vi "Core_Chem_User_Interface_v3.0.vi"() -> ()   [LabVIEW 2014]
uses:
  C:/Program Files (x86)/National Instruments/LabVIEW 2014/examples/Data Communication/Network Streams/Simple Network Streams/support/Network Stream Command.ctl
  <vilib>/dex/Stream Element Allocation Mode.ctl
  <vilib>/Platform/TimedLoop/XDataNode/timing_clust.ctl
  <vilib>/Platform/TimedLoop/XDataNode/nitl_modes.ctl
  <vilib>/Platform/TimedLoop/XDataNode/wakeup.ctl
  <vilib>/Utility/tcp.llb/UDP Multicast Read-Only Open.vi
  <vilib>/platform/TimedLoop/XDataNode/XDataNode.xnode
  <vilib>/Platform/TimedLoop/XDataNode/XDNodeRunTimeDep.lvlib
  <vilib>/FTP/NI_FTP.lvlib
panel:
  out "Network disconnected":bool
  out "cRIO connection status":bool
  out "Network Check error out":errorcluster
  out "SO2 Zeroing (Inflight)\nTime Remain (sec)":u32
  in  "eV6 User set time \n(Inflight) (sec)":i32=120
  in  "SO2 Inflight \nZeroing":bool
  out "Create folder error out 2":errorcluster
  out "Create folder error out":errorcluster
  in  "Confirm Flight Number":bool
  out "PRTAFT_UDP_In":string
  out "TWBOZO01":string
  out "CABOZO01":string
  out "TEIOZO01":string
  out "CHTSOO01":string
  out "CHFGGA01":string
  out "AL52CO01":string
  in  "Flight Number":string
  in  "Tab Control":T1(tab)
  out "FGGA preflight Des 17":string="Preflight - Start minimum 2 hours before take-off\n\n1. Ensure no bags/jackets are stowed on seat backs and behind seats in front of core chemistry rack at all times.\n\n2. Remove inlet covers if applicable.\n\n3. Connect Lilliput mini TFT/LCD VGA cable to FGGA VIDEO (back panel) and PS2 Keyboard/Mouse cables to FGGA Connectors (back panel). TFT/LCD screen kept in WAS/GAS rack Zargers Box. Keyboard/Mouse kept bottom of chemistry rack. (DO NOT disconnect PS2 cable). Connect TFT/LCD AC/DC PSU to 6026-8-98 Amphenol (SSP9) and make 230 Vac CB.\n\n4. Ensure all circuit breakers are pushed in, except 230Vac and 28Vdc, UPS switch off (down) and AL5002 CO Plasma Lamp switch off (down), WoW key to normal (horizontal).\n\n5. Wait for ALL network switches on the aircraft to be up and running before start-up. On the Flight Manager's Interface on the Flight Manager laptop, check SSP icons status (top row) should be all green.  \n\n6. Check AboutTime has synchronised laptop clock to aircraft timeservers (Filiberto/Gaston).\n\nClick the PowerUp Tab."
  out "FGGA preflight Des 16":string="PowerUp\n\n1.\tSSP9 forward face\tMake 3 CBs\n\n2.\tPWRDIST \t\tMake 230Vac CB \n                     Switch UPS On \t[UP]\n                     Make 28Vdc CB\n                     Check 28VDC OK Green Light comes on\n\n3.\tCore Chemistry e-Log\nComplete Core Chemistry e-Log in WordPad (Bnnn_CoreChemLog_v2.2), save on Flight Manager's laptop (192.168.101.180/      flt_folders/Bnnn); Fill in header with date, flight number and your name/initials.\n\n4. Wait for MFM flow rate to display non zero value.\n\n5.\tSAMPUMP\t\t\n - Switch WoW override key (vertical) to check pump starts, and MFM flowrate increase (>20 LPM) on the right hand plot. \n - Switch off WoW override\t\t\t\t [NORM, key horizontal]\n\nClick the 2B Ozone tab if operated, otherwise, click the UDP tab.\n\n\n"
  out "MFM":dbl(graph)
  in  "Ambient = OFF\nCabin = ON":bool
  out "FGGA preflight Des 15":string="2B Ozone Preflight\n\n1.\tSelect either Ambient or Cabin Air mode (default should be OFF for Ambient air mode).\n\n2. Check flowrate is greater than 2000 sccm on the right hand plot.\n\nClick the UDP tab."
  out "2B Ozone concentration":dbl(graph)
  out "2B Ozone flow rate":dbl(graph)
  out "2BOzone Event error out":errorcluster
  out "2BOzone command sender error out":errorcluster
  out "FGGA preflight Des 20":string="4. Check derived parameters in DECADES (192.168.101.110 & 192.168.101.108). 574 Ozone TEi49C; 588 CO AL5002; 611 SO2 TEi43i; 903 - 905 FGGA; 910 / 920 Ozone 2B."
  out "FGGA preflight Des 14":string="UDP Preflight\n1. Check all UDP packets are updating.  Unix time increasing by 1 sec (3rd parameter).\n2. Check flight number is correct.\n3. Confirm flight number and check it appears in the UDP packet (6th parameter). "
  in  "name":string="239.1.4.6"
  in  "Port":u16=50001
  out "FGGA":string
  out "CO":string
  out "TEi49 Ozone":string
  out "2B Cabin Ozone":string
  out "2B Ambient Ozone":string
  out "SO2":string
  in  "Ozone Zeroing Abort":bool
  out "Ozone Zeroing\nTime Remain (sec)":u32
  in  "Ozone Zeroing":bool
  out "TEI49 Sample Flow B":dbl(graph)
  out "TEi49 Concentration":dbl(graph)
  out "TEI49 Sample Flow A":dbl(graph)
  out "FGGA preflight Des 13":string="TEi49 Ozone PRE-FLIGHT - LAST ACTIONS BEFORE SEAT-BELTING DOWN (PRIOR TO ENGINES START)\n\n1. Ozone monitor zeroing\t\t[10 min minimum]\n\n\n2. Check TEi49 zero value and note down value in e-Log. \n"
  out "FGGA preflight Des 12":string="TEi49 Ozone Preflight\n\n1. Check nominal sample flowrate on both channels is ~0.7 LPM."
  out "Ozone Event error out":errorcluster
  out "Ozone command sender error out":errorcluster
  in  "Ozone UDP Time Offset":i32=1
  in  "SO2 Zeroing / Calibration Abort":bool
  out "SO2 react pressure":dbl(graph)
  in  "Prepare SO2 Zero Gas":bool
  in  "Prepare SO2 Span Gas":bool
  in  "Auto Zeroing \ninterval (sec)":i32=600
  out "Next Auto Zero\nStarts in (sec)":u32
  out "Auto Zero\nIndicator":string="Auto Zero Inactive; Manual Zero Allow"
  out "SO2 Resume Zeroing\nCount down timer (sec)":u32
  in  "SO2 Pause\nAuto Zeroing":bool
  out "TEi43i Concentration scaled / raw":cluster{dbl, dbl}(graph)
  in  "SO2 Auto Zeroing":bool
  out "mean zero\ncal status":bool
  out "SO2 Sensitivity":dbl format="%.2g"
  out "SO2 Zero":dbl format="%.2g"
  in  "eV9 Flush User\nset time (sec)":i32=15
  in  "MFC_3 User Set Value":dbl=2.0
  in  "MFC_2 User Set Value":dbl=2.5
  in  "eV6 User\nset time (sec)":i32=600
  out "SO2 Flush\nTime Remain (sec)":u32
  out "TEI43i MFC3 Sample Flow":dbl(graph)
  out "TEI43C Sample Flow":dbl(graph)
  out "TEI43i MFC2 Cal Flow":dbl(graph)
  out "SO2 CAL/Zero\nTime Remain (sec)":u32
  out "SO2 Cal/Zero Flush\nTime Remain (sec)":u32
  in  "SO2 CAL/Zero":bool
  out "FGGA preflight Des 11":string="TEi43 SO2 Inflight Calibration & Zeroing"
  in  "SO2 GND Zeroing":bool
  out "SO2 Zeroing\nTime Remain (sec)":u32
  out "FGGA preflight Des 10":string="TEi43 SO2 PRE-FLIGHT - LAST ACTIONS BEFORE SEAT-BELTING DOWN (PRIOR TO ENGINES START)\n\n1. SO2 monitors zeroing\t\t[10 min minimum]\n\n2. Check TEi43i or TEi43C zero value and note down value in e-Log.\n\n3. Select required SO2 Span/Zero CAL gas at CALDECK front panel using quick connector.\n    For pre- and post-flight SO2 span calibrations select span gas. - Perform SO2 CAL\n    For in-flight SO2 (auto) zeroing, select zero air gas.\n\n4. Enable SO2 auto zeroing (if required) and check zeroing interval. "
  in  "SO2 Flush":bool
  out "FGGA preflight Des 9":string="TEi43 SO2 Preflight\n\n1. Check nominal sample flowrate is 2.0 LPM on the right hand plot.\n\nSO2 calibration gas purge - SO2 calibration cylinder locate at bottom of WAS Gas rack.\n\n2.\n\n\n3. Press SO2 flush button, MFC2 cal flow should increase to 2.5 SLPM.\nMonitor MFC2 flow rate to make sure the reading decreases from 2.5 SLPM to 0.0 SLPM.\nCheck pressure content and delivery gauges also reads zero.\nIf pressure content & delivery gauges do NOT read zero, press SO2 flush button again until they do.\n\n4. Quickly open and close cylinder valve 1.\n\n5. Repeat step 3) to 4) three times.\n\n6. Open cylinder valve 1, system is ready. Note down content pressure in elog.\n\n7."
  in  "eV9 flush User\nset time (sec)":i32=30
  in  "eV8 User\nset time (sec)":i32=60
  out "SO2 Event error out":errorcluster
  out "SO2 command sender \nerror out":errorcluster
  in  "SO2 UDP Time Offset":i32=1
  out "Lamp Temperature":dbl(graph)
  out "CO CAL Status":bool
  in  "CO CAL":bool
  out "FGGA preflight Des 8":string="CO Preflight and Inflight Calibrations\nHold down the CAL button for 2 secs then release, CAL status should then lit up.\nInflight calibration performed on 45 minutes interval or more frequently if lamp temperature > 35.5 degC."
  in  "Prepare Gases":bool
  out "FGGA preflight Des 7":string="AL5002 CO Preflight Checks\n\n1.\n\n2. Start CO Vacuum. NB: If there is problem with the software control, use manual override switch [up] on CALDECK front panel\n\n3. CO Checks - charts on the right hand side\n    Lamp Flow Controller ~ 40 ml/min\n    Monochromator Flow Controller ~ 30 ml/min\n    Fluorescence Cell Pressure ~ 7.5 Torr\n\nIf Lamp/Mono flows are low, manual valves (V1 -> V5) may still be shut, or pressure adjusting valves (ALREG1 & 2) have not been set > 2 bar\n\nIf Cell pressure is 10 Torr (max range), check that COPUMP is running and eV7 is opened (CO Vacuum eV7 is ON).\n\n4. Switch Plasma Lamp at the front panel UP\n\nDetector count rate (on 'Raw Signal' or F2 instrument touchscreen) should increase to >=10000 Hz within a minute.  Recycle plasma lamp switch (off/on) if no significant increase in count rate after 10 mins.  CO concentration should increase (100s ppb). \n     \n\n"
  in  "CO Vaccum (eV7)":bool
  out "Raw Signal":dbl(graph)
  out "CO Concentration":dbl(graph)
  out "Fluorescence Cell Pressure":dbl(graph)
  out "Monochromator Flow":dbl(graph)
  out "Lamp Flow Controller":dbl(graph)
  in  "CO UDP Time Offset":i32=1
  out "CO2 Pressure\nDelivery (PSIA)":dbl(slide) scale=0.0..100.0
  out "Std\nContent (barG)":dbl(slide) scale=0.0..220.0
  out "N2\nContent (barG)":dbl(slide) scale=0.0..220.0
  out "CO2\nContent (barG)":dbl(slide) scale=0.0..170.0
  out "CO Event error out":errorcluster
  out "CO command sender error out":errorcluster
  out "CO Zero":T2(array[cluster])
  out "CO Sensitivity":T3(array[cluster])
  in  "FGGA Calibration Abort":bool
  out "Ring Down Time RDA & RDB":cluster{dbl, dbl}(graph)
  in  "Line Lock Setting Change":bool
  out "Cell temperature":dbl(graph)
  out "Cell pressure":dbl(graph)
  in  "Manual FGGA Pump":bool
  out "CO2":dbl(graph)
  out "CH4":dbl(graph)
  out "H2O":dbl(graph)
  out "WoW Flag":string="0"
  in  "FGGA pump\nsync to WoW":bool
  out "CH4 Dry":dbl(graph)
  out "CO2 Dry":dbl(graph)
  out "MFC1 Cal Flow":dbl(graph)
  out "Flush Target Tank\nTime Remain (sec)":u32
  out "Flush Low Tank\nTime Remain (sec)":u32
  out "Flush High Tank\nTime Remain (sec)":u32
  in  "Flush Target Tank":bool
  in  "Flush Low Tank":bool
  in  "Flush High Tank":bool
  in  "FGGA Restart":bool
  out "FGGA preflight Des 6":string="FGGA Instrument Controls"
  in  "High Cal":bool
  out "High Cal\nFlush Time Remain (sec)":u32
  out "High Cal\nCal Time Remain (sec)":u32
  in  "Low Cal":bool
  in  "Target Cal":bool
  in  "Span Cal - \nHigh Cal, CO Cal, Low Cal":bool
  out "Low Cal\nFlush Time Remain (sec)":u32
  out "Low Cal\nCal Time Remain (sec)":u32
  out "Target Cal\nFlush Time Remain (sec)":u32
  out "Target Cal\nCal Time Remain (sec)":u32
  in  "MFC_1 User Set Value":dbl=2.0
  out "FGGA preflight Des 5":string="FGGA Inflight Calibrations"
  out "FGGA preflight Des 4":string="FGGA Ground Preflight Checks\n\n1. Switch FGGA pump ON\n\n2. Check cavity pressure ~50 Torr\n\n3. Switch FGGA pump OFF\n\n4. Enable FGGA pump sync to WoW\n\n5.. Check Time Synchronisation\n\n6. Check CO2 & CH4 values\n\nIf CO2 & CH4 values are -1 ppm, follow the \nchange linelock settings procedure.\n\n\n\n\n\nLAST ACTION BEFORE SEAT-BELTING \nDOWN (PRIOR TO ENGINES START)\n\n1. Disconnect Monitor & stow away. Leave Keyboard & Mouse connected. Place keyboard at the bottom\nof the rack.\n\n"
  out "FGGA preflight Des 3":string="FGGA CAL Gas Purge\n\nFor each cylinder in gas stowage, check that,\n\n1. V1 Closed\n    V3 Closed\n    V4 Make sure arrow positioned downwards (i.e. flow points to gas line)\n\n2. V3 Open (turn anti-clockwise)\n\n3. Use the button on the right according to the operating cylinder to flush the line. Monitor the MFC flow rate to make sure the reading decreases from 3 to zero. (ie fully flushed). Pressure content & delivery gauges should also read zero.\n\n4. V3 Close (turn clockwise)\n\n5. V1 Open / Close quickly\n         Check delivery pressure gauge is ~ 40 PSI \n         (Use V2 to increase if necessary)\n\n6. Repeat steps 2) to 5) three times\n\n7. V3 Close (turn clockwise)\n\n8. V1 Open, check V2 ~ 40 PSIG\n\n9. V3 Open - System is ready"
  out "FGGA command sender error out":errorcluster
  out "FGGA Event Error out":errorcluster
  in  "FGGA UDP Time Offset":i32=1
  in  "FGGA Shutdown":bool
  in  "Postflight Procedures":bool
  in  "FTP ASCII Files to Local":bool
  in  "Transfer FGGA Files":bool
  out "FGGA preflight Des 18":string="Postflight\n\n1. Press the FTP ASCII File to Local button to transfer ASCII files to flight folder.\n\n\n2. Press the Transfer FGGA Files button to transfer FGGA files to flight folder. \n\n\n3. Shutdown FGGA.\n\n\n4. View Postflight Procedures."
  out "File List":string[](array[string])
  out "FGGA File Transfer Error out":errorcluster
  out "Move to FM Error out":errorcluster
  out "USB Disk Space Used %":dbl(slide) scale=0.0..100.0
  out "PTP Sync":bool
  out "CPU Total %":dbl(graph)
  out "PRTAFT_DLU":string
  in  "Pause Auto Zero Count \nDown set time (sec)":i32=600
  out "Calibration gas cylinder \nconcentration (ppb)":dbl format="%.4g"
  in  "Save Calibration gas\ncylinder concentration to file":bool
  in  "Calibration gas cylinder \nconcentration (ppb)":dbl=500.0 format="%.4g"
  in  "Simulate MOCCA Conc":dbl
  in  "MOCCA window \ndelay time (sec)":i32=30
  in  "MOCCA Limit":i32=800
  in  "SO2 Inflight MOCCA Alarm\n(default = OFF)":bool
  in  "Offset Mean Zero Calculation (default = ON)\nOFF = User input\nOn = Mean zero calculated with ev8":bool=TRUE
  out "FGGA preflight Des 19":string="This tab controls ONLY for advanced operators."
  in  "Inst_alm_thresh":i32=220
  in  "3hr_alm_thresh":i32=80
  in  "Simulate Inst Conc":i32
  in  "Simulate 3hr Average Conc":dbl
  in  "Simulate 2B Conc":bool
  in  "Ozone eV6":bool
  in  "Simulate Conc":bool
  in  "8hr TWA Limit":i32=490
  in  "10mins STEL Limit":i32=800
  in  "SO2 Sensitivity":dbl=1.1
  in  "SO2 Zero":dbl
  in  "Simulate TWA Conc":dbl
  in  "Simulate STEL Conc":dbl
  in  "MFC_3\nSLPM Value":dbl=2.0
  in  "MFC_2\nSLPM Value":dbl
  in  "SO2 eV6":bool
  in  "eV8":bool
  in  "eV9":bool
  in  "eV4":bool
  in  "eV3":bool
  in  "MFC_1\nSLPM Value":dbl
  in  "eV2":bool
  in  "eV1":bool
  in  "cRIO File IO Stop\n(USB Flash Drive Unmount)":bool
  # "Unix time"
  # "Flight Number"
  # "concentration (scaled)\npmt_volt\nlamp_volt\nlamp_intens\ninternal_temper\nreact_temper\nreact_press\nflow\nflags\nten_min_so2\neight_hr_so2\nten_min_so2_alm\neight_hr_so2_alm\nMFC_2absolute_pres\nMFC_2temperature\nMFC_2volumetic_flow\nMFC_2mass_flow\nMFC_2set_point\nMFC_3_absolute_pres\nMFC_3_temperature\nMFC_3volumetic_flow\nMFC_3mass_flow\nMFC_3set_point\nV6\nV8\nV9\nMFC2_Set_Value\nMFC3_Set_Value\nconcentration (raw)\nmean calculation status\noffset\nsensitivity\nev8_user_set_time\nauto_zeroing_control\nev8_zero_interval\nMOCCA_inflight_alarm\nMOCCA_time_window_delay\nMOCCA_SO2_limit\n10 min STEL limit\n8 hour TWA limit\nSO2 cal gas cylin conc\nsimulate_SO2_conc_control\nMOCCA_SO2_sim_value\nMOCCA_SO2_alarm"
  # "Unix time"
  # "Unix time"
  # "Unix time"
  # "Unix time"
  # "Flight Number"
  # "Flight Number"
  # "Flight Number"
  # "Flight Number"
  # "conc\ntemp\npress\nflow\nthreehr_oz\nInst_alarm\nthreehr_alarm"
  # "ch4\nco2\nh2o\npress_torr\ntemp_c\nfit_flag\nrda_usec\nrdb_usec\nch4_dry\nco2_dry\nMFC_1_absolute_pres\nMFC_1_temperature\nMFC_1volumetic_flow\nMFC_1mass_flow\nMFC_1set_point\nV1\nV2\nV3\nV4\nrestart_FGGA\nFGGA_Pump\nCAL_MFC_1Set_Value"
  # "conc\ntemp\npress\nflow"
  # "conc\nbenchtemp\npress\ncellAint\ncellBint\nFlowA\nFlowB\nlamptemp\nflag\nV6"
  # "conc\ncounts\nsens\nzero\nlampflow\nlamptemp\nmonoflow\nmonotemp\nmonopress\ncellpress\ncalpress\ntemppmt\ncalconc\nerr\ncal_counter\nerr_counter\nCO_vacuum_status\nIn_Cal\nALEG1_press_delivery\nALREG1_press_content\nALREG2_press_content\nALREG3_press_content"
  # "TEi43c"
  # "TEi43i"
  # "SO2 CAL / ZERO\nSETTINGS"
  # "FGGA"
  # "2B Ozone"
  # "TEi49C  - Ozone"
  # "TEi43 - SO2"
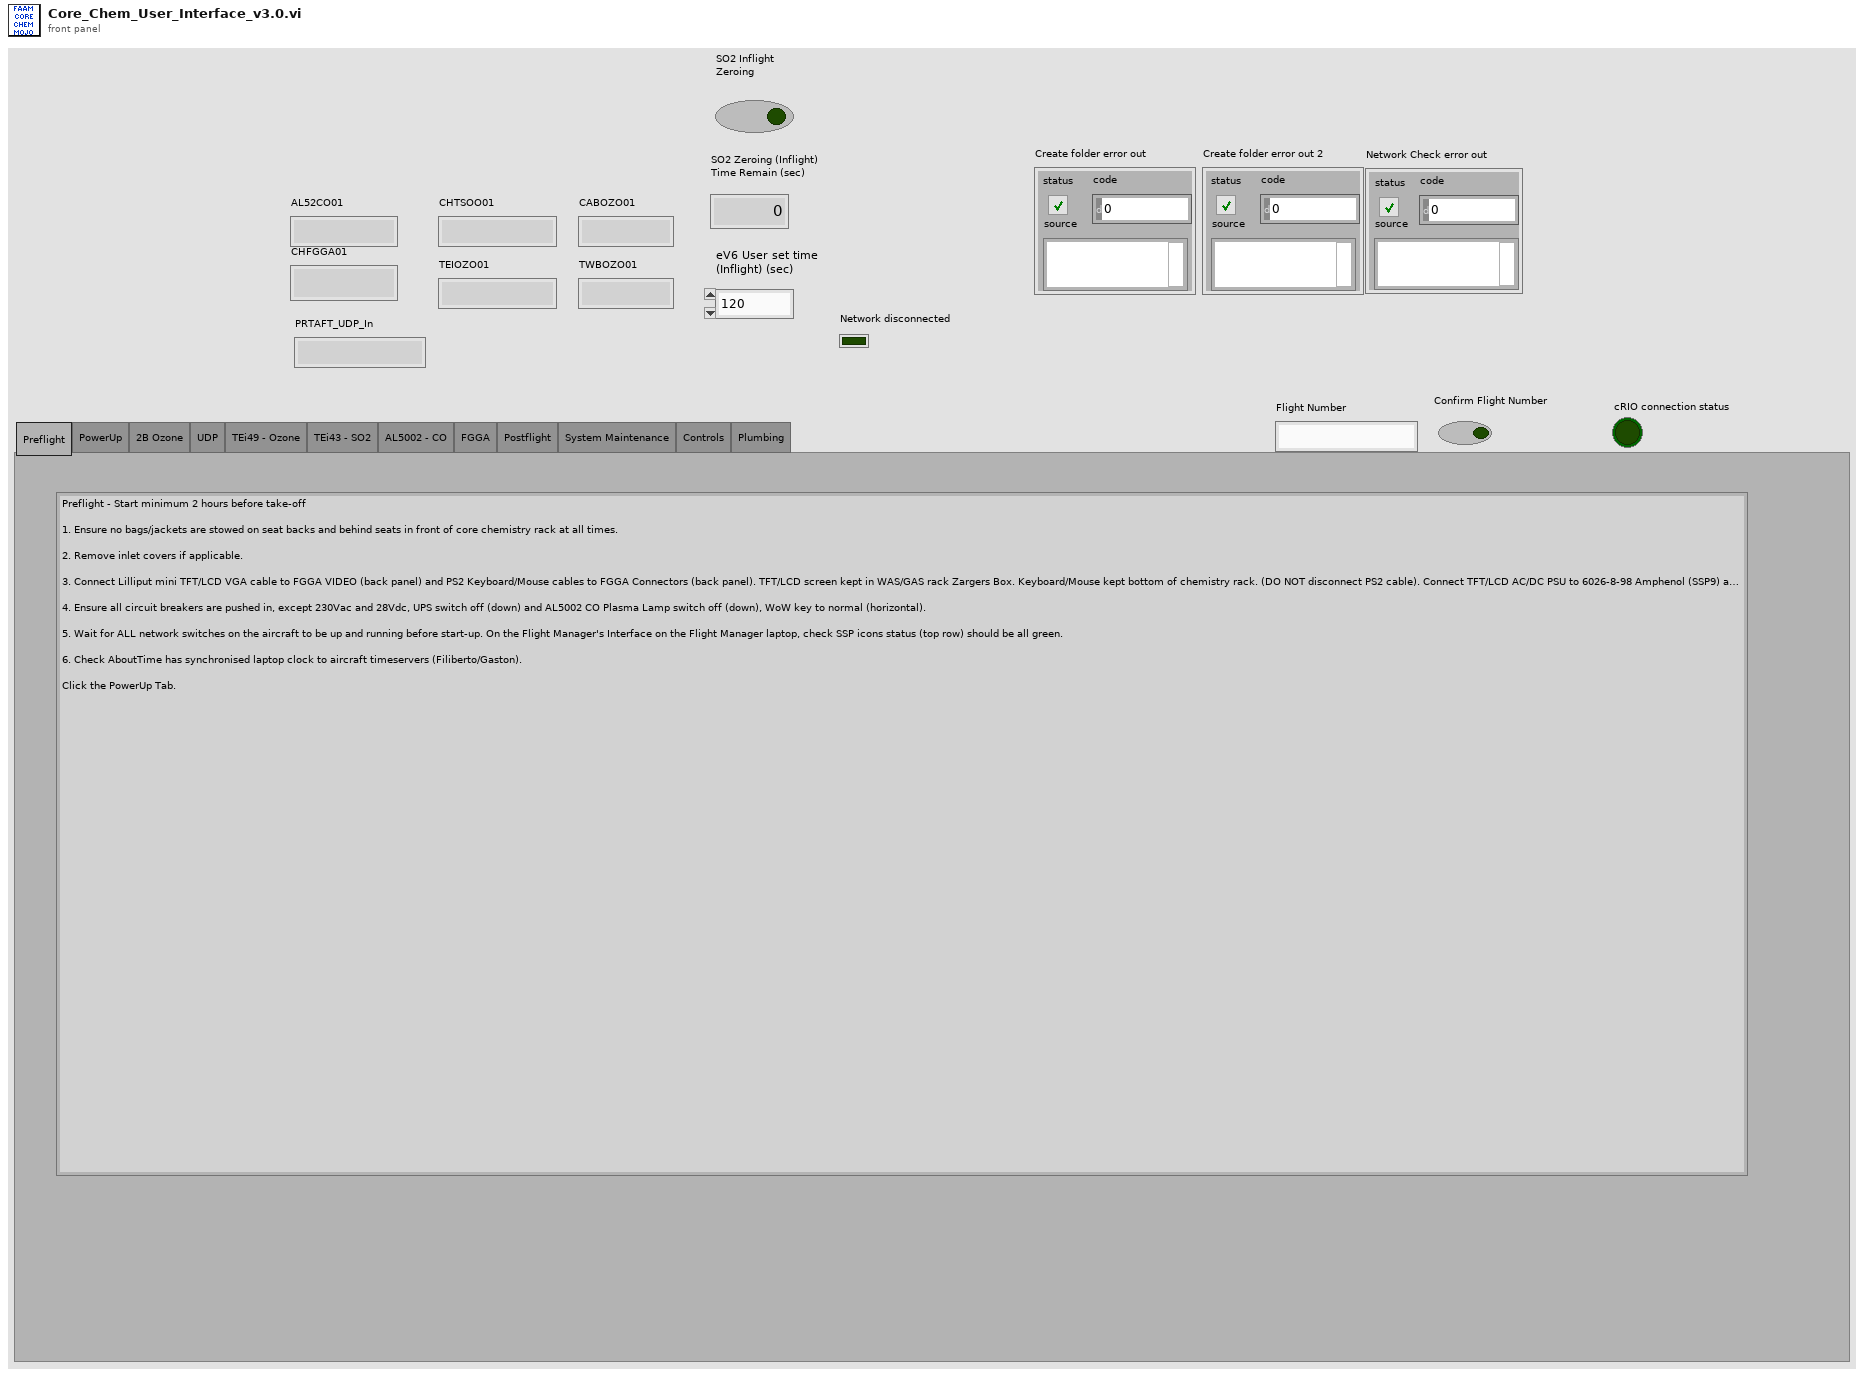
[diagram p1: front panel]
types:
  T1 = enum32{"Preflight", "PowerUp", "2B Ozone", "UDP", "TEi49 - Ozone", "TEi43 - SO2", "AL5002 - CO", "FGGA", "Postflight", "System Maintenance", "Controls", "Plumbing"}
  T2 = cluster{"time stamp":timestamp, "CO Offset":dbl}[]
  T3 = cluster{"time stamp":timestamp, "CO Sensitivity":dbl}[]
  T4 = typedef "Network Stream Command.ctl" = cluster{"Message":string, "Message Data":variant}
  T5 = typedef "Stream Element Allocation Mode.ctl" = u32
  T6 = typedef "XDNodeRunTimeDep.lvlib/timing_clust.ctl" = cluster{"Expected End [f-1]":u64, "Actual End [f-1]":u64, "Finished Late? [f-1]":bool, "Expected End [i-1]":u64, "Actual End [i-1]":u64, "Finished Late? [i-1]":bool, "Expected Start [i]":u64, "Actual Start [i]":u64, "Expected Start [f]":u64, "Actual Start [f]":u64, "Source Name":string, "Structure Name":string, "Period":i64, "Deadline":i64, "Offset":i64, "Start":i64, "Priority":i32, "Timeout":i32, "Mode":T7, "Wakeup Reason":T8, "Error":errorcluster, "Source Type":string, "Secondary Source Type":string, "Global End Time":u64, "Global Start Time":u64, "Frame Duration":u64, "Iteration Duration":u64, "Assigned CPU":i32, "I/O Scan Engine Mode":u32}
  T7 = typedef "XDNodeRunTimeDep.lvlib/nitl_modes.ctl" = enum32{"No Change", "Process missed periods, maintain original phase", "Discard missed periods, maintain original phase", "Process missed periods, ignore original phase", "Discard missed periods, ignore original phase"}
  T8 = typedef "XDNodeRunTimeDep.lvlib/wakeup.ctl" = enum32{"Normal", "Aborted", "Asynchronous wakeup", "Timing source error", "Timed loop error", "Timeout"}
  T9 = typedef "NI_FTP.lvlib/FTP Session.ctl" = refnum<k5>
  T10 = typedef "NI_FTP.lvlib/FTP File Info.ctl" = cluster{"type":enum16{"unknown", "file", "dir", "link"}, "permissions":string, "owner":string, "group":string, "size":i32, "date":string, "name":string, "link name":string}
  T11 = cluster{"Message":string, "Message 2":string, "Message 3":string}
  T12 = cluster{"Message":string, "Message 2":string, "Message 3":string, "Message 4":string}
  T13 = cluster{"Message":string, "Message 3":string, "Message 4":string}
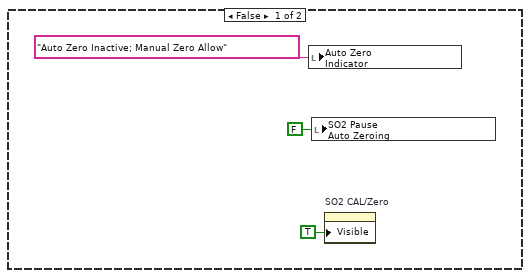
[diagram p5: hidden frame]
diagram:
  w8 = "XXXX"
  w10 = 0
  w11 = 0.0
  w17 = T4 {"Message"="", "Message Data"=variant} ("Message Cluster")
  w23 = T5 0 items=["allocate as needed", "pre-allocate"] ("element allocation mode")
  w29 = T4 {"Message"="", "Message Data"=variant} ("Message Cluster")
  w35 = T5 0 items=["allocate as needed", "pre-allocate"] ("element allocation mode")
  w40 = T4 {"Message"="", "Message Data"=variant} ("Message Cluster")
  w45 = T5 0 items=["allocate as needed", "pre-allocate"] ("element allocation mode")
  w54 = T5 0 items=["allocate as needed", "pre-allocate"] ("element allocation mode")
  w56 = T4 {"Message"="", "Message Data"=variant} ("Message Cluster")
  w63 = T5 0 items=["allocate as needed", "pre-allocate"] ("element allocation mode")
  w65 = T4 {"Message"="", "Message Data"=variant} ("Message Cluster")
  n1 = local write "cRIO File IO Stop\n(USB Flash Drive Unmount)"(FALSE ("Stop File Write")) -> ()
  n2 = local write "Flight Number"(w8) -> ()
  n3 = while {
    shift-right: [w69] -> _
    shift-left: w8 -> [w68]
    stop <- FALSE stop-if-true
    n4 = Not Equal?(x=w68, y="Flight Number") -> (x != y?=w71:bool)
    n5 = case shown="True" w71 {
      tunnel: [w74 w75] -> w69
      tunnel: "Flight Number" -> [_ w75]
      tunnel: w68 -> [w74 _]
      frame False {
      }
      frame True {
        n6 = One Button Dialog(message="Flight Number changed,\nPress flight number button to confirm") -> ()  [unwired: 1 in, 1 out]
      }
    }
    n7 = Wait (ms)(milliseconds to wait=u32 1000) -> ()  [unwired: 1 out]
  }
  n8 = while {
    stop <- FALSE stop-if-true
    # "UDP Read"
    n9 = String To IP(1:"name") -> (0:w82:u32)
    n10 = call-poly <vilib>:"UDP Multicast Open.vi"("multicast addr"=w82, "port"="Port") -> ("error out"=w80:errorcluster, "connection ID"=w79:refnum<k16>)  [unwired: 7 in, 1 out]
    n11 = Wait (ms)(milliseconds to wait=u32 1000) -> ()  [unwired: 1 out]
    n12 = case shown="No Error" w80 {
      selector: w80 -> [w86 _]
      tunnel: w79 -> [w85 _]
      frame No Error {
        w84 = ""
        n13 = while {
          tunnel: w86 -> [w132]
          tunnel: w85 -> [w131]
          shift-right: [w127] -> _
          shift-left: w84 -> [w128]
          shift-right: [w118] -> _
          shift-left: w84 -> [w120]
          shift-right: [w112] -> _
          shift-left: w84 -> [w114]
          shift-right: [w106] -> _
          shift-left: w84 -> [w107]
          shift-right: [w100] -> _
          shift-left: w84 -> [w101]
          shift-right: [w94] -> _
          shift-left: w84 -> [w95]
          shift-right: [w88] -> _
          shift-left: w84 -> [w89]
          stop <- w130 stop-if-true
          n14 = UDP Read(connection ID=w131, 8:w132) -> (data out=w87:string, error out=w130:errorcluster)  [unwired: 2 in, 3 out]
          n15 = Match Pattern(string=w87, regular expression="$TEIOZO") -> (match substring=w126:string, after substring=w125:string)  [unwired: 1 in, 2 out]
          n16 = Match Pattern(string=w87, regular expression="$TWBOZO01,") -> (match substring=w104:string, after substring=w103:string)  [unwired: 1 in, 2 out]
          n17 = Match Pattern(string=w87, regular expression="$CABOZO01,") -> (match substring=w110:string, after substring=w109:string)  [unwired: 1 in, 2 out]
          n18 = Match Pattern(string=w87, regular expression="$CHTSOO") -> (match substring=w98:string, after substring=w97:string)  [unwired: 1 in, 2 out]
          n19 = Match Pattern(string=w87, regular expression="$CHFGGA01,") -> (match substring=w122:string, after substring=w121:string)  [unwired: 1 in, 2 out]
          n20 = Match Pattern(string=w87, regular expression="$AL52CO01,") -> (match substring=w116:string, after substring=w115:string)  [unwired: 1 in, 2 out]
          n21 = Match Pattern(string=w87, regular expression="$PRTAFT01,") -> (match substring=w93:string, after substring=w92:string)  [unwired: 1 in, 2 out]
          n22 = Concatenate Strings(w126, w125) -> (w124:string)
          n23 = Concatenate Strings(w104, w103) -> (w102:string)
          n24 = Concatenate Strings(w110, w109) -> (w108:string)
          n25 = Concatenate Strings(w98, w97) -> (w96:string)
          n26 = Concatenate Strings(w122, w121) -> (w119:string)
          n27 = Concatenate Strings(w116, w115) -> (w113:string)
          n28 = Concatenate Strings(w93, w92) -> (w90:string)
          n29 = Replace Substring(4:w102, 5:w101) -> (1:w100:string)  [unwired: 2 in, 1 out]
          "TWBOZO01" <- w100
          n30 = Replace Substring(4:w124, 5:w128) -> (1:w127:string)  [unwired: 2 in, 1 out]
          "TEIOZO01" <- w127
          n31 = Replace Substring(4:w108, 5:w107) -> (1:w106:string)  [unwired: 2 in, 1 out]
          "CABOZO01" <- w106
          n32 = Replace Substring(4:w96, 5:w95) -> (1:w94:string)  [unwired: 2 in, 1 out]
          "CHTSOO01" <- w94
          n33 = Replace Substring(4:w113, 5:w114) -> (1:w112:string)  [unwired: 2 in, 1 out]
          "AL52CO01" <- w112
          n34 = Replace Substring(4:w119, 5:w120) -> (1:w118:string)  [unwired: 2 in, 1 out]
          "CHFGGA01" <- w118
          n35 = Replace Substring(4:w90, 5:w89) -> (1:w88:string)  [unwired: 2 in, 1 out]
          "PRTAFT_UDP_In" <- w88
        }
      }
      frame Error {
      }
    }
  }
  n36 = Obtain Queue(name (unnamed)="CO_Command", element data type=w65) -> (queue out=w16:refnum<queue>, error out=w59:errorcluster)  [unwired: 3 in, 1 out]
  n37 = Create Network Stream Writer Endpoint(6:w63, 7:10 ("writer buffer size"), 9:w65, 10:"//192.168.101.17/command/reader/CO" ("reader url"), 11:"/command/writer/CO" ("writer name")) -> (0:w62:errorcluster, 3:w61:refnum<k21>)  [unwired: 2 in]
  n38 = while {
    tunnel: w16 -> [w136]
    tunnel: w59 -> [w135]
    tunnel: [w133] -> _
    stop <- FALSE stop-if-true
    # "CO UI Event Handler Loop"
    n39 = event shown="[4] \"Confirm Flight Number\": Value Change" {
      selector: _ -> [_ _ _ _ _]
      dyn-events: _ -> [_ _ _ _ _]
      timeout: _ -> [_ _ _ _ _]
      tunnel: w136 -> [w143 w150 w154 w161 w169]
      tunnel: w135 -> [w142 w149 w153 w160 w168]
      tunnel: [w137 w144 w152 w159 w167] -> w133
      event "CO CAL": Value Change {
        n40 = event-data() -> ("NewVal"=w140:bool)  [unwired: 1 in]
        n41 = Bundle(cluster=T4 {"Message"="", "Message Data"=variant} ("Message Cluster"), "Message"="CO CAL", "Message Data"=w140) -> (w138:T4)
        n42 = Enqueue Element(queue=w143, element=w138, error in (no error)=w142) -> (error out=w137:errorcluster)  [unwired: 1 in, 2 out]
      }
      event "CO UDP Time Offset": Value Change {
        n43 = event-data() -> ("NewVal"=w147:i32)  [unwired: 1 in]
        n44 = Bundle(cluster=T4 {"Message"="", "Message Data"=variant} ("Message Cluster"), "Message"="UDP Time Offset", "Message Data"=w147) -> (w145:T4)
        n45 = Enqueue Element(queue=w150, element=w145, error in (no error)=w149) -> (error out=w144:errorcluster)  [unwired: 1 in, 2 out]
      }
      event "CO Vaccum (eV7)": Value Change {
        n46 = event-data() -> ("NewVal"=w151:bool)  [unwired: 1 in]
        n47 = Bundle(cluster=T4 {"Message"="", "Message Data"=variant} ("Message Cluster"), "Message"="CO Vacuum", "Message Data"=w151) -> (w155:T4)
        n48 = Enqueue Element(queue=w154, element=w155, error in (no error)=w153) -> (error out=w152:errorcluster)  [unwired: 1 in, 2 out]
      }
      event "cRIO File IO Stop\n(USB Flash Drive Unmount)": Value Change {
        n49 = event-data() -> ("NewVal"=w158:bool)  [unwired: 1 in]
        n50 = Bundle(cluster=T4 {"Message"="", "Message Data"=variant} ("Message Cluster"), "Message"="Stop File Write", "Message Data"=w158) -> (w162:T4)
        n51 = Enqueue Element(queue=w161, element=w162, error in (no error)=w160) -> (error out=w159:errorcluster)  [unwired: 1 in, 2 out]
      }
      event "Confirm Flight Number": Value Change {
        n52 = event-data() -> ()  [unwired: 1 in, 1 out]
        n53 = flat-sequence {
          tunnel: w168 -> [w171]
          tunnel: w169 -> [w172]
          tunnel: [w172] -> w166
          tunnel: [w171] -> w165
          tunnel: [w174] -> w167
          tunnel: w166 -> [w176]
          tunnel: w165 -> [w175]
          frame #0 {
            n54 = local write "cRIO File IO Stop\n(USB Flash Drive Unmount)"(FALSE ("cRIO File IO Stop\n(USB Flash Drive Unmount)")) -> ()
          }
          frame #1 {
            n55 = local read "Flight Number"() -> (w173:string)
            n56 = Bundle(cluster=T4 {"Message"="", "Message Data"=variant} ("Message Cluster"), "Message"="Flight Number", "Message Data"=w173) -> (w177:T4)
            n57 = Enqueue Element(queue=w176, element=w177, error in (no error)=w175) -> (error out=w174:errorcluster)  [unwired: 1 in, 2 out]
          }
        }
      }
    }
    "CO Event error out" <- w133
  }
  n58 = while {
    tunnel: w16 -> [w187]
    shift-right: [w182] -> _
    shift-left: w61 -> [w184]
    shift-right: [w180] -> w50
    shift-left: w62 -> [w186]
    tunnel: w59 -> [w181]
    stop <- w180 stop-if-true
    # "CO UI Command Sender"
    n59 = Dequeue Element(queue=w187, error in (no error)=w181) -> (element=w183:T4)  [unwired: 1 in, 3 out]
    n60 = Unbundle By Name(w183) -> ("Message"=w185:string)
    n61 = case shown="\"UDP Time Offset\"" w185 {
      tunnel: w186 -> [w188 w192 w199 w206 w213 w220]
      tunnel: w184 -> [w189 w195 w202 w209 w216 w223]
      tunnel: w183 -> [_ w194 w201 w208 w215 w222]
      tunnel: [w188 w191 w198 w205 w212 w219] -> w180
      tunnel: [w189 w190 w197 w204 w211 w218] -> w182
      frame "False", Default {
      }
      frame "CO CAL" {
        n62 = shared-variable-write(w195, w192, w194) -> (w193:refnum<k21>, w196:errorcluster)  [unwired: 1 in, 1 out]
        n63 = Flush Stream(8:w196, 11:w193) -> (0:w191:errorcluster, 3:w190:refnum<k21>)  [unwired: 2 in, 1 out]
      }
      frame "UDP Time Offset" {
        n64 = shared-variable-write(w202, w199, w201) -> (w200:refnum<k21>, w203:errorcluster)  [unwired: 1 in, 1 out]
        n65 = Flush Stream(8:w203, 11:w200) -> (0:w198:errorcluster, 3:w197:refnum<k21>)  [unwired: 2 in, 1 out]
      }
      frame "Stop File Write" {
        n66 = shared-variable-write(w209, w206, w208) -> (w207:refnum<k21>, w210:errorcluster)  [unwired: 1 in, 1 out]
        n67 = Flush Stream(8:w210, 11:w207) -> (0:w205:errorcluster, 3:w204:refnum<k21>)  [unwired: 2 in, 1 out]
      }
      frame "Flight Number" {
        n68 = shared-variable-write(w216, w213, w215) -> (w214:refnum<k21>, w217:errorcluster)  [unwired: 1 in, 1 out]
        n69 = Flush Stream(8:w217, 11:w214) -> (0:w212:errorcluster, 3:w211:refnum<k21>)  [unwired: 2 in, 1 out]
      }
      frame "CO Vacuum" {
        n70 = shared-variable-write(w223, w220, w222) -> (w221:refnum<k21>, w224:errorcluster)  [unwired: 1 in, 1 out]
        n71 = Flush Stream(8:w224, 11:w221) -> (0:w219:errorcluster, 3:w218:refnum<k21>)  [unwired: 2 in, 1 out]
      }
    }
  }
  "CO command sender error out" <- w50
  n72 = node-c288() -> (w15:T6)  [unwired: 4 in]
  n73 = Initialize Array(cluster{"time stamp":timestamp, "Y":dbl} {"time stamp"=timestamp(0 s since 1904-01-01), "Y"=0.0}, 30 ("dimension size")) -> (w12:cluster{"time stamp":timestamp, "Y":dbl}[])
  n74 = timed-loop {
    timing: w15 -> [_]
    timing-out: [_] -> w14
    stop <- _ stop-if-true
    # "PC Tasks"
    n75 = node-c288() -> ()  [unwired: 1 in, 1 out]
    n76 = event shown="[0] \"FTP ASCII Files to Local\": Value Change" {
      selector: _ -> [_ _ _ _]
      dyn-events: _ -> [_ _ _ _]
      timeout: _ -> [_ _ _ _]
      event "FTP ASCII Files to Local": Value Change {
        n77 = event-data() -> ()  [unwired: 1 in, 1 out]
        n78 = flat-sequence {
          tunnel: [w233] -> w227
          tunnel: [w245] -> w232
          tunnel: [w244] -> w230
          tunnel: [w243] -> w228
          tunnel: w227 -> [w243]
          tunnel: w232 -> [w303]
          tunnel: [w303] -> w231
          tunnel: w230 -> [w299]
          tunnel: [w298] -> w229
          tunnel: w228 -> [w298]
          tunnel: w231 -> [w309]
          tunnel: w229 -> [w304]
          frame #0 {
            n79 = local read "Flight Number"() -> (w235:string)
            n80 = Concatenate Strings("Confirm Flight Number" ("message"), "\n", w235) -> (w239:string)
            n81 = Two Button Dialog(message=w239, 1:"No" ("F button name (\"Cancel\")"), 2:"Yes" ("T button name (\"OK\")")) -> (T button?=w236:bool)
            n82 = case shown="False" w236 {
              tunnel: w235 -> [_ w242]
              tunnel: [w241 w242] -> w233
              frame False {
                n83 = call "Prompt User for Flight Number2"() -> ("Flight Number BXXX"=w241:string)  [unwired: 17 in, 2 out]
              }
              frame True {
              }
            }
          }
          frame #1 {
            n84 = Get Date/Time In Seconds() -> (seconds since 1Jan1904=w249:timestamp)
            n85 = Format Date/Time String(time format string (%c)="%Y%m%d", seconds (now)=w249) -> (date/time string=w247:string)  [unwired: 1 in]
            n86 = call <vilib>:"FTP Open Session.vi"("address"="192.168.101.17") -> ("error out"=w264:errorcluster, "ftp session"=w265:T9)  [unwired: 7 in, 2 out]
            n87 = Concatenate Strings("Use Today's Date" ("message"), "\r", w247) -> (w253:string)
            n88 = call <vilib>:"FTP Logon.vi"("error in (no error)"=w264, "password"="", "user"="anonymous", "ftp session"=w265) -> ("error out"=w261:errorcluster, "ftp session out"=w260:T9)  [unwired: 4 in, 2 out]
            n89 = Two Button Dialog(message=w253, 1:"No" ("F button name (\"Cancel\")"), 2:"Yes" ("T button name (\"OK\")")) -> (T button?=w250:bool)
            n90 = case shown="False" w250 {
              tunnel: [w268 w269] -> w244
              tunnel: w247 -> [_ w269]
              frame False {
                n91 = call "Prompt User for Date"() -> ("Date"=w268:string)  [unwired: 17 in, 2 out]
              }
              frame True {
              }
            }
            n92 = call <vilib>:"FTP Directory Listing.vi"("error in (no error)"=w261, "directory path"="/U:/data", "ftp session"=w260) -> ("dir list"=w259:T10[])  [unwired: 4 in, 4 out]
            n93 = for {
              tunnel: w259 -> [w289] mode=indexing
              tunnel: [w288] -> w256 mode=indexing
              tunnel: w244 -> [w287]
              # "Extract File Name According to the Date"
              n94 = Unbundle By Name(w289) -> ("name"=w295:string, "name"=w294:string)
              n95 = Match Pattern(string=w294, regular expression="_[0-9]+") -> (match substring=w292:string)  [unwired: 1 in, 3 out]
              n96 = String Subset(string=w292, offset (0)=1) -> (substring=w290:string)  [unwired: 1 in]
              n97 = Equal?(x=w290, y=w287) -> (x = y?=w296:bool)
              n98 = case shown="False" w296 {
                tunnel: w295 -> [_ w297]
                tunnel: [_ w297] -> w288
                frame False {
                }
                frame True {
                }
              }
            }
            n99 = Array Size(array=w256) -> (size(s)=w258:i32)
            n100 = for {
              N: w258 -> [_]
              shift-right: [w276] -> w246
              shift-left: w256 -> [w277]
              shift-right: [w274] -> _
              shift-left: 0 -> [w275]
              # "Remove Empty Array"
              n101 = Index Array(array=w277, index=w275) -> (element=w279:string)
              n102 = Equal?(x=w279, y="") -> (x = y?=w278:bool)
              n103 = case shown="True" w278 {
                tunnel: w277 -> [w283 w286]
                tunnel: w275 -> [w282 w284]
                tunnel: [w283 w285] -> w276
                tunnel: [w281 w284] -> w274
                frame False {
                  n104 = Increment(x=w282) -> (x+1=w281:i32)
                }
                frame True {
                  n105 = Delete From Array(array=w286, index=w284) -> (array with subset deleted=w285:string[])  [unwired: 1 in, 1 out]
                }
              }
            }
            "File List" <- w246
            n106 = for {
              tunnel: w246 -> [w272] mode=indexing
              tunnel: [w270] -> w245 mode=indexing
              # "Specify destination path for each file"
              n107 = Concatenate Strings("C:\\temp\\", w272) -> (w271:string)
              n108 = String To Path(string=w271) -> (path=w270:path)
            }
          }
          frame #2 {
            # "FTP a list of files"
            n109 = call <vilib>:"System Exec.vi"("wait until completion? (T)"=TRUE, "working directory"=path "C:/temp", "standard input"=w299, "command line"="C:\\temp\\transfer_ascii_files.bat") -> ()  [unwired: 4 in, 4 out]
          }
          frame #3 {
            # "Move file from local PC to Flight Folder"
            n110 = Build Path(base path=path "\\\\192.168.101.180\\flt_folders" ("path"), name or relative path=w304) -> (appended path=w311:path)
            n111 = Concatenate Strings(w304, "_" ("string"), "corechem" ("string")) -> (w310:string)
            n112 = Build Path(base path=w311, name or relative path=w310) -> (appended path=w306:path)
            n113 = Create Folder(path (use dialog)=w306) -> (created path=w305:path, error out=→"Create folder error out 2":errorcluster)  [unwired: 2 in, 1 out]
            n114 = for {
              tunnel: w305 -> [w318]
              tunnel: [w317] -> w308
              tunnel: w309 -> [w315] mode=indexing
              n115 = Copy(9:TRUE ("overwrite (F)"), 10:w318, 11:w315) -> (0:w317:errorcluster)  [unwired: 2 in, 2 out]
            }
            "Move to FM Error out" <- w308
          }
          frame #4 {
            n116 = local write "FTP ASCII Files to Local"(FALSE ("FTP Files to Local")) -> ()
          }
        }
      }
      event "Transfer FGGA Files": Value Change {
        n117 = event-data() -> ()  [unwired: 1 in, 6 out]
        n118 = flat-sequence {
          tunnel: [w324] -> w323
          tunnel: w323 -> [w336]
          tunnel: [w336] -> w322
          tunnel: [w335] -> w321
          tunnel: [w334] -> w320
          tunnel: w322 -> [w346]
          tunnel: w321 -> [w345]
          tunnel: w320 -> [w347]
          frame #0 {
            n119 = local read "Flight Number"() -> (w325:string)
            n120 = Concatenate Strings("Confirm Flight Number" ("message"), "\n", w325) -> (w327:string)
            n121 = Two Button Dialog(message=w327, 1:"No" ("F button name (\"Cancel\")"), 2:"Yes" ("T button name (\"OK\")")) -> (T button?=w331:bool)
            n122 = case shown="False" w331 {
              tunnel: w325 -> [_ w333]
              tunnel: [w332 w333] -> w324
              frame False {
                n123 = call "Prompt User for Flight Number"() -> ("Flight Number BXXX"=w332:string)  [unwired: 17 in, 2 out]
              }
              frame True {
              }
            }
          }
          frame #1 {
            n124 = Two Button Dialog(message="Get FGGA Files\nof Today's Date?", 1:"No" ("F button name (\"Cancel\")"), 2:"Yes" ("T button name (\"OK\")")) -> (T button?=w340:bool)
            n125 = case shown="False" w340 {
              selector: w340 -> [w342 w343]
              tunnel: [w342 w343] -> w334
              tunnel: [w341 _] -> w335
              frame False {
                n126 = call "Prompt User for Date"() -> ("Date"=w341:string)  [unwired: 17 in, 2 out]
              }
              frame True {
              }
            }
          }
          frame #2 {
            n127 = Build Path(base path=path "\\\\192.168.101.180\\flt_folders" ("path"), name or relative path=w346) -> (appended path=w351:path)
            n128 = Concatenate Strings(w346, "_" ("string"), "corechem" ("string")) -> (w350:string)
            n129 = Build Path(base path=w351, name or relative path=w350) -> (appended path=w344:path)
            n130 = Create Folder(path (use dialog)=w344) -> (error out=→"Create folder error out":errorcluster)  [unwired: 2 in, 2 out]
            n131 = call "labSSH_FGGA_Files_Transfer.vi"("Flight_num"=w346, "Get current?"=w347, "Date"=w345, "Flight Folder Path"=w344) -> ("error IO"=→"FGGA File Transfer Error out":errorcluster)  [unwired: 11 in]
          }
          frame #3 {
            n132 = local write "Transfer FGGA Files"(FALSE) -> ()
          }
        }
      }
      event "FGGA Restart": Value Change {
        n133 = event-data() -> ()  [unwired: 1 in, 6 out]
        n134 = flat-sequence {
          frame #0 {
            n135 = Two Button Dialog(message="FGGA will be restarted,\nARE YOU SURE?") -> (T button?=w357:bool)  [unwired: 2 in]
            n136 = case shown="True" w357 {
              frame False {
              }
              frame True {
                n137 = call "labSSH_Commands.vi"("Data"="reboot") -> ()  [unwired: 14 in, 1 out]
              }
            }
          }
          frame #1 {
            n138 = local write "FGGA Restart"(FALSE ("FGGA Restart")) -> ()
          }
        }
      }
      event "FGGA Shutdown": Value Change {
        n139 = event-data() -> ()  [unwired: 1 in, 6 out]
        n140 = flat-sequence {
          frame #0 {
            n141 = Two Button Dialog(message="FGGA will be shutdown,\nARE YOU SURE?") -> (T button?=w361:bool)  [unwired: 2 in]
            n142 = case shown="True" w361 {
              frame False {
              }
              frame True {
                n143 = call "labSSH_Commands.vi"("Data"="halt") -> ()  [unwired: 14 in, 1 out]
              }
            }
          }
          frame #1 {
            n144 = local write "FGGA Shutdown"(FALSE ("FGGA Restart")) -> ()
          }
        }
      }
    }
    n145 = node-c288() -> ()  [unwired: 1 in, 1 out]
  }
  n146 = local write "Network disconnected"(FALSE ("Network disconnect")) -> ()
  n147 = while {
    shift-right: [w485] -> _
    shift-left: w11 -> [w483]
    shift-right: [w487] -> _
    shift-left: w10 -> [w488]
    shift-right: [w486] -> _
    shift-left: w12 -> [w490]
    shift-right: [w479] -> _
    shift-left: w12 -> [w481]
    shift-right: [w476] -> _
    shift-left: w11 -> [w475]
    shift-right: [w478] -> _
    shift-left: w10 -> [w480]
    stop <- FALSE stop-if-true
    w421 = ""
    w416 = "%s" ("format string")
    w607 = "%s" ("format string")
    w612 = "%s" ("format string")
    w617 = "%s" ("format string")
    w623 = "%s" ("format string")
    w629 = "%s" ("format string")
    w633 = "%s" ("format string")
    # "UDP Data Processing"
    n148 = local read "CHFGGA01"() -> (w636:string)
    n149 = local read "TWBOZO01"() -> (w611:string)
    n150 = local read "AL52CO01"() -> (w628:string)
    n151 = local read "CABOZO01"() -> (w616:string)
    n152 = local read "TEIOZO01"() -> (w622:string)
    n153 = local read "CHTSOO01"() -> (w606:string)
    n154 = local read "Ambient = OFF\nCabin = ON"() -> (w511:bool)
    n155 = Spreadsheet String To Array(delimiter (Tab)=",", format string=w633, spreadsheet string=w636, array type (2D Dbl)=string[] []) -> (array=w583:string[])
    n156 = Spreadsheet String To Array(delimiter (Tab)=",", format string=w629, spreadsheet string=w628, array type (2D Dbl)=string[] []) -> (array=w604:string[])
    n157 = Spreadsheet String To Array(delimiter (Tab)=",", format string=w617, spreadsheet string=w616, array type (2D Dbl)=string[] []) -> (array=w508:string[])
    n158 = Spreadsheet String To Array(delimiter (Tab)=",", format string=w623, spreadsheet string=w622, array type (2D Dbl)=string[] []) -> (array=w581:string[])
    n159 = Spreadsheet String To Array(delimiter (Tab)=",", format string=w612, spreadsheet string=w611, array type (2D Dbl)=string[] []) -> (array=w507:string[])
    n160 = Spreadsheet String To Array(delimiter (Tab)=",", format string=w607, spreadsheet string=w606, array type (2D Dbl)=string[] []) -> (array=w579:string[])
    n161 = Array To Spreadsheet String(delimiter (Tab)="\r", array=w583, 3:w633) -> (spreadsheet string=→"FGGA":string)
    n162 = Array To Spreadsheet String(delimiter (Tab)="\r", array=w604, 3:w629) -> (spreadsheet string=→"CO":string)
    n163 = Array To Spreadsheet String(delimiter (Tab)="\r", array=w508, 3:w617) -> (spreadsheet string=→"2B Cabin Ozone":string)
    n164 = Array To Spreadsheet String(delimiter (Tab)="\r", array=w581, 3:w623) -> (spreadsheet string=→"TEi49 Ozone":string)
    n165 = Array To Spreadsheet String(delimiter (Tab)="\r", array=w507, 3:w612) -> (spreadsheet string=→"2B Ambient Ozone":string)
    n166 = Array To Spreadsheet String(delimiter (Tab)="\r", array=w579, 3:w607) -> (spreadsheet string=→"SO2":string)
    n167 = Select(t=w508, s=w511, f=w507) -> (s? t:f=w506:string[])
    n168 = Index Array(array=w579, index #1=6 ("index"), index #2=4 ("index"), index #3=3 ("index"), index #4=7 ("index"), index #5=8 ("index"), index #6=15 ("index"), index #7=24 ("index"), index #8=29 ("index"), index #9=36 ("index"), index #10=37 ("index"), index #11=38 ("index"), index #12=39 ("index"), index #13=48 ("index"), index #14=14 ("index")) -> (element #1=w498:string, element #2=w562:string, element #3=w557:string, element #4=w550:string, element #5=w526:string, element #6=w525:string, element #7=w439:string, element #8=w438:string, element #9=w387:string, element #10=w383:string, element #11=w379:string, element #12=w377:string, element #13=w369:string, element #14=w367:string)
    n169 = Index Array(array=w506, index #1=8 ("index"), index #2=11 ("index")) -> (element #1=w500:string, element #2=w501:string)
    n170 = Index Array(array=w581, index #1=6 ("index"), index #2=4 ("index"), index #3=3 ("index"), index #4=7 ("index"), index #5=9 ("index"), index #6=14 ("index"), index #7=15 ("index")) -> (element #1=w575:string, element #2=w563:string, element #3=w558:string, element #4=w543:string, element #5=w517:string, element #6=w516:string, element #7=w515:string)
    n171 = Scan Value(string=w500, format string="%f") -> (value=→"2B Ozone concentration":dbl)  [unwired: 1 in, 1 out]
    n172 = Scan Value(string=w501, format string="%4f") -> (value=→"2B Ozone flow rate":dbl)  [unwired: 1 in, 1 out]
    n173 = Index Array(array=w583, index #1=6 ("index"), index #2=4 ("index"), index #3=3 ("index"), index #4=7 ("index"), index #5=8 ("index"), index #6=9 ("index"), index #7=10 ("index"), index #8=17 ("index"), index #9=16 ("index"), index #10=11 ("index"), index #11=12 ("index"), index #12=21 ("index"), index #13=14 ("index"), index #14=15 ("index")) -> (element #1=w577:string, element #2=w565:string, element #3=w560:string, element #4=w545:string, element #5=w463:string, element #6=w460:string, element #7=w455:string, element #8=w453:string, element #9=w450:string, element #10=w445:string, element #11=w444:string, element #12=w431:string, element #13=w397:string, element #14=w396:string)
    n174 = Index Array(array=w604, index #1=2 ("index"), index #2=27 ("index"), index #3=28 ("index"), index #4=29 ("index"), index #5=30 ("index"), index #6=31 ("index"), index #7=6 ("index"), index #8=4 ("index"), index #9=3 ("index"), index #10=8 ("index"), index #11=14 ("index"), index #12=16 ("index"), index #13=19 ("index"), index #14=12 ("index"), index #15=13 ("index"), index #16=10 ("index"), index #17=11 ("index"), index #18=15 ("index")) -> (element #1=w473:string, element #2=w547:string, element #3=w594:string, element #4=w588:string, element #5=w586:string, element #6=w587:string, element #7=w576:string, element #8=w564:string, element #9=w559:string, element #10=w548:string, element #11=w535:string, element #12=w532:string, element #13=w531:string, element #14=w493:string, element #15=w492:string, element #16=w427:string, element #17=w408:string, element #18=w402:string)
    n175 = Scan Value(string=w369, format string="%f") -> (value=→"Calibration gas cylinder \nconcentration (ppb)":dbl)  [unwired: 1 in, 1 out]
    n176 = Scan Value(string=w439, format string="%f") -> (value=→"TEI43i MFC2 Cal Flow":dbl)  [unwired: 1 in, 1 out]
    n177 = Scan Value(string=w438, format string="%f") -> (value=→"TEI43i MFC3 Sample Flow":dbl)  [unwired: 1 in, 1 out]
    n178 = Scan Value(string=w387, format string="%f") -> (value=w373:dbl)  [unwired: 1 in, 1 out]
    n179 = Scan Value(string=w383, format string="%d", default (0 dbl)=0) -> (value=w381:i32)  [unwired: 1 out]
    n180 = Scan Value(string=w367, format string="%f") -> (value=→"SO2 react pressure":dbl)  [unwired: 1 in, 1 out]
    n181 = Scan Value(string=w377, format string="%f") -> (value=→"SO2 Sensitivity":dbl)  [unwired: 1 in, 1 out]
    n182 = Scan Value(string=w379, format string="%f") -> (value=→"SO2 Zero":dbl)  [unwired: 1 in, 1 out]
    n183 = Scan Value(string=w526, format string="%f") -> (value=w374:dbl)  [unwired: 1 in, 1 out]
    n184 = Scan Value(string=w525, format string="%f") -> (value=→"TEI43C Sample Flow":dbl)  [unwired: 1 in, 1 out]
    n185 = Not Equal To 0?(x=w381) -> (x != 0?=→"mean zero\ncal status":bool)
    n186 = Decimal String To Number(string=w473) -> (number=w471:i32)  [unwired: 2 in, 1 out]
    n187 = call "Find_Data_SubVI.vi"("FGGA"=w577, "CO"=w576, "Ozone"=w575, "SO2"=w498) -> ("Output Value"=→"CPU Total %":dbl)  [unwired: 11 in]
    n188 = call "Find_Data_SubVI.vi"("FGGA"=w565, "CO"=w564, "Ozone"=w563, "SO2"=w562) -> ("Output Value"=→"MFM":dbl)  [unwired: 11 in]
    n189 = call "Find_Data_SubVI.vi"("FGGA"=w560, "CO"=w559, "Ozone"=w558, "SO2"=w557) -> ("Output Value"=w556:dbl)  [unwired: 11 in]
    n190 = call "Find_Data_SubVI.vi"("FGGA"=w545, "CO"=w548, "Ozone"=w543, "SO2"=w550) -> ("Output Value"=→"USB Disk Space Used %":dbl)  [unwired: 11 in]
    n191 = Not Equal To 0?(x=w556) -> (x != 0?=→"PTP Sync":bool)
    n192 = Add(x=w471, y=u32 2082844800) -> (x+y=w470:u32)
    n193 = Scan Value(string=w431, format string="%f") -> (value=→"MFC1 Cal Flow":dbl)  [unwired: 1 in, 1 out]
    n194 = Scan Value(string=w397, format string="%f") -> (value=w395:dbl)  [unwired: 1 in, 1 out]
    n195 = Scan Value(string=w396, format string="%f") -> (value=w393:dbl)  [unwired: 1 in, 1 out]
    n196 = Scan Value(string=w444, format string="%f") -> (value=→"Cell temperature":dbl)  [unwired: 1 in, 1 out]
    n197 = Scan Value(string=w445, format string="%f") -> (value=→"Cell pressure":dbl)  [unwired: 1 in, 1 out]
    n198 = Scan Value(string=w450, format string="%f") -> (value=→"CH4 Dry":dbl)  [unwired: 1 in, 1 out]
    n199 = Scan Value(string=w453, format string="%f") -> (value=→"CO2 Dry":dbl)  [unwired: 1 in, 1 out]
    n200 = Scan Value(string=w455, format string="%f") -> (value=→"H2O":dbl)  [unwired: 1 in, 1 out]
    n201 = Scan Value(string=w460, format string="%f") -> (value=→"CO2":dbl)  [unwired: 1 in, 1 out]
    n202 = Scan Value(string=w463, format string="%f") -> (value=→"CH4":dbl)  [unwired: 1 in, 1 out]
    n203 = local read "PRTAFT_UDP_In"() -> (w414:string)
    n204 = Scan Value(string=w587, format string="%f") -> (value=→"Std\nContent (barG)":dbl)  [unwired: 1 in, 1 out]
    n205 = Scan Value(string=w547, format string="%d", default (0 dbl)=u32 0) -> (value=w601:u32)  [unwired: 1 out]
    n206 = Scan Value(string=w586, format string="%f") -> (value=→"N2\nContent (barG)":dbl)  [unwired: 1 in, 1 out]
    n207 = Scan Value(string=w588, format string="%f") -> (value=→"CO2\nContent (barG)":dbl)  [unwired: 1 in, 1 out]
    n208 = Scan Value(string=w594, format string="%f") -> (value=→"CO2 Pressure\nDelivery (PSIA)":dbl)  [unwired: 1 in, 1 out]
    n209 = Bundle(w374, w373) -> (→"TEi43i Concentration scaled / raw":cluster{dbl, dbl})  [unwired: 1 in]
    n210 = To Time Stamp(1:w470) -> (0:w474:timestamp)
    n211 = Scan Value(string=w535, format string="%f") -> (value=→"Lamp Flow Controller":dbl)  [unwired: 1 in, 1 out]
    n212 = Scan Value(string=w408, format string="%f") -> (value=→"Raw Signal":dbl)  [unwired: 1 in, 1 out]
    n213 = Scan Value(string=w402, format string="%f") -> (value=→"Lamp Temperature":dbl)  [unwired: 1 in, 1 out]
    n214 = Scan Value(string=w427, format string="%f") -> (value=→"CO Concentration":dbl)  [unwired: 1 in, 1 out]
    n215 = Scan Value(string=w532, format string="%f") -> (value=→"Monochromator Flow":dbl)  [unwired: 1 in, 1 out]
    n216 = Scan Value(string=w531, format string="%f") -> (value=→"Fluorescence Cell Pressure":dbl)  [unwired: 1 in, 1 out]
    n217 = Not Equal To 0?(x=w601) -> (x != 0?=→"CO CAL Status":bool)
    n218 = Scan Value(string=w515, format string="%f") -> (value=→"TEI49 Sample Flow B":dbl)  [unwired: 1 in, 1 out]
    n219 = Scan Value(string=w517, format string="%f") -> (value=→"TEi49 Concentration":dbl)  [unwired: 1 in, 1 out]
    n220 = Scan Value(string=w516, format string="%f") -> (value=→"TEI49 Sample Flow A":dbl)  [unwired: 1 in, 1 out]
    n221 = Scan Value(string=w493, format string="%f") -> (value=w484:dbl)  [unwired: 1 in, 1 out]
    n222 = Scan Value(string=w492, format string="%f") -> (value=w477:dbl)  [unwired: 1 in, 1 out]
    n223 = Not Equal?(x=w483, y=w484) -> (x != y?=w489:bool)
    n224 = Not Equal?(x=w475, y=w477) -> (x != y?=w482:bool)
    n225 = Spreadsheet String To Array(delimiter (Tab)=",", format string=w416, spreadsheet string=w414, array type (2D Dbl)=string[] []) -> (array=w415:string[])
    n226 = case shown="True" w489 {
      tunnel: w490 -> [w657 w666]
      tunnel: w488 -> [w658 w665]
      tunnel: [w658 w664] -> w487
      tunnel: w474 -> [_ w660]
      tunnel: w484 -> [_ w661]
      tunnel: [w657 w663] -> w486
      tunnel: [w656 w662] -> w485
      tunnel: w484 -> [_ w662]
      tunnel: w483 -> [w656 _]
      frame False {
      }
      frame True {
        n227 = Bundle(w660, w661) -> (w659:cluster{timestamp, dbl})  [unwired: 1 in]
        n228 = Replace Array Subset(array=w666, new element=w659, index=w665) -> (w663:cluster{"time stamp":timestamp, "Y":dbl}[])
        n229 = Increment(x=w665) -> (x+1=w664:i32)
      }
    }
    "CO Sensitivity" <- w486
    n230 = case shown="True" w482 {
      tunnel: w481 -> [w646 w655]
      tunnel: w480 -> [w647 w654]
      tunnel: [w647 w653] -> w478
      tunnel: w474 -> [_ w652]
      tunnel: w477 -> [_ w651]
      tunnel: [w646 w650] -> w479
      tunnel: [w645 w649] -> w476
      tunnel: w477 -> [_ w649]
      tunnel: w475 -> [w645 _]
      frame False {
      }
      frame True {
        n231 = Bundle(w652, w651) -> (w648:cluster{timestamp, dbl})  [unwired: 1 in]
        n232 = Replace Array Subset(array=w655, new element=w648, index=w654) -> (w650:cluster{"time stamp":timestamp, "Y":dbl}[])
        n233 = Increment(x=w654) -> (x+1=w653:i32)
      }
    }
    "CO Zero" <- w479
    n234 = Array To Spreadsheet String(delimiter (Tab)="\r", array=w415, 3:w416) -> (spreadsheet string=→"PRTAFT_DLU":string)
    n235 = Index Array(array=w415, index #1=5 ("index"), index #2=19 ("index")) -> (element #1=w419:string, element #2=w417:string)
    n236 = Not Equal?(x=w419, y=w421) -> (x != y?=w420:bool)
    n237 = Not Equal?(x=w417, y=w421) -> (x != y?=w418:bool)
    n238 = Bundle(w395, w393) -> (→"Ring Down Time RDA & RDB":cluster{dbl, dbl})  [unwired: 1 in]
    n239 = case shown="False" w418 {
      tunnel: ["1" w642] -> w411
      tunnel: w417 -> [_ w642]
      frame False {
      }
      frame True {
      }
    }
    n240 = case shown="False" w420 {
      tunnel: ["XXXX" w644] -> w412
      tunnel: w419 -> [_ w644]
      frame False {
      }
      frame True {
      }
    }
    n241 = Wait (ms)(milliseconds to wait=u32 1000) -> ()  [unwired: 1 out]
    n242 = local write "WoW Flag"(w411) -> ()
    n243 = local write "Flight Number"(w412) -> ()
  }
  n244 = while {
    stop <- FALSE stop-if-true
    # "Check Connection with the cRIO continuously"
    n245 = node-c288() -> (w668:T6)  [unwired: 4 in]
    n246 = TCP Open Connection(address="192.168.101.17", remote port or service name=u16 7001) -> (connection ID=w677:refnum<k5>, error out=w678:errorcluster)  [unwired: 3 in]
    n247 = timed-loop {
      tunnel: w678 -> [w693]
      tunnel: w677 -> [w690]
      tunnel: [w686] -> w670
      tunnel: [w687] -> w674
      shift-right: [w682] -> _
      shift-left: FALSE -> [w683]
      timing: w668 -> [_]
      timing-out: [_] -> w667
      stop <- w686 stop-if-true
      # "Maintain live connecton to cRIO for connection watchdog"
      n248 = node-c288() -> ()  [unwired: 1 in, 1 out]
      n249 = TCP Write(connection ID=w690, data in="1", error in (no error)=w693, 9:2000 ("timeout ms (25000)")) -> (connection ID out=w691:refnum<k5>, bytes written=w688:i32, error out=w692:errorcluster)
      n250 = Select(t=FALSE, s=w683, f=TRUE) -> (s? t:f=w682:bool)
      "cRIO connection status" <- w682
      n251 = local write "Network disconnected"(FALSE ("Network disconnect")) -> ()
      n252 = TCP Read(connection ID=w691, bytes to read=w688, error in (no error)=w692, 9:2000 ("timeout ms (25000)")) -> (connection ID out=w687:refnum<k5>, error out=w686:errorcluster)  [unwired: 1 in, 1 out]
      n253 = node-c288() -> ()  [unwired: 1 in, 1 out]
    }
    n254 = node-c288(w667) -> ()  [unwired: 1 out]
    n255 = TCP Close Connection(connection ID=w674, error in (no error)=w670) -> (error out=w669:errorcluster)  [unwired: 1 in, 1 out]
    "Network Check error out" <- w669
    n256 = Unbundle By Name(w669) -> ("status"=w671:bool)
    "Network disconnected" <- w671
    n257 = case shown="True" w671 {
      frame False {
      }
      frame True {
        n258 = One Button Dialog(message="Connection to cRIO lost\nAll Calibration(s) will be terminated") -> ()  [unwired: 1 in, 1 out]
      }
    }
  }
  n259 = while {
    stop <- FALSE stop-if-true
    # "Preflight Sub VI Descriptions"
    n260 = Wait (ms)(milliseconds to wait=u32 500) -> ()  [unwired: 1 out]
    n261 = case shown="True" "Line Lock Setting Change" {
      frame False {
      }
      frame True {
        n262 = call "FGGA Linelock Settings Procedures.vi"() -> ()  [unwired: 12 in]
      }
    }
  }
  n263 = while {
    stop <- FALSE stop-if-true
    # "Postflight Sub VI Descriptions"
    n264 = case shown="True" "Postflight Procedures" {
      frame False {
      }
      frame True {
        n265 = call "PostFlight Procedures.vi"() -> ()  [unwired: 12 in]
      }
    }
    n266 = Wait (ms)(milliseconds to wait=u32 500) -> ()  [unwired: 1 out]
  }
  n267 = while {
    stop <- FALSE stop-if-true
    # "Preflight Sub VI Descriptions"
    n268 = case shown="True" "Prepare Gases" {
      frame False {
      }
      frame True {
        n269 = call "CO Gas Preparation.vi"() -> ()  [unwired: 12 in]
      }
    }
    n270 = Wait (ms)(milliseconds to wait=u32 500) -> ()  [unwired: 1 out]
  }
  n271 = while {
    stop <- FALSE stop-if-true
    # "Preflight Sub VI Descriptions"
    n272 = case shown="True" "Prepare SO2 Span Gas" {
      frame False {
      }
      frame True {
        n273 = call "SO2 Span Gas Preparation.vi"() -> ()  [unwired: 12 in]
      }
    }
    n274 = Wait (ms)(milliseconds to wait=u32 500) -> ()  [unwired: 1 out]
  }
  n275 = while {
    stop <- FALSE stop-if-true
    # "Preflight Sub VI Descriptions"
    n276 = case shown="True" "Prepare SO2 Zero Gas" {
      frame False {
      }
      frame True {
        n277 = call "SO2 ZeroAir Gas Preparation.vi"() -> ()  [unwired: 12 in]
      }
    }
    n278 = Wait (ms)(milliseconds to wait=u32 500) -> ()  [unwired: 1 out]
  }
  n279 = Obtain Queue(name (unnamed)="FGGA_Command", element data type=w56) -> (queue out=w6:refnum<queue>, error out=w5:errorcluster)  [unwired: 3 in, 1 out]
  n280 = while {
    shift-right: [w717] -> _
    shift-left: u8 1 -> [w718]
    tunnel: w6 -> [w715]
    tunnel: w5 -> [w714]
    stop <- FALSE stop-if-true
    # "FGGA pump synchronise to WoW Wait on Wheel Flag"
    n281 = Wait (ms)(milliseconds to wait=u32 1000) -> ()  [unwired: 1 out]
    n282 = case shown="True" "FGGA pump\nsync to WoW" {
      tunnel: [w721 w726] -> w717
      tunnel: w718 -> [w721 w725]
      tunnel: w715 -> [_ w724]
      tunnel: w714 -> [_ w723]
      frame False {
      }
      frame True {
        n283 = local read "WoW Flag"() -> (w722:string)
        n284 = Scan Value(string=w722, format string="%d", default (0 dbl)=u8 0) -> (value=w726:u8)  [unwired: 1 out]
        n285 = Not Equal?(x=w726, y=w725) -> (x != y?=w729:bool)
        n286 = case shown="True" w729 {
          tunnel: w726 -> [_ w732]
          tunnel: w724 -> [_ w731]
          tunnel: w723 -> [_ w730]
          frame False {
          }
          frame True {
            n287 = Equal?(x=w732, y=u8 0) -> (x = y?=w737:bool)
            n288 = case shown="True" w737 {
              selector: w737 -> [w739 w740]
              tunnel: [w739 w740] -> w733
              frame False {
              }
              frame True {
              }
            }
            n289 = local write "Manual FGGA Pump"(w733) -> ()
            n290 = Bundle(cluster=T4 {"Message"="", "Message Data"=variant} ("Message Cluster"), "Message"="FGGA_pump", "Message Data"=w733) -> (w734:T4)
            n291 = Enqueue Element(queue=w731, element=w734, error in (no error)=w730) -> ()  [unwired: 1 in, 3 out]
          }
        }
      }
    }
  }
  n292 = while {
    tunnel: w6 -> [w742]
    tunnel: w5 -> [w741]
    tunnel: [w744] -> _
    tunnel: w16 -> [w743]
    stop <- FALSE stop-if-true
    # "FGGA UI Event Handler Loop"
    n293 = event shown="[9] \"Span Cal -  High Cal, CO Cal, Low Cal\": Value Change" {
      selector: _ -> [_ _ _ _ _ _ _ _ _ _ _ _ _ _ _ _ _]
      dyn-events: _ -> [_ _ _ _ _ _ _ _ _ _ _ _ _ _ _ _ _]
      timeout: _ -> [_ _ _ _ _ _ _ _ _ _ _ _ _ _ _ _ _]
      tunnel: w742 -> [w752 w756 w763 w770 w777 w785 w799 w806 w821 w962 w1213 w1283 w1353 w1409 w1523 w1622 w1629]
      tunnel: w741 -> [w751 w755 w762 w769 w776 w784 w798 w805 w820 w961 w1212 w1282 w1352 w1408 w1522 w1621 w1628]
      tunnel: [w746 w754 w761 w768 w775 w783 w797 w804 w811 w935 w1205 w1275 w1345 w1399 w1515 w1620 w1627] -> w744
      tunnel: w743 -> [_ _ _ _ _ _ _ _ _ w949 _ _ _ _ _ _ _]
      event "eV1": Value Change {
        n294 = event-data() -> ("NewVal"=w749:bool)  [unwired: 1 in]
        n295 = Bundle(cluster=T4 {"Message"="", "Message Data"=variant} ("Message Cluster"), "Message"="V1", "Message Data"=w749) -> (w747:T4)
        n296 = Enqueue Element(queue=w752, element=w747, error in (no error)=w751) -> (error out=w746:errorcluster)  [unwired: 1 in, 2 out]
      }
      event "eV2": Value Change {
        n297 = event-data() -> ("NewVal"=w753:bool)  [unwired: 1 in]
        n298 = Bundle(cluster=T4 {"Message"="", "Message Data"=variant} ("Message Cluster"), "Message"="V2", "Message Data"=w753) -> (w757:T4)
        n299 = Enqueue Element(queue=w756, element=w757, error in (no error)=w755) -> (error out=w754:errorcluster)  [unwired: 1 in, 2 out]
      }
      event "eV3": Value Change {
        n300 = event-data() -> ("NewVal"=w760:bool)  [unwired: 1 in]
        n301 = Bundle(cluster=T4 {"Message"="", "Message Data"=variant} ("Message Cluster"), "Message"="V3", "Message Data"=w760) -> (w764:T4)
        n302 = Enqueue Element(queue=w763, element=w764, error in (no error)=w762) -> (error out=w761:errorcluster)  [unwired: 1 in, 2 out]
      }
      event "eV4": Value Change {
        n303 = event-data() -> ("NewVal"=w767:bool)  [unwired: 1 in]
        n304 = Bundle(cluster=T4 {"Message"="", "Message Data"=variant} ("Message Cluster"), "Message"="V4", "Message Data"=w767) -> (w771:T4)
        n305 = Enqueue Element(queue=w770, element=w771, error in (no error)=w769) -> (error out=w768:errorcluster)  [unwired: 1 in, 2 out]
      }
      event "Manual FGGA Pump": Value Change {
        n306 = event-data() -> ("NewVal"=w774:bool)  [unwired: 1 in]
        n307 = Bundle(cluster=T4 {"Message"="", "Message Data"=variant} ("Message Cluster"), "Message"="FGGA_pump", "Message Data"=w774) -> (w778:T4)
        n308 = Enqueue Element(queue=w777, element=w778, error in (no error)=w776) -> (error out=w775:errorcluster)  [unwired: 1 in, 2 out]
      }
      event "Confirm Flight Number": Value Change {
        n309 = event-data() -> ()  [unwired: 1 in, 6 out]
        n310 = flat-sequence {
          tunnel: w784 -> [w787]
          tunnel: w785 -> [w788]
          tunnel: [w788] -> w782
          tunnel: [w787] -> w781
          tunnel: [w790] -> w783
          tunnel: w782 -> [w792]
          tunnel: w781 -> [w791]
          frame #0 {
            n311 = local write "cRIO File IO Stop\n(USB Flash Drive Unmount)"(FALSE ("cRIO File IO Stop\n(USB Flash Drive Unmount)")) -> ()
          }
          frame #1 {
            n312 = local read "Flight Number"() -> (w789:string)
            n313 = Bundle(cluster=T4 {"Message"="", "Message Data"=variant} ("Message Cluster"), "Message"="Flight Number", "Message Data"=w789) -> (w793:T4)
            n314 = Enqueue Element(queue=w792, element=w793, error in (no error)=w791) -> (error out=w790:errorcluster)  [unwired: 1 in, 2 out]
          }
        }
      }
      event "FGGA Restart": Value Change {
        n315 = event-data() -> ("NewVal"=w796:bool)  [unwired: 1 in]
        n316 = Bundle(cluster=T4 {"Message"="", "Message Data"=variant} ("Message Cluster"), "Message"="FGGA_restart", "Message Data"=w796) -> (w800:T4)
        n317 = Enqueue Element(queue=w799, element=w800, error in (no error)=w798) -> (error out=w797:errorcluster)  [unwired: 1 in, 2 out]
      }
      event "cRIO File IO Stop\n(USB Flash Drive Unmount)": Value Change {
        n318 = event-data() -> ("NewVal"=w803:bool)  [unwired: 1 in]
        n319 = Bundle(cluster=T4 {"Message"="", "Message Data"=variant} ("Message Cluster"), "Message"="Stop File Write", "Message Data"=w803) -> (w807:T4)
        n320 = Enqueue Element(queue=w806, element=w807, error in (no error)=w805) -> (error out=w804:errorcluster)  [unwired: 1 in, 2 out]
      }
      event "High Cal": Value Change {
        n321 = event-data() -> ()  [unwired: 1 in, 1 out]
        n322 = flat-sequence {
          tunnel: w821 -> [w826]
          tunnel: w820 -> [w825]
          tunnel: [w824] -> w819
          tunnel: [w823] -> w818
          tunnel: w819 -> [w842]
          tunnel: w818 -> [w841]
          tunnel: [w839] -> w817
          tunnel: [w838] -> w816
          tunnel: [w846] -> w815
          tunnel: [w847] -> w814
          tunnel: w816 -> [w851]
          tunnel: w817 -> [w850]
          tunnel: w815 -> [w904]
          tunnel: w814 -> [w903]
          tunnel: [w901] -> w813
          tunnel: [w900] -> w812
          tunnel: w813 -> [w918]
          tunnel: w812 -> [w917]
          tunnel: [w915] -> w810
          tunnel: [w923] -> w811
          tunnel: w810 -> [w923]
          frame #0 {
            w822 = TRUE
            n323 = Cluster To Array(cluster=T11 {"Message"="V2", "Message 2"="V3", "Message 3"="V4"}) -> (array=w827:string[])
            n324 = for {
              tunnel: w827 -> [w834] mode=indexing
              tunnel: w826 -> [w833]
              tunnel: w825 -> [w832]
              tunnel: [w831] -> w824
              tunnel: [w830] -> w823
              tunnel: w822 -> [w829]
              n325 = Bundle(cluster=T4 {"Message"="", "Message Data"=variant} ("Message Cluster"), "Message"=w834, "Message Data"=w829) -> (w836:T4)
              n326 = Enqueue Element(queue=w833, element=w836, error in (no error)=w832) -> (queue out=w831:refnum<queue>, error out=w830:errorcluster)  [unwired: 1 in, 1 out]
            }
            n327 = local write "eV2"(w822) -> ()
            n328 = local write "eV4"(w822) -> ()
            n329 = local write "eV3"(w822) -> ()
          }
          frame #1 {
            n330 = local read "MFC_1 User Set Value"() -> (w837:dbl)
            n331 = local write "MFC_1\nSLPM Value"(w837) -> ()
            n332 = Bundle(cluster=T4 {"Message"="", "Message Data"=variant} ("Message Cluster"), "Message"="MFC_1", "Message Data"=w837) -> (w840:T4)
            n333 = Enqueue Element(queue=w842, element=w840, error in (no error)=w841) -> (queue out=w839:refnum<queue>, error out=w838:errorcluster)  [unwired: 1 in, 1 out]
          }
          frame #2 {
            n334 = for {
              N: 45 -> [w894]
              tunnel: w851 -> [w884]
              tunnel: w850 -> [w885]
              tunnel: [w885] -> w849
              tunnel: [w884] -> w848
              tunnel: [w883] -> w845
              i -> [w893]
              stop <- w883 stop-if-true
              n335 = Subtract(x=w894, y=w893) -> (x-y=w892:i32)
              n336 = Decrement(x=w892) -> (x-1=w891:i32)
              n337 = local read "FGGA Calibration Abort"() -> (w888:bool)
              n338 = case shown="True" w888 {
                selector: w888 -> [w897 _]
                tunnel: [w897 w898] -> w886
                frame False {
                }
                frame True {
                  n339 = Two Button Dialog(message="Are you sure to abort FGGA High Cal?") -> (T button?=w898:bool)  [unwired: 2 in]
                }
              }
              n340 = Wait (ms)(milliseconds to wait=u32 1000) -> ()  [unwired: 1 out]
              n341 = local read "Network disconnected"() -> (w887:bool)
              n342 = Or(x=w887, y=w886) -> (x .or. y?=w883:bool)
              n343 = case shown="False" w886 {
                selector: w886 -> [w896 _]
                frame False {
                  n344 = local write "FGGA Calibration Abort"(w896) -> ()
                }
                frame True {
                }
              }
              n345 = Select(t=0, s=w883, f=w891) -> (s? t:f=→"High Cal\nFlush Time Remain (sec)":i32)
            }
            n346 = case shown="False" w845 {
              tunnel: w849 -> [w858 w882]
              tunnel: w848 -> [w857 w881]
              tunnel: [w854 w881] -> w847
              tunnel: [w853 w882] -> w846
              frame False {
                w859 = TRUE
                # "Carry on if connection to cRIO is made\nor calibration not abort"
                n347 = Bundle(cluster=T4 {"Message"="", "Message Data"=variant} ("Message Cluster"), "Message"="V1", "Message Data"=w859) -> (w860:T4)
                n348 = local write "eV1"(w859) -> ()
                n349 = Enqueue Element(queue=w858, element=w860, error in (no error)=w857) -> (queue out=w855:refnum<queue>, error out=w856:errorcluster)  [unwired: 1 in, 1 out]
                n350 = for {
                  N: 60 -> [w875]
                  tunnel: w856 -> [w865]
                  tunnel: w855 -> [w864]
                  tunnel: [w865] -> w854
                  tunnel: [w864] -> w853
                  i -> [w874]
                  stop <- w866 stop-if-true
                  n351 = local read "FGGA Calibration Abort"() -> (w869:bool)
                  n352 = Subtract(x=w875, y=w874) -> (x-y=w873:i32)
                  n353 = case shown="True" w869 {
                    selector: w869 -> [w878 _]
                    tunnel: [w878 w879] -> w867
                    frame False {
                    }
                    frame True {
                      n354 = Two Button Dialog(message="Are you sure to abort FGGA High Cal?") -> (T button?=w879:bool)  [unwired: 2 in]
                    }
                  }
                  n355 = local read "Network disconnected"() -> (w868:bool)
                  n356 = Wait (ms)(milliseconds to wait=u32 1000) -> ()  [unwired: 1 out]
                  n357 = Decrement(x=w873) -> (x-1=w870:i32)
                  n358 = Or(x=w868, y=w867) -> (x .or. y?=w866:bool)
                  n359 = case shown="False" w867 {
                    selector: w867 -> [w877 _]
                    frame False {
                      n360 = local write "FGGA Calibration Abort"(w877) -> ()
                    }
                    frame True {
                    }
                  }
                  n361 = Select(t=0, s=w866, f=w870) -> (s? t:f=→"High Cal\nCal Time Remain (sec)":i32)
                }
              }
              frame True {
              }
            }
          }
          frame #3 {
            w902 = FALSE
            n362 = Cluster To Array(cluster=T12 {"Message"="V2", "Message 2"="V3", "Message 3"="V4", "Message 4"="V1"}) -> (array=w905:string[])
            n363 = for {
              tunnel: w905 -> [w912] mode=indexing
              tunnel: [w911] -> w901
              tunnel: [w910] -> w900
              tunnel: w902 -> [w909]
              tunnel: w904 -> [w908]
              tunnel: w903 -> [w907]
              n364 = Bundle(cluster=T4 {"Message"="", "Message Data"=variant} ("Message Cluster"), "Message"=w912, "Message Data"=w909) -> (w914:T4)
              n365 = Enqueue Element(queue=w908, element=w914, error in (no error)=w907) -> (queue out=w911:refnum<queue>, error out=w910:errorcluster)  [unwired: 1 in, 1 out]
            }
            n366 = local write "eV2"(w902) -> ()
            n367 = local write "eV4"(w902) -> ()
            n368 = local write "eV3"(w902) -> ()
            n369 = local write "eV1"(w902) -> ()
          }
          frame #4 {
            w916 = 0.0 ("MFC_1\nSLPM Value")
            n370 = local write "MFC_1\nSLPM Value"(w916) -> ()
            n371 = Bundle(cluster=T4 {"Message"="", "Message Data"=variant} ("Message Cluster"), "Message"="MFC_1", "Message Data"=w916) -> (w920:T4)
            n372 = Enqueue Element(queue=w918, element=w920, error in (no error)=w917) -> (error out=w915:errorcluster)  [unwired: 1 in, 2 out]
          }
          frame #5 {
            w922 = FALSE ("High Cal")
            n373 = local write "High Cal"(w922) -> ()
            n374 = local write "FGGA Calibration Abort"(w922) -> ()
          }
        }
      }
      event "Span Cal - \nHigh Cal, CO Cal, Low Cal": Value Change {
        n375 = event-data() -> ()  [unwired: 1 in, 1 out]
        n376 = flat-sequence {
          tunnel: w962 -> [w968]
          tunnel: w961 -> [w967]
          tunnel: [w966] -> w960
          tunnel: [w965] -> w959
          tunnel: w960 -> [w984]
          tunnel: w959 -> [w983]
          tunnel: [w981] -> w957
          tunnel: [w980] -> w955
          tunnel: [w990] -> w958
          tunnel: w957 -> [w990]
          tunnel: [w989] -> w956
          tunnel: w955 -> [w989]
          tunnel: [w987] -> w934
          tunnel: [w987] -> w931
          tunnel: w958 -> [w1008]
          tunnel: w956 -> [w1009]
          tunnel: [w1009] -> w941
          tunnel: w949 -> [w1010]
          tunnel: [w1010] -> w939
          tunnel: [w1008] -> w937
          tunnel: w934 -> [w1007]
          tunnel: [w1006] -> w932
          tunnel: w931 -> [w1006]
          tunnel: w941 -> [w1020]
          tunnel: [w1020] -> w940
          tunnel: w939 -> [w1019]
          tunnel: [w1019] -> w938
          tunnel: w937 -> [w1017]
          tunnel: [w1017] -> w936
          tunnel: [w1016] -> w933
          tunnel: w932 -> [w1016]
          tunnel: [w1024] -> w954
          tunnel: [w1023] -> w953
          tunnel: w936 -> [w1025]
          tunnel: w938 -> [w1031]
          tunnel: w940 -> [w1026]
          tunnel: w933 -> [w1022]
          tunnel: [w1022] -> w927
          tunnel: [w1021] -> w924
          tunnel: w954 -> [w1070]
          tunnel: w953 -> [w1069]
          tunnel: [w1067] -> w952
          tunnel: [w1066] -> w951
          tunnel: [w1065] -> w928
          tunnel: w927 -> [w1065]
          tunnel: [w1064] -> w925
          tunnel: w924 -> [w1064]
          tunnel: w952 -> [w1087]
          tunnel: w951 -> [w1086]
          tunnel: [w1084] -> w950
          tunnel: [w1083] -> w946
          tunnel: [w1082] -> w929
          tunnel: w928 -> [w1082]
          tunnel: [w1081] -> w926
          tunnel: w925 -> [w1081]
          tunnel: w950 -> [w1096]
          tunnel: [w1096] -> w948
          tunnel: [w1094] -> w947
          tunnel: w946 -> [w1094]
          tunnel: [w1093] -> w930
          tunnel: w929 -> [w1092]
          tunnel: w926 -> [w1091]
          tunnel: [w1101] -> w945
          tunnel: [w1100] -> w944
          tunnel: w948 -> [w1098]
          tunnel: w947 -> [w1099]
          tunnel: w930 -> [w1097]
          tunnel: w945 -> [w1183]
          tunnel: w944 -> [w1182]
          tunnel: [w1180] -> w943
          tunnel: [w1179] -> w942
          tunnel: w943 -> [w1198]
          tunnel: w942 -> [w1197]
          tunnel: [w1195] -> w935
          frame #0 {
            w964 = TRUE
            n377 = Cluster To Array(cluster=T11 {"Message"="V2", "Message 2"="V3", "Message 3"="V4"}) -> (array=w969:string[])
            n378 = for {
              tunnel: w969 -> [w976] mode=indexing
              tunnel: w968 -> [w975]
              tunnel: w967 -> [w974]
              tunnel: [w973] -> w966
              tunnel: [w972] -> w965
              tunnel: w964 -> [w971]
              n379 = Bundle(cluster=T4 {"Message"="", "Message Data"=variant} ("Message Cluster"), "Message"=w976, "Message Data"=w971) -> (w978:T4)
              n380 = Enqueue Element(queue=w975, element=w978, error in (no error)=w974) -> (queue out=w973:refnum<queue>, error out=w972:errorcluster)  [unwired: 1 in, 1 out]
            }
            n381 = local write "High Cal"(TRUE ("High Cal")) -> ()
            n382 = local write "eV2"(w964) -> ()
            n383 = local write "eV4"(w964) -> ()
            n384 = local write "eV3"(w964) -> ()
          }
          frame #1 {
            n385 = local read "MFC_1 User Set Value"() -> (w979:dbl)
            n386 = local write "MFC_1\nSLPM Value"(w979) -> ()
            n387 = Bundle(cluster=T4 {"Message"="", "Message Data"=variant} ("Message Cluster"), "Message"="MFC_1", "Message Data"=w979) -> (w982:T4)
            n388 = Enqueue Element(queue=w984, element=w982, error in (no error)=w983) -> (queue out=w981:refnum<queue>, error out=w980:errorcluster)  [unwired: 1 in, 1 out]
          }
          frame #2 {
            n389 = for {
              N: 45 -> [w1000]
              tunnel: [w992] -> w987
              i -> [w999]
              stop <- w992 stop-if-true
              n390 = local read "FGGA Calibration Abort"() -> (w993:bool)
              n391 = case shown="True" w993 {
                selector: w993 -> [w1003 _]
                tunnel: [w1003 w1004] -> w991
                frame False {
                }
                frame True {
                  n392 = Two Button Dialog(message="Are you sure to abort FGGA Span Cal?") -> (T button?=w1004:bool)  [unwired: 2 in]
                }
              }
              n393 = local read "Network disconnected"() -> (w994:bool)
              n394 = Subtract(x=w1000, y=w999) -> (x-y=w998:i32)
              n395 = Decrement(x=w998) -> (x-1=w996:i32)
              n396 = Wait (ms)(milliseconds to wait=u32 1000) -> ()  [unwired: 1 out]
              n397 = Or(x=w994, y=w991) -> (x .or. y?=w992:bool)
              n398 = case shown="False" w991 {
                selector: w991 -> [w1002 _]
                frame False {
                  n399 = local write "FGGA Calibration Abort"(w1002) -> ()
                }
                frame True {
                }
              }
              n400 = Select(t=0, s=w992, f=w996) -> (s? t:f=w995:i32)
              n401 = local write "High Cal\nFlush Time Remain (sec)"(w995) -> ()
            }
          }
          frame #3 {
            n402 = case shown="False" w1007 {
              tunnel: w1010 -> [w1011 _]
              frame False {
                # "CO Cal if no network\ndisconnect or abort cal"
                n403 = Bundle(cluster=T4 {"Message"="", "Message Data"=variant} ("Message Cluster"), "Message"="CO CAL", "Message Data"=TRUE) -> (w1013:T4)
                n404 = Enqueue Element(queue=w1011, element=w1013) -> ()  [unwired: 2 in, 3 out]
              }
              frame True {
              }
            }
          }
          frame #4 {
            # "To Ensure\nCO CAL\nis certain"
            n405 = Wait (ms)(milliseconds to wait=u32 1000) -> ()  [unwired: 1 out]
          }
          frame #5 {
            n406 = Bundle(cluster=T4 {"Message"="", "Message Data"=variant} ("Message Cluster"), "Message"="CO CAL", "Message Data"=FALSE) -> (w1027:T4)
            n407 = Enqueue Element(queue=w1031, element=w1027) -> ()  [unwired: 2 in, 3 out]
            n408 = case shown="False" w1022 {
              selector: w1022 -> [_ w1061]
              tunnel: w1026 -> [w1038 w1062]
              tunnel: w1025 -> [w1037 w1063]
              tunnel: [w1034 w1063] -> w1024
              tunnel: [w1033 w1062] -> w1023
              tunnel: [w1032 w1061] -> w1021
              frame False {
                w1042 = TRUE
                # "Carry on if connection to cRIO is made\nor calibration not abort"
                n409 = Bundle(cluster=T4 {"Message"="", "Message Data"=variant} ("Message Cluster"), "Message"="V1", "Message Data"=w1042) -> (w1041:T4)
                n410 = local write "eV1"(w1042) -> ()
                n411 = Enqueue Element(queue=w1037, element=w1041, error in (no error)=w1038) -> (queue out=w1036:refnum<queue>, error out=w1035:errorcluster)  [unwired: 1 in, 1 out]
                n412 = for {
                  N: 60 -> [w1055]
                  tunnel: w1036 -> [w1046]
                  tunnel: w1035 -> [w1045]
                  tunnel: [w1046] -> w1034
                  tunnel: [w1045] -> w1033
                  tunnel: [w1044] -> w1032
                  i -> [w1054]
                  stop <- w1044 stop-if-true
                  n413 = local read "FGGA Calibration Abort"() -> (w1049:bool)
                  n414 = case shown="True" w1049 {
                    selector: w1049 -> [w1058 _]
                    tunnel: [w1058 w1059] -> w1047
                    frame False {
                    }
                    frame True {
                      n415 = Two Button Dialog(message="Are you sure to abort FGGA Span Cal?") -> (T button?=w1059:bool)  [unwired: 2 in]
                    }
                  }
                  n416 = Subtract(x=w1055, y=w1054) -> (x-y=w1053:i32)
                  n417 = Decrement(x=w1053) -> (x-1=w1051:i32)
                  n418 = Wait (ms)(milliseconds to wait=u32 1000) -> ()  [unwired: 1 out]
                  n419 = local read "Network disconnected"() -> (w1048:bool)
                  n420 = Or(x=w1048, y=w1047) -> (x .or. y?=w1044:bool)
                  n421 = Select(t=0, s=w1044, f=w1051) -> (s? t:f=w1050:i32)
                  n422 = local write "High Cal\nCal Time Remain (sec)"(w1050) -> ()
                  n423 = case shown="False" w1047 {
                    selector: w1047 -> [w1057 _]
                    frame False {
                      n424 = local write "FGGA Calibration Abort"(w1057) -> ()
                    }
                    frame True {
                    }
                  }
                }
              }
              frame True {
              }
            }
          }
          frame #6 {
            w1068 = FALSE
            n425 = Cluster To Array(cluster=T12 {"Message"="V2", "Message 2"="V3", "Message 3"="V4", "Message 4"="V1"}) -> (array=w1071:string[])
            n426 = for {
              tunnel: w1071 -> [w1078] mode=indexing
              tunnel: [w1077] -> w1067
              tunnel: [w1076] -> w1066
              tunnel: w1068 -> [w1075]
              tunnel: w1070 -> [w1074]
              tunnel: w1069 -> [w1073]
              n427 = Bundle(cluster=T4 {"Message"="", "Message Data"=variant} ("Message Cluster"), "Message"=w1078, "Message Data"=w1075) -> (w1080:T4)
              n428 = Enqueue Element(queue=w1074, element=w1080, error in (no error)=w1073) -> (queue out=w1077:refnum<queue>, error out=w1076:errorcluster)  [unwired: 1 in, 1 out]
            }
            n429 = local write "eV2"(w1068) -> ()
            n430 = local write "eV4"(w1068) -> ()
            n431 = local write "eV3"(w1068) -> ()
            n432 = local write "eV1"(w1068) -> ()
          }
          frame #7 {
            w1085 = 0.0 ("MFC_1\nSLPM Value")
            n433 = local write "MFC_1\nSLPM Value"(w1085) -> ()
            n434 = Bundle(cluster=T4 {"Message"="", "Message Data"=variant} ("Message Cluster"), "Message"="MFC_1", "Message Data"=w1085) -> (w1089:T4)
            n435 = Enqueue Element(queue=w1087, element=w1089, error in (no error)=w1086) -> (queue out=w1083:refnum<queue>, error out=w1084:errorcluster)  [unwired: 1 in, 1 out]
          }
          frame #8 {
            n436 = local write "High Cal"(FALSE ("High Cal")) -> ()
            n437 = Or(x=w1092, y=w1091) -> (x .or. y?=w1093:bool)
          }
          frame #9 {
            n438 = case shown="False" w1097 {
              tunnel: [w1104 w1178] -> w1101
              tunnel: [w1103 w1177] -> w1100
              tunnel: w1099 -> [w1113 w1178]
              tunnel: w1098 -> [w1111 w1177]
              frame False {
                w1109 = TRUE
                n439 = Cluster To Array(cluster=cluster{"Message":string, "Message 3":string} {"Message"="V2", "Message 3"="V4"}) -> (array=w1114:string[])
                n440 = for {
                  tunnel: w1114 -> [w1157] mode=indexing
                  tunnel: w1113 -> [w1156]
                  tunnel: [w1155] -> w1115
                  tunnel: [w1154] -> w1117
                  tunnel: w1109 -> [w1153]
                  tunnel: w1111 -> [w1152]
                  n441 = Bundle(cluster=T4 {"Message"="", "Message Data"=variant} ("Message Cluster"), "Message"=w1157, "Message Data"=w1153) -> (w1159:T4)
                  n442 = Enqueue Element(queue=w1156, element=w1159, error in (no error)=w1152) -> (queue out=w1155:refnum<queue>, error out=w1154:errorcluster)  [unwired: 1 in, 1 out]
                }
                n443 = local write "eV4"(w1109) -> ()
                n444 = local write "eV2"(w1109) -> ()
                n445 = local write "Low Cal"(TRUE ("Low Cal")) -> ()
                n446 = local read "MFC_1 User Set Value"() -> (w1118:dbl)
                n447 = local write "MFC_1\nSLPM Value"(w1118) -> ()
                n448 = Bundle(cluster=T4 {"Message"="", "Message Data"=variant} ("Message Cluster"), "Message"="MFC_1", "Message Data"=w1118) -> (w1119:T4)
                n449 = Enqueue Element(queue=w1115, element=w1119, error in (no error)=w1117) -> (queue out=w1108:refnum<queue>, error out=w1106:errorcluster)  [unwired: 1 in, 1 out]
                n450 = for {
                  N: 45 -> [w1171]
                  tunnel: [w1162] -> w1107
                  tunnel: w1108 -> [w1162]
                  tunnel: [w1161] -> w1105
                  tunnel: w1106 -> [w1161]
                  tunnel: [w1160] -> w1102
                  i -> [w1170]
                  stop <- w1160 stop-if-true
                  n451 = local read "FGGA Calibration Abort"() -> (w1165:bool)
                  n452 = case shown="True" w1165 {
                    selector: w1165 -> [w1174 _]
                    tunnel: [w1174 w1175] -> w1163
                    frame False {
                    }
                    frame True {
                      n453 = Two Button Dialog(message="Are you sure to abort FGGA Span Cal?") -> (T button?=w1175:bool)  [unwired: 2 in]
                    }
                  }
                  n454 = Subtract(x=w1171, y=w1170) -> (x-y=w1169:i32)
                  n455 = Decrement(x=w1169) -> (x-1=w1166:i32)
                  n456 = Wait (ms)(milliseconds to wait=u32 1000) -> ()  [unwired: 1 out]
                  n457 = local read "Network disconnected"() -> (w1164:bool)
                  n458 = Or(x=w1164, y=w1163) -> (x .or. y?=w1160:bool)
                  n459 = Select(t=0, s=w1160, f=w1166) -> (s? t:f=w1167:i32)
                  n460 = local write "Low Cal\nFlush Time Remain (sec)"(w1167) -> ()
                  n461 = case shown="False" w1163 {
                    selector: w1163 -> [w1173 _]
                    frame False {
                      n462 = local write "FGGA Calibration Abort"(w1173) -> ()
                    }
                    frame True {
                    }
                  }
                }
                n463 = case shown="False" w1102 {
                  tunnel: w1107 -> [w1127 w1151]
                  tunnel: w1105 -> [w1126 w1150]
                  tunnel: [w1124 w1151] -> w1104
                  tunnel: [w1122 w1150] -> w1103
                  frame False {
                    w1128 = TRUE
                    n464 = local write "eV1"(w1128) -> ()
                    n465 = Bundle(cluster=T4 {"Message"="", "Message Data"=variant} ("Message Cluster"), "Message"="V1", "Message Data"=w1128) -> (w1130:T4)
                    n466 = Enqueue Element(queue=w1127, element=w1130, error in (no error)=w1126) -> (queue out=w1125:refnum<queue>, error out=w1123:errorcluster)  [unwired: 1 in, 1 out]
                    n467 = for {
                      N: 60 -> [w1144]
                      tunnel: [w1134] -> w1124
                      tunnel: w1125 -> [w1134]
                      tunnel: w1123 -> [w1133]
                      tunnel: [w1133] -> w1122
                      i -> [w1143]
                      stop <- w1135 stop-if-true
                      n468 = local read "FGGA Calibration Abort"() -> (w1138:bool)
                      n469 = case shown="True" w1138 {
                        selector: w1138 -> [w1147 _]
                        tunnel: [w1147 w1148] -> w1136
                        frame False {
                        }
                        frame True {
                          n470 = Two Button Dialog(message="Are you sure to abort FGGA Span Cal?") -> (T button?=w1148:bool)  [unwired: 2 in]
                        }
                      }
                      n471 = Wait (ms)(milliseconds to wait=u32 1000) -> ()  [unwired: 1 out]
                      n472 = local read "Network disconnected"() -> (w1137:bool)
                      n473 = Subtract(x=w1144, y=w1143) -> (x-y=w1142:i32)
                      n474 = Decrement(x=w1142) -> (x-1=w1139:i32)
                      n475 = Or(x=w1137, y=w1136) -> (x .or. y?=w1135:bool)
                      n476 = Select(t=0, s=w1135, f=w1139) -> (s? t:f=w1140:i32)
                      n477 = local write "Low Cal\nCal Time Remain (sec)"(w1140) -> ()
                      n478 = case shown="False" w1136 {
                        selector: w1136 -> [w1146 _]
                        frame False {
                          n479 = local write "FGGA Calibration Abort"(w1146) -> ()
                        }
                        frame True {
                        }
                      }
                    }
                  }
                  frame True {
                    # "Ignore Cal if connection problem or abort button pressed"
                  }
                }
              }
              frame True {
                # "Ignore Cal if connection problem or abort button pressed"
              }
            }
          }
          frame #10 {
            w1181 = FALSE
            n480 = Cluster To Array(cluster=T13 {"Message"="V2", "Message 3"="V4", "Message 4"="V1"}) -> (array=w1184:string[])
            n481 = local write "eV1"(w1181) -> ()
            n482 = local write "eV2"(w1181) -> ()
            n483 = local write "eV4"(w1181) -> ()
            n484 = for {
              tunnel: w1184 -> [w1191] mode=indexing
              tunnel: [w1190] -> w1180
              tunnel: [w1189] -> w1179
              tunnel: w1181 -> [w1188]
              tunnel: w1183 -> [w1187]
              tunnel: w1182 -> [w1186]
              n485 = Bundle(cluster=T4 {"Message"="", "Message Data"=variant} ("Message Cluster"), "Message"=w1191, "Message Data"=w1188) -> (w1193:T4)
              n486 = Enqueue Element(queue=w1187, element=w1193, error in (no error)=w1186) -> (queue out=w1190:refnum<queue>, error out=w1189:errorcluster)  [unwired: 1 in, 1 out]
            }
          }
          frame #11 {
            w1194 = FALSE
            w1196 = 0.0 ("MFC_1\nSLPM Value")
            n487 = local write "MFC_1\nSLPM Value"(w1196) -> ()
            n488 = local write "Span Cal - \nHigh Cal, CO Cal, Low Cal"(w1194) -> ()
            n489 = local write "FGGA Calibration Abort"(w1194) -> ()
            n490 = local write "Low Cal"(w1194) -> ()
            n491 = Bundle(cluster=T4 {"Message"="", "Message Data"=variant} ("Message Cluster"), "Message"="MFC_1", "Message Data"=w1196) -> (w1200:T4)
            n492 = Enqueue Element(queue=w1198, element=w1200, error in (no error)=w1197) -> (error out=w1195:errorcluster)  [unwired: 1 in, 2 out]
          }
        }
      }
      event "Flush High Tank": Value Change {
        n493 = event-data() -> ()  [unwired: 1 in, 6 out]
        n494 = flat-sequence {
          tunnel: w1213 -> [w1218]
          tunnel: w1212 -> [w1217]
          tunnel: [w1216] -> w1211
          tunnel: [w1215] -> w1210
          tunnel: w1211 -> [w1234]
          tunnel: w1210 -> [w1233]
          tunnel: [w1231] -> w1209
          tunnel: [w1230] -> w1208
          tunnel: w1209 -> [w1237]
          tunnel: w1208 -> [w1238]
          tunnel: [w1238] -> w1203
          tunnel: [w1237] -> w1202
          tunnel: [w1251] -> w1207
          tunnel: [w1250] -> w1206
          tunnel: w1203 -> [w1249]
          tunnel: w1202 -> [w1248]
          tunnel: w1207 -> [w1266]
          tunnel: w1206 -> [w1265]
          tunnel: [w1263] -> w1204
          tunnel: [w1271] -> w1205
          tunnel: w1204 -> [w1271]
          frame #0 {
            w1214 = TRUE
            n495 = Cluster To Array(cluster=T11 {"Message"="V2", "Message 2"="V3", "Message 3"="V4"}) -> (array=w1219:string[])
            n496 = for {
              tunnel: w1219 -> [w1226] mode=indexing
              tunnel: w1218 -> [w1225]
              tunnel: w1217 -> [w1224]
              tunnel: [w1223] -> w1216
              tunnel: [w1222] -> w1215
              tunnel: w1214 -> [w1221]
              n497 = Bundle(cluster=T4 {"Message"="", "Message Data"=variant} ("Message Cluster"), "Message"=w1226, "Message Data"=w1221) -> (w1228:T4)
              n498 = Enqueue Element(queue=w1225, element=w1228, error in (no error)=w1224) -> (queue out=w1223:refnum<queue>, error out=w1222:errorcluster)  [unwired: 1 in, 1 out]
            }
            n499 = local write "eV2"(w1214) -> ()
            n500 = local write "eV4"(w1214) -> ()
            n501 = local write "eV3"(w1214) -> ()
          }
          frame #1 {
            n502 = local read "MFC_1 User Set Value"() -> (w1229:dbl)
            n503 = local write "MFC_1\nSLPM Value"(w1229) -> ()
            n504 = Bundle(cluster=T4 {"Message"="", "Message Data"=variant} ("Message Cluster"), "Message"="MFC_1", "Message Data"=w1229) -> (w1232:T4)
            n505 = Enqueue Element(queue=w1234, element=w1232, error in (no error)=w1233) -> (queue out=w1231:refnum<queue>, error out=w1230:errorcluster)  [unwired: 1 in, 1 out]
          }
          frame #2 {
            n506 = for {
              N: 15 -> [w1246]
              i -> [w1245]
              stop <- w1241 stop-if-true
              n507 = Subtract(x=w1246, y=w1245) -> (x-y=w1244:i32)
              n508 = Decrement(x=w1244) -> (x-1=w1242:i32)
              n509 = local read "Network disconnected"() -> (w1241:bool)
              n510 = Wait (ms)(milliseconds to wait=u32 1000) -> ()  [unwired: 1 out]
              n511 = Select(t=0, s=w1241, f=w1242) -> (s? t:f=→"Flush High Tank\nTime Remain (sec)":i32)
            }
          }
          frame #3 {
            w1252 = FALSE
            n512 = Cluster To Array(cluster=T11 {"Message"="V2", "Message 2"="V3", "Message 3"="V4"}) -> (array=w1253:string[])
            n513 = for {
              tunnel: w1253 -> [w1260] mode=indexing
              tunnel: [w1259] -> w1251
              tunnel: [w1258] -> w1250
              tunnel: w1252 -> [w1257]
              tunnel: w1248 -> [w1256]
              tunnel: w1249 -> [w1255]
              n514 = Bundle(cluster=T4 {"Message"="", "Message Data"=variant} ("Message Cluster"), "Message"=w1260, "Message Data"=w1257) -> (w1262:T4)
              n515 = Enqueue Element(queue=w1256, element=w1262, error in (no error)=w1255) -> (queue out=w1259:refnum<queue>, error out=w1258:errorcluster)  [unwired: 1 in, 1 out]
            }
            n516 = local write "eV2"(w1252) -> ()
            n517 = local write "eV4"(w1252) -> ()
            n518 = local write "eV3"(w1252) -> ()
          }
          frame #4 {
            w1264 = 0.0 ("MFC_1\nSLPM Value")
            n519 = local write "MFC_1\nSLPM Value"(w1264) -> ()
            n520 = Bundle(cluster=T4 {"Message"="", "Message Data"=variant} ("Message Cluster"), "Message"="MFC_1", "Message Data"=w1264) -> (w1268:T4)
            n521 = Enqueue Element(queue=w1266, element=w1268, error in (no error)=w1265) -> (error out=w1263:errorcluster)  [unwired: 1 in, 2 out]
          }
          frame #5 {
            n522 = local write "Flush High Tank"(FALSE ("High Cal")) -> ()
          }
        }
      }
      event "Flush Low Tank": Value Change {
        n523 = event-data() -> ()  [unwired: 1 in, 1 out]
        n524 = flat-sequence {
          tunnel: w1283 -> [w1288]
          tunnel: w1282 -> [w1287]
          tunnel: [w1286] -> w1281
          tunnel: [w1285] -> w1280
          tunnel: w1281 -> [w1304]
          tunnel: w1280 -> [w1303]
          tunnel: [w1301] -> w1279
          tunnel: [w1300] -> w1278
          tunnel: w1279 -> [w1307]
          tunnel: w1278 -> [w1308]
          tunnel: [w1308] -> w1273
          tunnel: [w1307] -> w1272
          tunnel: [w1321] -> w1277
          tunnel: [w1320] -> w1276
          tunnel: w1273 -> [w1319]
          tunnel: w1272 -> [w1318]
          tunnel: w1277 -> [w1336]
          tunnel: w1276 -> [w1335]
          tunnel: [w1333] -> w1274
          tunnel: [w1341] -> w1275
          tunnel: w1274 -> [w1341]
          frame #0 {
            w1284 = TRUE
            n525 = Cluster To Array(cluster=cluster{"Message":string, "Message 3":string} {"Message"="V2", "Message 3"="V4"}) -> (array=w1289:string[])
            n526 = for {
              tunnel: w1289 -> [w1296] mode=indexing
              tunnel: w1288 -> [w1295]
              tunnel: w1287 -> [w1294]
              tunnel: [w1293] -> w1286
              tunnel: [w1292] -> w1285
              tunnel: w1284 -> [w1291]
              n527 = Bundle(cluster=T4 {"Message"="", "Message Data"=variant} ("Message Cluster"), "Message"=w1296, "Message Data"=w1291) -> (w1298:T4)
              n528 = Enqueue Element(queue=w1295, element=w1298, error in (no error)=w1294) -> (queue out=w1293:refnum<queue>, error out=w1292:errorcluster)  [unwired: 1 in, 1 out]
            }
            n529 = local write "eV2"(w1284) -> ()
            n530 = local write "eV4"(w1284) -> ()
          }
          frame #1 {
            n531 = local read "MFC_1 User Set Value"() -> (w1299:dbl)
            n532 = local write "MFC_1\nSLPM Value"(w1299) -> ()
            n533 = Bundle(cluster=T4 {"Message"="", "Message Data"=variant} ("Message Cluster"), "Message"="MFC_1", "Message Data"=w1299) -> (w1302:T4)
            n534 = Enqueue Element(queue=w1304, element=w1302, error in (no error)=w1303) -> (queue out=w1301:refnum<queue>, error out=w1300:errorcluster)  [unwired: 1 in, 1 out]
          }
          frame #2 {
            n535 = for {
              N: 15 -> [w1316]
              i -> [w1315]
              stop <- w1310 stop-if-true
              n536 = Subtract(x=w1316, y=w1315) -> (x-y=w1314:i32)
              n537 = Decrement(x=w1314) -> (x-1=w1311:i32)
              n538 = local read "Network disconnected"() -> (w1310:bool)
              n539 = Wait (ms)(milliseconds to wait=u32 1000) -> ()  [unwired: 1 out]
              n540 = Select(t=0, s=w1310, f=w1311) -> (s? t:f=→"Flush Low Tank\nTime Remain (sec)":i32)
            }
          }
          frame #3 {
            w1322 = FALSE
            n541 = Cluster To Array(cluster=cluster{"Message":string, "Message 3":string} {"Message"="V2", "Message 3"="V4"}) -> (array=w1323:string[])
            n542 = for {
              tunnel: w1323 -> [w1330] mode=indexing
              tunnel: [w1329] -> w1321
              tunnel: [w1328] -> w1320
              tunnel: w1322 -> [w1327]
              tunnel: w1318 -> [w1326]
              tunnel: w1319 -> [w1325]
              n543 = Bundle(cluster=T4 {"Message"="", "Message Data"=variant} ("Message Cluster"), "Message"=w1330, "Message Data"=w1327) -> (w1332:T4)
              n544 = Enqueue Element(queue=w1326, element=w1332, error in (no error)=w1325) -> (queue out=w1329:refnum<queue>, error out=w1328:errorcluster)  [unwired: 1 in, 1 out]
            }
            n545 = local write "eV2"(w1322) -> ()
            n546 = local write "eV4"(w1322) -> ()
          }
          frame #4 {
            w1334 = 0.0 ("MFC_1\nSLPM Value")
            n547 = local write "MFC_1\nSLPM Value"(w1334) -> ()
            n548 = Bundle(cluster=T4 {"Message"="", "Message Data"=variant} ("Message Cluster"), "Message"="MFC_1", "Message Data"=w1334) -> (w1338:T4)
            n549 = Enqueue Element(queue=w1336, element=w1338, error in (no error)=w1335) -> (error out=w1333:errorcluster)  [unwired: 1 in, 2 out]
          }
          frame #5 {
            n550 = local write "Flush Low Tank"(FALSE ("High Cal")) -> ()
          }
        }
      }
      event "Flush Target Tank": Value Change {
        n551 = event-data() -> ()  [unwired: 1 in, 1 out]
        n552 = flat-sequence {
          tunnel: w1353 -> [w1361]
          tunnel: w1352 -> [w1360]
          tunnel: [w1359] -> w1351
          tunnel: [w1358] -> w1350
          tunnel: w1351 -> [w1367]
          tunnel: w1350 -> [w1366]
          tunnel: [w1364] -> w1349
          tunnel: [w1363] -> w1348
          tunnel: w1349 -> [w1370]
          tunnel: w1348 -> [w1371]
          tunnel: [w1371] -> w1343
          tunnel: [w1370] -> w1342
          tunnel: [w1387] -> w1347
          tunnel: [w1386] -> w1346
          tunnel: w1343 -> [w1385]
          tunnel: w1342 -> [w1384]
          tunnel: w1347 -> [w1392]
          tunnel: w1346 -> [w1391]
          tunnel: [w1389] -> w1344
          tunnel: [w1397] -> w1345
          tunnel: w1344 -> [w1397]
          frame #0 {
            w1357 = TRUE
            n553 = local write "eV4"(w1357) -> ()
            n554 = Bundle(cluster=T4 {"Message"="", "Message Data"=variant} ("Message Cluster"), "Message"="V4" ("Message 3"), "Message Data"=w1357) -> (w1356:T4)
            n555 = Enqueue Element(queue=w1361, element=w1356, error in (no error)=w1360) -> (queue out=w1359:refnum<queue>, error out=w1358:errorcluster)  [unwired: 1 in, 1 out]
          }
          frame #1 {
            n556 = local read "MFC_1 User Set Value"() -> (w1362:dbl)
            n557 = local write "MFC_1\nSLPM Value"(w1362) -> ()
            n558 = Bundle(cluster=T4 {"Message"="", "Message Data"=variant} ("Message Cluster"), "Message"="MFC_1", "Message Data"=w1362) -> (w1365:T4)
            n559 = Enqueue Element(queue=w1367, element=w1365, error in (no error)=w1366) -> (queue out=w1364:refnum<queue>, error out=w1363:errorcluster)  [unwired: 1 in, 1 out]
          }
          frame #2 {
            n560 = for {
              N: 15 -> [w1379]
              i -> [w1378]
              stop <- w1374 stop-if-true
              n561 = Subtract(x=w1379, y=w1378) -> (x-y=w1377:i32)
              n562 = Decrement(x=w1377) -> (x-1=w1375:i32)
              n563 = Wait (ms)(milliseconds to wait=u32 1000) -> ()  [unwired: 1 out]
              n564 = local read "Network disconnected"() -> (w1374:bool)
              n565 = Select(t=0, s=w1374, f=w1375) -> (s? t:f=→"Flush Target Tank\nTime Remain (sec)":i32)
            }
          }
          frame #3 {
            w1388 = FALSE
            n566 = Bundle(cluster=T4 {"Message"="", "Message Data"=variant} ("Message Cluster"), "Message"="V4" ("Message 3"), "Message Data"=w1388) -> (w1383:T4)
            n567 = local write "eV4"(w1388) -> ()
            n568 = Enqueue Element(queue=w1384, element=w1383, error in (no error)=w1385) -> (queue out=w1387:refnum<queue>, error out=w1386:errorcluster)  [unwired: 1 in, 1 out]
          }
          frame #4 {
            w1390 = 0.0 ("MFC_1\nSLPM Value")
            n569 = local write "MFC_1\nSLPM Value"(w1390) -> ()
            n570 = Bundle(cluster=T4 {"Message"="", "Message Data"=variant} ("Message Cluster"), "Message"="MFC_1", "Message Data"=w1390) -> (w1394:T4)
            n571 = Enqueue Element(queue=w1392, element=w1394, error in (no error)=w1391) -> (error out=w1389:errorcluster)  [unwired: 1 in, 2 out]
          }
          frame #5 {
            n572 = local write "Flush Target Tank"(FALSE ("High Cal")) -> ()
          }
        }
      }
      event "Low Cal": Value Change {
        n573 = event-data() -> ()  [unwired: 1 in, 1 out]
        n574 = flat-sequence {
          tunnel: w1409 -> [w1414]
          tunnel: w1408 -> [w1413]
          tunnel: [w1412] -> w1407
          tunnel: [w1411] -> w1406
          tunnel: w1407 -> [w1430]
          tunnel: w1406 -> [w1429]
          tunnel: [w1427] -> w1405
          tunnel: [w1426] -> w1404
          tunnel: [w1435] -> w1403
          tunnel: [w1434] -> w1402
          tunnel: w1404 -> [w1438]
          tunnel: w1405 -> [w1439]
          tunnel: w1403 -> [w1492]
          tunnel: w1402 -> [w1491]
          tunnel: [w1489] -> w1401
          tunnel: [w1488] -> w1400
          tunnel: w1401 -> [w1506]
          tunnel: w1400 -> [w1505]
          tunnel: [w1503] -> w1398
          tunnel: [w1511] -> w1399
          tunnel: w1398 -> [w1511]
          frame #0 {
            w1410 = TRUE
            n575 = Cluster To Array(cluster=cluster{"Message":string, "Message 3":string} {"Message"="V2", "Message 3"="V4"}) -> (array=w1415:string[])
            n576 = for {
              tunnel: w1415 -> [w1422] mode=indexing
              tunnel: w1414 -> [w1421]
              tunnel: w1413 -> [w1420]
              tunnel: [w1419] -> w1412
              tunnel: [w1418] -> w1411
              tunnel: w1410 -> [w1417]
              n577 = Bundle(cluster=T4 {"Message"="", "Message Data"=variant} ("Message Cluster"), "Message"=w1422, "Message Data"=w1417) -> (w1424:T4)
              n578 = Enqueue Element(queue=w1421, element=w1424, error in (no error)=w1420) -> (queue out=w1419:refnum<queue>, error out=w1418:errorcluster)  [unwired: 1 in, 1 out]
            }
            n579 = local write "eV2"(w1410) -> ()
            n580 = local write "eV4"(w1410) -> ()
          }
          frame #1 {
            n581 = local read "MFC_1 User Set Value"() -> (w1425:dbl)
            n582 = local write "MFC_1\nSLPM Value"(w1425) -> ()
            n583 = Bundle(cluster=T4 {"Message"="", "Message Data"=variant} ("Message Cluster"), "Message"="MFC_1", "Message Data"=w1425) -> (w1428:T4)
            n584 = Enqueue Element(queue=w1430, element=w1428, error in (no error)=w1429) -> (queue out=w1427:refnum<queue>, error out=w1426:errorcluster)  [unwired: 1 in, 1 out]
          }
          frame #2 {
            n585 = for {
              N: 45 -> [w1482]
              tunnel: w1439 -> [w1473]
              tunnel: w1438 -> [w1472]
              tunnel: [w1473] -> w1437
              tunnel: [w1472] -> w1436
              tunnel: [w1471] -> w1433
              i -> [w1481]
              stop <- w1471 stop-if-true
              n586 = local read "FGGA Calibration Abort"() -> (w1476:bool)
              n587 = case shown="True" w1476 {
                selector: w1476 -> [w1485 _]
                tunnel: [w1485 w1486] -> w1474
                frame False {
                }
                frame True {
                  n588 = Two Button Dialog(message="Are you sure to abort FGGA Low Cal?") -> (T button?=w1486:bool)  [unwired: 2 in]
                }
              }
              n589 = local read "Network disconnected"() -> (w1475:bool)
              n590 = Subtract(x=w1482, y=w1481) -> (x-y=w1480:i32)
              n591 = Decrement(x=w1480) -> (x-1=w1478:i32)
              n592 = Wait (ms)(milliseconds to wait=u32 1000) -> ()  [unwired: 1 out]
              n593 = Or(x=w1475, y=w1474) -> (x .or. y?=w1471:bool)
              n594 = case shown="False" w1474 {
                selector: w1474 -> [w1484 _]
                frame False {
                  n595 = local write "FGGA Calibration Abort"(w1484) -> ()
                }
                frame True {
                }
              }
              n596 = Select(t=0, s=w1471, f=w1478) -> (s? t:f=→"Low Cal\nFlush Time Remain (sec)":i32)
            }
            n597 = case shown="False" w1433 {
              tunnel: w1437 -> [w1446 w1470]
              tunnel: w1436 -> [w1445 w1469]
              tunnel: [w1443 w1470] -> w1435
              tunnel: [w1441 w1469] -> w1434
              frame False {
                w1447 = TRUE
                # "Carry on if connection to cRIO is made\nor calibration not abort"
                n598 = Bundle(cluster=T4 {"Message"="", "Message Data"=variant} ("Message Cluster"), "Message"="V1", "Message Data"=w1447) -> (w1448:T4)
                n599 = local write "eV1"(w1447) -> ()
                n600 = Enqueue Element(queue=w1446, element=w1448, error in (no error)=w1445) -> (queue out=w1444:refnum<queue>, error out=w1442:errorcluster)  [unwired: 1 in, 1 out]
                n601 = for {
                  N: 60 -> [w1463]
                  tunnel: w1444 -> [w1453]
                  tunnel: [w1453] -> w1443
                  tunnel: w1442 -> [w1452]
                  tunnel: [w1452] -> w1441
                  i -> [w1462]
                  stop <- w1454 stop-if-true
                  n602 = Subtract(x=w1463, y=w1462) -> (x-y=w1461:i32)
                  n603 = local read "FGGA Calibration Abort"() -> (w1456:bool)
                  n604 = case shown="True" w1456 {
                    selector: w1456 -> [w1466 _]
                    tunnel: [w1466 w1467] -> w1455
                    frame False {
                    }
                    frame True {
                      n605 = Two Button Dialog(message="Are you sure to abort FGGA Low Cal?") -> (T button?=w1467:bool)  [unwired: 2 in]
                    }
                  }
                  n606 = Decrement(x=w1461) -> (x-1=w1458:i32)
                  n607 = local read "Network disconnected"() -> (w1457:bool)
                  n608 = Wait (ms)(milliseconds to wait=u32 1000) -> ()  [unwired: 1 out]
                  n609 = Or(x=w1457, y=w1455) -> (x .or. y?=w1454:bool)
                  n610 = case shown="False" w1455 {
                    selector: w1455 -> [w1465 _]
                    frame False {
                      n611 = local write "FGGA Calibration Abort"(w1465) -> ()
                    }
                    frame True {
                    }
                  }
                  n612 = Select(t=0, s=w1454, f=w1458) -> (s? t:f=→"Low Cal\nCal Time Remain (sec)":i32)
                }
              }
              frame True {
              }
            }
          }
          frame #3 {
            w1490 = FALSE
            n613 = Cluster To Array(cluster=T13 {"Message"="V2", "Message 3"="V4", "Message 4"="V1"}) -> (array=w1493:string[])
            n614 = for {
              tunnel: w1493 -> [w1500] mode=indexing
              tunnel: [w1499] -> w1489
              tunnel: [w1498] -> w1488
              tunnel: w1490 -> [w1497]
              tunnel: w1492 -> [w1496]
              tunnel: w1491 -> [w1495]
              n615 = Bundle(cluster=T4 {"Message"="", "Message Data"=variant} ("Message Cluster"), "Message"=w1500, "Message Data"=w1497) -> (w1502:T4)
              n616 = Enqueue Element(queue=w1496, element=w1502, error in (no error)=w1495) -> (queue out=w1499:refnum<queue>, error out=w1498:errorcluster)  [unwired: 1 in, 1 out]
            }
            n617 = local write "eV2"(w1490) -> ()
            n618 = local write "eV4"(w1490) -> ()
            n619 = local write "eV1"(w1490) -> ()
          }
          frame #4 {
            w1504 = 0.0 ("MFC_1\nSLPM Value")
            n620 = local write "MFC_1\nSLPM Value"(w1504) -> ()
            n621 = Bundle(cluster=T4 {"Message"="", "Message Data"=variant} ("Message Cluster"), "Message"="MFC_1", "Message Data"=w1504) -> (w1508:T4)
            n622 = Enqueue Element(queue=w1506, element=w1508, error in (no error)=w1505) -> (error out=w1503:errorcluster)  [unwired: 1 in, 2 out]
          }
          frame #5 {
            w1510 = FALSE ("High Cal")
            n623 = local write "Low Cal"(w1510) -> ()
            n624 = local write "FGGA Calibration Abort"(w1510) -> ()
          }
        }
      }
      event "Target Cal": Value Change {
        n625 = event-data() -> ()  [unwired: 1 in, 1 out]
        n626 = flat-sequence {
          tunnel: w1523 -> [w1531]
          tunnel: w1522 -> [w1530]
          tunnel: [w1529] -> w1521
          tunnel: [w1528] -> w1520
          tunnel: w1521 -> [w1537]
          tunnel: w1520 -> [w1536]
          tunnel: [w1534] -> w1519
          tunnel: [w1533] -> w1518
          tunnel: w1518 -> [w1544]
          tunnel: w1519 -> [w1545]
          tunnel: [w1542] -> w1513
          tunnel: [w1541] -> w1512
          tunnel: [w1597] -> w1517
          tunnel: [w1598] -> w1516
          tunnel: w1513 -> [w1596]
          tunnel: w1512 -> [w1595]
          tunnel: w1517 -> [w1613]
          tunnel: w1516 -> [w1612]
          tunnel: [w1610] -> w1514
          tunnel: [w1618] -> w1515
          tunnel: w1514 -> [w1618]
          frame #0 {
            w1527 = TRUE
            n627 = local write "eV4"(w1527) -> ()
            n628 = Bundle(cluster=T4 {"Message"="", "Message Data"=variant} ("Message Cluster"), "Message"="V4" ("Message 3"), "Message Data"=w1527) -> (w1526:T4)
            n629 = Enqueue Element(queue=w1531, element=w1526, error in (no error)=w1530) -> (queue out=w1529:refnum<queue>, error out=w1528:errorcluster)  [unwired: 1 in, 1 out]
          }
          frame #1 {
            n630 = local read "MFC_1 User Set Value"() -> (w1532:dbl)
            n631 = local write "MFC_1\nSLPM Value"(w1532) -> ()
            n632 = Bundle(cluster=T4 {"Message"="", "Message Data"=variant} ("Message Cluster"), "Message"="MFC_1", "Message Data"=w1532) -> (w1535:T4)
            n633 = Enqueue Element(queue=w1537, element=w1535, error in (no error)=w1536) -> (queue out=w1534:refnum<queue>, error out=w1533:errorcluster)  [unwired: 1 in, 1 out]
          }
          frame #2 {
            n634 = for {
              N: 45 -> [w1589]
              tunnel: [w1580] -> w1546
              tunnel: w1545 -> [w1580]
              tunnel: [w1579] -> w1543
              tunnel: w1544 -> [w1579]
              tunnel: [w1578] -> w1540
              i -> [w1588]
              stop <- w1578 stop-if-true
              n635 = Subtract(x=w1589, y=w1588) -> (x-y=w1587:i32)
              n636 = Decrement(x=w1587) -> (x-1=w1584:i32)
              n637 = local read "FGGA Calibration Abort"() -> (w1583:bool)
              n638 = local read "Network disconnected"() -> (w1582:bool)
              n639 = case shown="True" w1583 {
                selector: w1583 -> [w1592 _]
                tunnel: [w1592 w1593] -> w1581
                frame False {
                }
                frame True {
                  n640 = Two Button Dialog(message="Are you sure to abort FGGA Target Cal?") -> (T button?=w1593:bool)  [unwired: 2 in]
                }
              }
              n641 = Wait (ms)(milliseconds to wait=u32 1000) -> ()  [unwired: 1 out]
              n642 = Or(x=w1582, y=w1581) -> (x .or. y?=w1578:bool)
              n643 = case shown="False" w1581 {
                selector: w1581 -> [w1591 _]
                frame False {
                  n644 = local write "FGGA Calibration Abort"(w1591) -> ()
                }
                frame True {
                }
              }
              n645 = Select(t=0, s=w1578, f=w1584) -> (s? t:f=→"Target Cal\nFlush Time Remain (sec)":i32)
            }
            n646 = case shown="False" w1540 {
              tunnel: w1546 -> [w1553 w1577]
              tunnel: w1543 -> [w1552 w1576]
              tunnel: [w1549 w1577] -> w1542
              tunnel: [w1548 w1576] -> w1541
              frame False {
                w1554 = TRUE
                # "Carry on if connection to cRIO is made\nor calibration not abort"
                n647 = Bundle(cluster=T4 {"Message"="", "Message Data"=variant} ("Message Cluster"), "Message"="V1", "Message Data"=w1554) -> (w1555:T4)
                n648 = local write "eV1"(w1554) -> ()
                n649 = Enqueue Element(queue=w1553, element=w1555, error in (no error)=w1552) -> (queue out=w1551:refnum<queue>, error out=w1550:errorcluster)  [unwired: 1 in, 1 out]
                n650 = for {
                  N: 60 -> [w1570]
                  tunnel: w1551 -> [w1560]
                  tunnel: w1550 -> [w1559]
                  tunnel: [w1560] -> w1549
                  tunnel: [w1559] -> w1548
                  i -> [w1569]
                  stop <- w1561 stop-if-true
                  n651 = Subtract(x=w1570, y=w1569) -> (x-y=w1568:i32)
                  n652 = Decrement(x=w1568) -> (x-1=w1566:i32)
                  n653 = local read "FGGA Calibration Abort"() -> (w1564:bool)
                  n654 = case shown="True" w1564 {
                    selector: w1564 -> [w1573 _]
                    tunnel: [w1573 w1574] -> w1562
                    frame False {
                    }
                    frame True {
                      n655 = Two Button Dialog(message="Are you sure to abort FGGA Target Cal?") -> (T button?=w1574:bool)  [unwired: 2 in]
                    }
                  }
                  n656 = Wait (ms)(milliseconds to wait=u32 1000) -> ()  [unwired: 1 out]
                  n657 = local read "Network disconnected"() -> (w1563:bool)
                  n658 = Or(x=w1563, y=w1562) -> (x .or. y?=w1561:bool)
                  n659 = case shown="False" w1562 {
                    selector: w1562 -> [w1572 _]
                    frame False {
                      n660 = local write "FGGA Calibration Abort"(w1572) -> ()
                    }
                    frame True {
                    }
                  }
                  n661 = Select(t=0, s=w1561, f=w1566) -> (s? t:f=→"Target Cal\nCal Time Remain (sec)":i32)
                }
              }
              frame True {
              }
            }
          }
          frame #3 {
            w1601 = FALSE
            n662 = Cluster To Array(cluster=cluster{"Message 3":string, "Message":string} {"Message 3"="V4", "Message"="V1"}) -> (array=w1599:string[])
            n663 = for {
              tunnel: w1599 -> [w1607] mode=indexing
              tunnel: [w1606] -> w1597
              tunnel: [w1605] -> w1598
              tunnel: w1601 -> [w1604]
              tunnel: w1596 -> [w1603]
              tunnel: w1595 -> [w1602]
              n664 = Bundle(cluster=T4 {"Message"="", "Message Data"=variant} ("Message Cluster"), "Message"=w1607, "Message Data"=w1604) -> (w1609:T4)
              n665 = Enqueue Element(queue=w1603, element=w1609, error in (no error)=w1602) -> (queue out=w1606:refnum<queue>, error out=w1605:errorcluster)  [unwired: 1 in, 1 out]
            }
            n666 = local write "eV4"(w1601) -> ()
            n667 = local write "eV1"(w1601) -> ()
          }
          frame #4 {
            w1611 = 0.0 ("MFC_1\nSLPM Value")
            n668 = local write "MFC_1\nSLPM Value"(w1611) -> ()
            n669 = Bundle(cluster=T4 {"Message"="", "Message Data"=variant} ("Message Cluster"), "Message"="MFC_1", "Message Data"=w1611) -> (w1615:T4)
            n670 = Enqueue Element(queue=w1613, element=w1615, error in (no error)=w1612) -> (error out=w1610:errorcluster)  [unwired: 1 in, 2 out]
          }
          frame #5 {
            w1617 = FALSE ("High Cal")
            n671 = local write "Target Cal"(w1617) -> ()
            n672 = local write "FGGA Calibration Abort"(w1617) -> ()
          }
        }
      }
      event "MFC_1\nSLPM Value": Value Change {
        n673 = event-data() -> ()  [unwired: 1 in, 1 out]
        n674 = local read "MFC_1\nSLPM Value"() -> (w1619:dbl)
        n675 = Bundle(cluster=T4 {"Message"="", "Message Data"=variant} ("Message Cluster"), "Message"="MFC_1", "Message Data"=w1619) -> (w1623:T4)
        n676 = Enqueue Element(queue=w1622, element=w1623, error in (no error)=w1621) -> (error out=w1620:errorcluster)  [unwired: 1 in, 2 out]
      }
      event "FGGA UDP Time Offset": Value Change {
        n677 = event-data() -> ("NewVal"=w1626:i32)  [unwired: 1 in, 5 out]
        n678 = Bundle(cluster=T4 {"Message"="", "Message Data"=variant} ("Message Cluster"), "Message"="UDP Time Offset", "Message Data"=w1626) -> (w1630:T4)
        n679 = Enqueue Element(queue=w1629, element=w1630, error in (no error)=w1628) -> (error out=w1627:errorcluster)  [unwired: 1 in, 2 out]
      }
    }
    "FGGA Event Error out" <- w744
  }
  n680 = node-c288(w14) -> ()  [unwired: 1 out]
  n681 = Create Network Stream Writer Endpoint(6:w54, 7:10 ("writer buffer size"), 9:w56, 10:"//192.168.101.17/command/reader/FGGA" ("reader url"), 11:"/command/writer/FGGA" ("writer name")) -> (0:w53:errorcluster, 3:w52:refnum<k21>)  [unwired: 2 in]
  n682 = while {
    tunnel: w6 -> [w1640]
    shift-right: [w1635] -> _
    shift-left: w52 -> [w1637]
    shift-right: [w1633] -> w49
    shift-left: w53 -> [w1639]
    tunnel: w5 -> [w1634]
    stop <- w1633 stop-if-true
    # "FGGA UI Command Sender"
    n683 = Dequeue Element(queue=w1640, error in (no error)=w1634) -> (element=w1636:T4)  [unwired: 1 in, 3 out]
    n684 = Unbundle By Name(w1636) -> ("Message"=w1638:string)
    n685 = case shown="\"UDP Time Offset\"" w1638 {
      tunnel: w1639 -> [w1641 w1645 w1652 w1659 w1666 w1673 w1680 w1687 w1694 w1701 w1708]
      tunnel: w1637 -> [w1642 w1648 w1655 w1662 w1669 w1676 w1683 w1690 w1697 w1704 w1711]
      tunnel: w1636 -> [_ w1647 w1654 w1661 w1668 w1675 w1682 w1689 w1696 w1703 w1710]
      tunnel: [w1641 w1644 w1651 w1658 w1665 w1672 w1679 w1686 w1693 w1700 w1707] -> w1633
      tunnel: [w1642 w1643 w1650 w1657 w1664 w1671 w1678 w1685 w1692 w1699 w1706] -> w1635
      frame "False", Default {
      }
      frame "V1" {
        n686 = shared-variable-write(w1648, w1645, w1647) -> (w1646:refnum<k21>, w1649:errorcluster)  [unwired: 1 in, 1 out]
        n687 = Flush Stream(8:w1649, 11:w1646) -> (0:w1644:errorcluster, 3:w1643:refnum<k21>)  [unwired: 2 in, 1 out]
      }
      frame "MFC_1" {
        n688 = shared-variable-write(w1655, w1652, w1654) -> (w1653:refnum<k21>, w1656:errorcluster)  [unwired: 1 in, 1 out]
        n689 = Flush Stream(8:w1656, 11:w1653) -> (0:w1651:errorcluster, 3:w1650:refnum<k21>)  [unwired: 2 in, 1 out]
      }
      frame "UDP Time Offset" {
        n690 = shared-variable-write(w1662, w1659, w1661) -> (w1660:refnum<k21>, w1663:errorcluster)  [unwired: 1 in, 1 out]
        n691 = Flush Stream(8:w1663, 11:w1660) -> (0:w1658:errorcluster, 3:w1657:refnum<k21>)  [unwired: 2 in, 1 out]
      }
      frame "V2" {
        n692 = shared-variable-write(w1669, w1666, w1668) -> (w1667:refnum<k21>, w1670:errorcluster)  [unwired: 1 in, 1 out]
        n693 = Flush Stream(8:w1670, 11:w1667) -> (0:w1665:errorcluster, 3:w1664:refnum<k21>)  [unwired: 2 in, 1 out]
      }
      frame "V3" {
        n694 = shared-variable-write(w1676, w1673, w1675) -> (w1674:refnum<k21>, w1677:errorcluster)  [unwired: 1 in, 1 out]
        n695 = Flush Stream(8:w1677, 11:w1674) -> (0:w1672:errorcluster, 3:w1671:refnum<k21>)  [unwired: 2 in, 1 out]
      }
      frame "V4" {
        n696 = shared-variable-write(w1683, w1680, w1682) -> (w1681:refnum<k21>, w1684:errorcluster)  [unwired: 1 in, 1 out]
        n697 = Flush Stream(8:w1684, 11:w1681) -> (0:w1679:errorcluster, 3:w1678:refnum<k21>)  [unwired: 2 in, 1 out]
      }
      frame "FGGA_pump" {
        n698 = shared-variable-write(w1690, w1687, w1689) -> (w1688:refnum<k21>, w1691:errorcluster)  [unwired: 1 in, 1 out]
        n699 = Flush Stream(8:w1691, 11:w1688) -> (0:w1686:errorcluster, 3:w1685:refnum<k21>)  [unwired: 2 in, 1 out]
      }
      frame "Flight Number" {
        n700 = shared-variable-write(w1697, w1694, w1696) -> (w1695:refnum<k21>, w1698:errorcluster)  [unwired: 1 in, 1 out]
        n701 = Flush Stream(8:w1698, 11:w1695) -> (0:w1693:errorcluster, 3:w1692:refnum<k21>)  [unwired: 2 in, 1 out]
      }
      frame "FGGA_restart" {
        n702 = shared-variable-write(w1704, w1701, w1703) -> (w1702:refnum<k21>, w1705:errorcluster)  [unwired: 1 in, 1 out]
        n703 = Flush Stream(8:w1705, 11:w1702) -> (0:w1700:errorcluster, 3:w1699:refnum<k21>)  [unwired: 2 in, 1 out]
      }
      frame "Stop File Write" {
        n704 = shared-variable-write(w1711, w1708, w1710) -> (w1709:refnum<k21>, w1712:errorcluster)  [unwired: 1 in, 1 out]
        n705 = Flush Stream(8:w1712, 11:w1709) -> (0:w1707:errorcluster, 3:w1706:refnum<k21>)  [unwired: 2 in, 1 out]
      }
    }
  }
  "FGGA command sender error out" <- w49
  n706 = local write "FGGA Calibration Abort"(FALSE ("FGGA Calibration Abort")) -> ()
  n707 = Obtain Queue(name (unnamed)="SO2_Command", element data type=w40) -> (queue out=w4:refnum<queue>, error out=w3:errorcluster)  [unwired: 3 in, 1 out]
  n708 = while {
    tunnel: w4 -> [w1716]
    tunnel: w3 -> [w1715]
    tunnel: [w1713] -> _
    stop <- FALSE stop-if-true
    # "SO2 UI Event Handler Loop"
    n709 = event shown="[5] \"SO2 CAL/Zero\": Value Change" {
      selector: _ -> [_ _ _ _ _ _ _ _ _ _ _ _ _ _ _ _ _ _ _ _ _ _ _ _ _ _ _ _]
      dyn-events: _ -> [_ _ _ _ _ _ _ _ _ _ _ _ _ _ _ _ _ _ _ _ _ _ _ _ _ _ _ _]
      timeout: _ -> [_ _ _ _ _ _ _ _ _ _ _ _ _ _ _ _ _ _ _ _ _ _ _ _ _ _ _ _]
      tunnel: w1716 -> [w1723 w1735 w1782 w1793 w1836 w1871 w1966 w1972 w1983 w1986 w1994 w2000 w2007 w2013 w2019 w2029 w2033 w2040 w2047 w2054 w2061 w2068 w2075 w2082 w2089 w2096 w2104 w2118]
      tunnel: w1715 -> [w1722 w1734 w1781 w1792 w1835 w1870 w1965 w1971 w1982 w1985 w1992 w1999 w2006 w2012 w2018 w2028 w2032 w2039 w2046 w2053 w2060 w2067 w2074 w2081 w2088 w2095 w2103 w2117]
      tunnel: [w1717 w1733 _ w1791 w1834 _ _ _ w1977 w1984 w1991 _ w2005 _ _ w2023 w2031 w2038 w2045 w2052 w2059 w2066 w2073 w2080 w2087 w2094 w2102 w2116] -> w1713
      event "eV9": Value Change {
        n710 = event-data() -> ("NewVal"=w1720:bool)  [unwired: 1 in]
        n711 = Bundle(cluster=T4 {"Message"="", "Message Data"=variant} ("Message Cluster"), "Message"="V9", "Message Data"=w1720) -> (w1718:T4)
        n712 = Enqueue Element(queue=w1723, element=w1718, error in (no error)=w1722) -> (error out=w1717:errorcluster)  [unwired: 1 in, 2 out]
      }
      event "SO2 Flush": Value Change {
        n713 = event-data() -> ()  [unwired: 1 in, 1 out]
        n714 = flat-sequence {
          tunnel: w1735 -> [w1743]
          tunnel: w1734 -> [w1742]
          tunnel: [w1738] -> w1730
          tunnel: [w1736] -> w1728
          tunnel: w1730 -> [w1745]
          tunnel: [w1747] -> w1729
          tunnel: w1728 -> [w1746]
          tunnel: [w1748] -> w1727
          tunnel: w1729 -> [w1754]
          tunnel: [w1754] -> w1732
          tunnel: [w1752] -> w1731
          tunnel: w1727 -> [w1752]
          tunnel: w1732 -> [w1766]
          tunnel: [w1765] -> w1726
          tunnel: w1731 -> [w1767]
          tunnel: [w1763] -> w1724
          tunnel: w1726 -> [w1773]
          tunnel: [w1774] -> w1725
          tunnel: w1724 -> [w1772]
          tunnel: [w1779] -> w1733
          tunnel: w1725 -> [w1779]
          frame #0 {
            w1737 = TRUE ("SO2 Flush")
            n715 = Bundle(cluster=T4 {"Message"="", "Message Data"=variant} ("Message Cluster"), "Message"="V9", "Message Data"=w1737) -> (w1739:T4)
            n716 = local write "eV9"(w1737) -> ()
            n717 = Enqueue Element(queue=w1743, element=w1739, error in (no error)=w1742) -> (queue out=w1736:refnum<queue>, error out=w1738:errorcluster)  [unwired: 1 in, 1 out]
          }
          frame #1 {
            n718 = local read "MFC_2 User Set Value"() -> (w1744:dbl)
            n719 = local write "MFC_2\nSLPM Value"(w1744) -> ()
            n720 = Bundle(cluster=T4 {"Message"="", "Message Data"=variant} ("Message Cluster"), "Message"="MFC_2", "Message Data"=w1744) -> (w1749:T4)
            n721 = Enqueue Element(queue=w1746, element=w1749, error in (no error)=w1745) -> (queue out=w1748:refnum<queue>, error out=w1747:errorcluster)  [unwired: 1 in, 1 out]
          }
          frame #2 {
            n722 = for {
              N: "eV9 Flush User\nset time (sec)" -> [w1761]
              i -> [w1760]
              stop <- w1755 stop-if-true
              n723 = local read "Network disconnected"() -> (w1755:bool)
              n724 = Subtract(x=w1761, y=w1760) -> (x-y=w1759:i32)
              n725 = Decrement(x=w1759) -> (x-1=w1757:i32)
              n726 = Wait (ms)(milliseconds to wait=u32 1000) -> ()  [unwired: 1 out]
              n727 = Select(t=0, s=w1755, f=w1757) -> (s? t:f=w1756:i32)
              n728 = local write "SO2 Flush\nTime Remain (sec)"(w1756) -> ()
            }
          }
          frame #3 {
            w1764 = FALSE
            n729 = Bundle(cluster=T4 {"Message"="", "Message Data"=variant} ("Message Cluster"), "Message"="V9", "Message Data"=w1764) -> (w1768:T4)
            n730 = local write "eV9"(w1764) -> ()
            n731 = Enqueue Element(queue=w1767, element=w1768, error in (no error)=w1766) -> (queue out=w1763:refnum<queue>, error out=w1765:errorcluster)  [unwired: 1 in, 1 out]
          }
          frame #4 {
            w1771 = 0.0 ("MFC_2\nSLPM Value")
            n732 = local write "MFC_2\nSLPM Value"(w1771) -> ()
            n733 = Bundle(cluster=T4 {"Message"="", "Message Data"=variant} ("Message Cluster"), "Message"="MFC_2", "Message Data"=w1771) -> (w1775:T4)
            n734 = Enqueue Element(queue=w1772, element=w1775, error in (no error)=w1773) -> (error out=w1774:errorcluster)  [unwired: 1 in, 2 out]
          }
          frame #5 {
            n735 = local write "SO2 Flush"(FALSE ("SO2 Flush")) -> ()
          }
        }
      }
      event "Auto Zeroing \ninterval (sec)": Value Change {
        n736 = event-data() -> ("NewVal"=w1780:i32)  [unwired: 1 in]
        n737 = Bundle(cluster=T4 {"Message"="", "Message Data"=variant} ("Message Cluster"), "Message"="zeroing_interval", "Message Data"=w1780) -> (w1783:T4)
        n738 = Enqueue Element(queue=w1782, element=w1783, error in (no error)=w1781) -> ()  [unwired: 1 in, 3 out]
      }
      event "SO2 GND Zeroing": Value Change {
        n739 = event-data() -> ()  [unwired: 1 in, 1 out]
        n740 = flat-sequence {
          tunnel: w1793 -> [w1801]
          tunnel: w1792 -> [w1800]
          tunnel: [w1796] -> w1790
          tunnel: [w1794] -> w1786
          tunnel: w1790 -> [w1804]
          tunnel: [w1804] -> w1789
          tunnel: [w1803] -> w1787
          tunnel: w1786 -> [w1803]
          tunnel: w1789 -> [w1822]
          tunnel: [w1821] -> w1788
          tunnel: w1787 -> [w1823]
          tunnel: [w1828] -> w1791
          tunnel: w1788 -> [w1828]
          frame #0 {
            w1795 = TRUE ("SO2 Flush")
            n741 = local write "SO2 eV6"(w1795) -> ()
            n742 = Bundle(cluster=T4 {"Message"="", "Message Data"=variant} ("Message Cluster"), "Message"="V6", "Message Data"=w1795) -> (w1797:T4)
            n743 = Enqueue Element(queue=w1801, element=w1797, error in (no error)=w1800) -> (queue out=w1794:refnum<queue>, error out=w1796:errorcluster)  [unwired: 1 in, 1 out]
          }
          frame #1 {
            # "10 Mins Count down"
            n744 = for {
              N: "eV6 User\nset time (sec)" -> [w1814]
              i -> [w1813]
              stop <- w1805 stop-if-true
              n745 = local read "SO2 Zeroing / Calibration Abort"() -> (w1811:bool)
              n746 = case shown="True" w1811 {
                selector: w1811 -> [w1817 _]
                tunnel: [w1817 w1818] -> w1806
                frame False {
                }
                frame True {
                  n747 = Two Button Dialog(message="Are you sure to abort SO2 Zeroing?") -> (T button?=w1818:bool)  [unwired: 2 in]
                }
              }
              n748 = Subtract(x=w1814, y=w1813) -> (x-y=w1812:i32)
              n749 = Decrement(x=w1812) -> (x-1=w1808:i32)
              n750 = Wait (ms)(milliseconds to wait=u32 1000) -> ()  [unwired: 1 out]
              n751 = local read "Network disconnected"() -> (w1809:bool)
              n752 = Or(x=w1809, y=w1806) -> (x .or. y?=w1805:bool)
              n753 = case shown="False" w1806 {
                selector: w1806 -> [w1816 _]
                frame False {
                  n754 = local write "SO2 Zeroing / Calibration Abort"(w1816) -> ()
                }
                frame True {
                }
              }
              n755 = Select(t=0, s=w1805, f=w1808) -> (s? t:f=w1807:i32)
              n756 = local write "SO2 Zeroing\nTime Remain (sec)"(w1807) -> ()
            }
          }
          frame #2 {
            w1820 = FALSE
            n757 = Bundle(cluster=T4 {"Message"="", "Message Data"=variant} ("Message Cluster"), "Message"="V6", "Message Data"=w1820) -> (w1824:T4)
            n758 = local write "SO2 eV6"(w1820) -> ()
            n759 = Enqueue Element(queue=w1823, element=w1824, error in (no error)=w1822) -> (error out=w1821:errorcluster)  [unwired: 1 in, 2 out]
          }
          frame #3 {
            n760 = local write "SO2 GND Zeroing"(FALSE ("SO2 Flush")) -> ()
          }
        }
      }
      event "SO2 Inflight \nZeroing": Value Change {
        n761 = event-data() -> ()  [unwired: 1 in, 1 out]
        n762 = flat-sequence {
          tunnel: w1836 -> [w1844]
          tunnel: w1835 -> [w1843]
          tunnel: [w1839] -> w1833
          tunnel: [w1837] -> w1829
          tunnel: w1833 -> [w1847]
          tunnel: [w1847] -> w1832
          tunnel: [w1846] -> w1830
          tunnel: w1829 -> [w1846]
          tunnel: w1832 -> [w1855]
          tunnel: [w1854] -> w1831
          tunnel: w1830 -> [w1856]
          tunnel: [w1861] -> w1834
          tunnel: w1831 -> [w1861]
          frame #0 {
            w1838 = TRUE ("SO2 Flush")
            n763 = local write "SO2 eV6"(w1838) -> ()
            n764 = Bundle(cluster=T4 {"Message"="", "Message Data"=variant} ("Message Cluster"), "Message"="V6", "Message Data"=w1838) -> (w1840:T4)
            n765 = Enqueue Element(queue=w1844, element=w1840, error in (no error)=w1843) -> (queue out=w1837:refnum<queue>, error out=w1839:errorcluster)  [unwired: 1 in, 1 out]
          }
          frame #1 {
            n766 = for {
              N: "eV6 User set time \n(Inflight) (sec)" -> [w1851]
              i -> [w1850]
              n767 = Subtract(x=w1851, y=w1850) -> (x-y=w1849:i32)
              n768 = Decrement(x=w1849) -> (x-1=w1848:i32)
              n769 = local write "SO2 Zeroing (Inflight)\nTime Remain (sec)"(w1848) -> ()
              n770 = Wait (ms)(milliseconds to wait=u32 1000) -> ()  [unwired: 1 out]
            }
          }
          frame #2 {
            w1853 = FALSE
            n771 = Bundle(cluster=T4 {"Message"="", "Message Data"=variant} ("Message Cluster"), "Message"="V6", "Message Data"=w1853) -> (w1857:T4)
            n772 = local write "SO2 eV6"(w1853) -> ()
            n773 = Enqueue Element(queue=w1856, element=w1857, error in (no error)=w1855) -> (error out=w1854:errorcluster)  [unwired: 1 in, 2 out]
          }
          frame #3 {
            n774 = local write "SO2 Inflight \nZeroing"(FALSE ("SO2 Flush")) -> ()
          }
        }
      }
      event "SO2 CAL/Zero": Value Change {
        n775 = event-data() -> ()  [unwired: 1 in, 1 out]
        n776 = flat-sequence {
          tunnel: w1871 -> [w1879]
          tunnel: w1870 -> [w1878]
          tunnel: [w1874] -> w1869
          tunnel: [w1873] -> w1867
          tunnel: w1869 -> [w1883]
          tunnel: [w1882] -> w1868
          tunnel: w1867 -> [w1884]
          tunnel: [w1880] -> w1866
          tunnel: [w1890] -> w1865
          tunnel: [w1889] -> w1864
          tunnel: w1866 -> [w1894]
          tunnel: w1868 -> [w1892]
          tunnel: w1865 -> [w1946]
          tunnel: w1864 -> [w1945]
          tunnel: [w1944] -> w1863
          tunnel: [w1943] -> w1862
          tunnel: w1863 -> [w1960]
          tunnel: w1862 -> [w1959]
          frame #0 {
            w1872 = TRUE ("SO2 Flush")
            n777 = Bundle(cluster=T4 {"Message"="", "Message Data"=variant} ("Message Cluster"), "Message"="V9", "Message Data"=w1872) -> (w1875:T4)
            n778 = local write "eV9"(w1872) -> ()
            n779 = Enqueue Element(queue=w1879, element=w1875, error in (no error)=w1878) -> (queue out=w1873:refnum<queue>, error out=w1874:errorcluster)  [unwired: 1 in, 1 out]
          }
          frame #1 {
            n780 = local read "MFC_2 User Set Value"() -> (w1881:dbl)
            n781 = local write "MFC_2\nSLPM Value"(w1881) -> ()
            n782 = Bundle(cluster=T4 {"Message"="", "Message Data"=variant} ("Message Cluster"), "Message"="MFC_2", "Message Data"=w1881) -> (w1885:T4)
            n783 = Enqueue Element(queue=w1884, element=w1885, error in (no error)=w1883) -> (queue out=w1880:refnum<queue>, error out=w1882:errorcluster)  [unwired: 1 in, 1 out]
          }
          frame #2 {
            n784 = for {
              N: "eV9 flush User\nset time (sec)" -> [w1937]
              tunnel: [w1928] -> w1893
              tunnel: w1894 -> [w1928]
              tunnel: [w1927] -> w1891
              tunnel: w1892 -> [w1927]
              tunnel: [w1926] -> w1888
              i -> [w1936]
              stop <- w1926 stop-if-true
              n785 = local read "SO2 Zeroing / Calibration Abort"() -> (w1933:bool)
              n786 = case shown="True" w1933 {
                selector: w1933 -> [w1940 _]
                tunnel: [w1940 w1941] -> w1931
                frame False {
                }
                frame True {
                  n787 = Two Button Dialog(message="Are you sure to abort SO2 Cal?") -> (T button?=w1941:bool)  [unwired: 2 in]
                }
              }
              n788 = Subtract(x=w1937, y=w1936) -> (x-y=w1935:i32)
              n789 = Decrement(x=w1935) -> (x-1=w1929:i32)
              n790 = Wait (ms)(milliseconds to wait=u32 1000) -> ()  [unwired: 1 out]
              n791 = local read "Network disconnected"() -> (w1932:bool)
              n792 = Or(x=w1932, y=w1931) -> (x .or. y?=w1926:bool)
              n793 = Select(t=0, s=w1926, f=w1929) -> (s? t:f=w1930:i32)
              n794 = local write "SO2 Cal/Zero Flush\nTime Remain (sec)"(w1930) -> ()
              n795 = case shown="False" w1931 {
                selector: w1931 -> [w1939 _]
                frame False {
                  n796 = local write "SO2 Zeroing / Calibration Abort"(w1939) -> ()
                }
                frame True {
                }
              }
            }
            n797 = case shown="False" w1888 {
              tunnel: w1893 -> [w1901 w1925]
              tunnel: w1891 -> [w1900 w1924]
              tunnel: [w1898 w1925] -> w1890
              tunnel: [w1896 w1924] -> w1889
              frame False {
                w1902 = TRUE ("SO2 Flush")
                # "carry on cal when no connection problem or abort not confirmed"
                n798 = Bundle(cluster=T4 {"Message"="", "Message Data"=variant} ("Message Cluster"), "Message"="V8", "Message Data"=w1902) -> (w1903:T4)
                n799 = local write "eV8"(w1902) -> ()
                n800 = Enqueue Element(queue=w1901, element=w1903, error in (no error)=w1900) -> (queue out=w1899:refnum<queue>, error out=w1897:errorcluster)  [unwired: 1 in, 1 out]
                n801 = for {
                  N: "eV8 User\nset time (sec)" -> [w1918]
                  tunnel: [w1908] -> w1898
                  tunnel: w1899 -> [w1908]
                  tunnel: [w1907] -> w1896
                  tunnel: w1897 -> [w1907]
                  i -> [w1917]
                  stop <- w1909 stop-if-true
                  n802 = local read "SO2 Zeroing / Calibration Abort"() -> (w1915:bool)
                  n803 = case shown="True" w1915 {
                    selector: w1915 -> [w1921 _]
                    tunnel: [w1921 w1922] -> w1912
                    frame False {
                    }
                    frame True {
                      n804 = Two Button Dialog(message="Are you sure to abort SO2 Cal?") -> (T button?=w1922:bool)  [unwired: 2 in]
                    }
                  }
                  n805 = Subtract(x=w1918, y=w1917) -> (x-y=w1916:i32)
                  n806 = local read "Network disconnected"() -> (w1913:bool)
                  n807 = Decrement(x=w1916) -> (x-1=w1911:i32)
                  n808 = Or(x=w1913, y=w1912) -> (x .or. y?=w1909:bool)
                  n809 = Select(t=0, s=w1909, f=w1911) -> (s? t:f=w1910:i32)
                  n810 = case shown="False" w1912 {
                    selector: w1912 -> [w1920 _]
                    frame False {
                      n811 = local write "SO2 Zeroing / Calibration Abort"(w1920) -> ()
                    }
                    frame True {
                    }
                  }
                  n812 = local write "SO2 CAL/Zero\nTime Remain (sec)"(w1910) -> ()
                  n813 = Wait (ms)(milliseconds to wait=u32 1000) -> ()  [unwired: 1 out]
                }
              }
              frame True {
                # "Ignore the rest of the cal when there is connection problem or abort confirmed"
              }
            }
          }
          frame #3 {
            n814 = Cluster To Array(cluster=cluster{"Message":string, "Message 2":string} {"Message"="V8", "Message 2"="V9"}) -> (array=w1948:string[])
            n815 = for {
              tunnel: w1948 -> [w1955] mode=indexing
              tunnel: FALSE ("SO2 Flush") -> [w1954]
              tunnel: w1946 -> [w1953]
              tunnel: w1945 -> [w1952]
              tunnel: [w1951] -> w1944
              tunnel: [w1950] -> w1943
              n816 = Bundle(cluster=T4 {"Message"="", "Message Data"=variant} ("Message Cluster"), "Message"=w1955, "Message Data"=w1954) -> (w1956:T4)
              n817 = Enqueue Element(queue=w1953, element=w1956, error in (no error)=w1952) -> (queue out=w1951:refnum<queue>, error out=w1950:errorcluster)  [unwired: 1 in, 1 out]
            }
          }
          frame #4 {
            w1958 = 0.0 ("MFC_2\nSLPM Value")
            n818 = local write "MFC_2\nSLPM Value"(w1958) -> ()
            n819 = Bundle(cluster=T4 {"Message"="", "Message Data"=variant} ("Message Cluster"), "Message"="MFC_2", "Message Data"=w1958) -> (w1961:T4)
            n820 = Enqueue Element(queue=w1960, element=w1961, error in (no error)=w1959) -> ()  [unwired: 1 in, 3 out]
          }
          frame #5 {
            w1964 = FALSE ("SO2 Flush")
            n821 = local write "eV9"(w1964) -> ()
            n822 = local write "SO2 Zeroing / Calibration Abort"(w1964) -> ()
            n823 = local write "eV8"(w1964) -> ()
            n824 = local write "SO2 CAL/Zero"(w1964) -> ()
          }
        }
      }
      event "eV8 User\nset time (sec)": Value Change {
        n825 = event-data() -> ("NewVal"=w1967:i32)  [unwired: 1 in]
        n826 = Bundle(cluster=T4 {"Message"="", "Message Data"=variant} ("Message Cluster"), "Message"="eV8_user_set_time", "Message Data"=w1967) -> (w1968:T4)
        n827 = Enqueue Element(queue=w1966, element=w1968, error in (no error)=w1965) -> ()  [unwired: 1 in, 3 out]
      }
      event "Offset Mean Zero Calculation (default = ON)\nOFF = User input\nOn = Mean zero calculated with ev8": Value Change {
        n828 = event-data() -> ("NewVal"=w1973:bool)  [unwired: 1 in]
        n829 = Bundle(cluster=T4 {"Message"="", "Message Data"=variant} ("Message Cluster"), "Message"="mean_cal_status", "Message Data"=w1973) -> (w1974:T4)
        n830 = Enqueue Element(queue=w1972, element=w1974, error in (no error)=w1971) -> ()  [unwired: 1 in, 3 out]
      }
      event "MFC_2\nSLPM Value": Value Change {
        n831 = event-data() -> ("NewVal"=w1980:dbl)  [unwired: 1 in]
        n832 = Bundle(cluster=T4 {"Message"="", "Message Data"=variant} ("Message Cluster"), "Message"="MFC_2", "Message Data"=w1980) -> (w1978:T4)
        n833 = Enqueue Element(queue=w1983, element=w1978, error in (no error)=w1982) -> (error out=w1977:errorcluster)  [unwired: 1 in, 2 out]
      }
      event "SO2 Inflight MOCCA Alarm\n(default = OFF)": Value Change {
        n834 = event-data() -> ("NewVal"=w1987:bool)  [unwired: 1 in]
        n835 = Bundle(cluster=T4 {"Message"="", "Message Data"=variant} ("Message Cluster"), "Message"="SO2_MOCCA_Alarm", "Message Data"=w1987) -> (w1988:T4)
        n836 = Enqueue Element(queue=w1986, element=w1988, error in (no error)=w1985) -> (error out=w1984:errorcluster)  [unwired: 1 in, 2 out]
      }
      event "MOCCA window \ndelay time (sec)": Value Change {
        n837 = event-data() -> ("NewVal"=w1993:i32)  [unwired: 1 in]
        n838 = Bundle(cluster=T4 {"Message"="", "Message Data"=variant} ("Message Cluster"), "Message"="MOCCA_window_delay_time", "Message Data"=w1993) -> (w1995:T4)
        n839 = Enqueue Element(queue=w1994, element=w1995, error in (no error)=w1992) -> (error out=w1991:errorcluster)  [unwired: 1 in, 2 out]
      }
      event "MOCCA Limit": Value Change {
        n840 = event-data() -> ("NewVal"=w1998:i32)  [unwired: 1 in]
        n841 = Bundle(cluster=T4 {"Message"="", "Message Data"=variant} ("Message Cluster"), "Message"="MOCCA_limit", "Message Data"=w1998) -> (w2001:T4)
        n842 = Enqueue Element(queue=w2000, element=w2001, error in (no error)=w1999) -> ()  [unwired: 1 in, 3 out]
      }
      event "Save Calibration gas\ncylinder concentration to file": Value Change {
        n843 = event-data() -> ("NewVal"=w2004:bool)  [unwired: 1 in]
        n844 = Bundle(cluster=T4 {"Message"="", "Message Data"=variant} ("Message Cluster"), "Message"="calcon_save", "Message Data"=w2004) -> (w2008:T4)
        n845 = Enqueue Element(queue=w2007, element=w2008, error in (no error)=w2006) -> (error out=w2005:errorcluster)  [unwired: 1 in, 2 out]
      }
      event "Calibration gas cylinder \nconcentration (ppb)": Value Change {
        n846 = event-data() -> ("NewVal"=w2011:dbl)  [unwired: 1 in]
        n847 = Bundle(cluster=T4 {"Message"="", "Message Data"=variant} ("Message Cluster"), "Message"="cal_gas_cylin_conc", "Message Data"=w2011) -> (w2014:T4)
        n848 = Enqueue Element(queue=w2013, element=w2014, error in (no error)=w2012) -> ()  [unwired: 1 in, 3 out]
      }
      event "Simulate MOCCA Conc": Value Change {
        n849 = event-data() -> ("NewVal"=w2017:dbl)  [unwired: 1 in]
        n850 = Bundle(cluster=T4 {"Message"="", "Message Data"=variant} ("Message Cluster"), "Message"="sim_MOCCA_conc", "Message Data"=w2017) -> (w2020:T4)
        n851 = Enqueue Element(queue=w2019, element=w2020, error in (no error)=w2018) -> ()  [unwired: 1 in, 3 out]
      }
      event "MFC_3\nSLPM Value": Value Change {
        n852 = event-data() -> ("NewVal"=w2026:dbl)  [unwired: 1 in]
        n853 = Bundle(cluster=T4 {"Message"="", "Message Data"=variant} ("Message Cluster"), "Message"="MFC_3", "Message Data"=w2026) -> (w2024:T4)
        n854 = Enqueue Element(queue=w2029, element=w2024, error in (no error)=w2028) -> (error out=w2023:errorcluster)  [unwired: 1 in, 2 out]
      }
      event "eV8": Value Change {
        n855 = event-data() -> ("NewVal"=w2030:bool)  [unwired: 1 in]
        n856 = Bundle(cluster=T4 {"Message"="", "Message Data"=variant} ("Message Cluster"), "Message"="V8", "Message Data"=w2030) -> (w2034:T4)
        n857 = Enqueue Element(queue=w2033, element=w2034, error in (no error)=w2032) -> (error out=w2031:errorcluster)  [unwired: 1 in, 2 out]
      }
      event "SO2 eV6": Value Change {
        n858 = event-data() -> ("NewVal"=w2037:bool)  [unwired: 1 in]
        n859 = Bundle(cluster=T4 {"Message"="", "Message Data"=variant} ("Message Cluster"), "Message"="V6", "Message Data"=w2037) -> (w2041:T4)
        n860 = Enqueue Element(queue=w2040, element=w2041, error in (no error)=w2039) -> (error out=w2038:errorcluster)  [unwired: 1 in, 2 out]
      }
      event "Simulate Conc": Value Change {
        n861 = event-data() -> ("NewVal"=w2044:bool)  [unwired: 1 in]
        n862 = Bundle(cluster=T4 {"Message"="", "Message Data"=variant} ("Message Cluster"), "Message"="Simulate Conc", "Message Data"=w2044) -> (w2048:T4)
        n863 = Enqueue Element(queue=w2047, element=w2048, error in (no error)=w2046) -> (error out=w2045:errorcluster)  [unwired: 1 in, 2 out]
      }
      event "SO2 UDP Time Offset": Value Change {
        n864 = event-data() -> ("NewVal"=w2051:i32)  [unwired: 1 in]
        n865 = Bundle(cluster=T4 {"Message"="", "Message Data"=variant} ("Message Cluster"), "Message"="UDP Time Offset", "Message Data"=w2051) -> (w2055:T4)
        n866 = Enqueue Element(queue=w2054, element=w2055, error in (no error)=w2053) -> (error out=w2052:errorcluster)  [unwired: 1 in, 2 out]
      }
      event "Simulate STEL Conc": Value Change {
        n867 = event-data() -> ("NewVal"=w2058:dbl)  [unwired: 1 in]
        n868 = Bundle(cluster=T4 {"Message"="", "Message Data"=variant} ("Message Cluster"), "Message"="Simulate STEL Conc", "Message Data"=w2058) -> (w2062:T4)
        n869 = Enqueue Element(queue=w2061, element=w2062, error in (no error)=w2060) -> (error out=w2059:errorcluster)  [unwired: 1 in, 2 out]
      }
      event "Simulate TWA Conc": Value Change {
        n870 = event-data() -> ("NewVal"=w2065:dbl)  [unwired: 1 in]
        n871 = Bundle(cluster=T4 {"Message"="", "Message Data"=variant} ("Message Cluster"), "Message"="Simulate TWA Conc", "Message Data"=w2065) -> (w2069:T4)
        n872 = Enqueue Element(queue=w2068, element=w2069, error in (no error)=w2067) -> (error out=w2066:errorcluster)  [unwired: 1 in, 2 out]
      }
      event "10mins STEL Limit": Value Change {
        n873 = event-data() -> ("NewVal"=w2072:i32)  [unwired: 1 in]
        n874 = Bundle(cluster=T4 {"Message"="", "Message Data"=variant} ("Message Cluster"), "Message"="10mins STEL Limit", "Message Data"=w2072) -> (w2076:T4)
        n875 = Enqueue Element(queue=w2075, element=w2076, error in (no error)=w2074) -> (error out=w2073:errorcluster)  [unwired: 1 in, 2 out]
      }
      event "8hr TWA Limit": Value Change {
        n876 = event-data() -> ("NewVal"=w2079:i32)  [unwired: 1 in]
        n877 = Bundle(cluster=T4 {"Message"="", "Message Data"=variant} ("Message Cluster"), "Message"="8hr TWA Limit", "Message Data"=w2079) -> (w2083:T4)
        n878 = Enqueue Element(queue=w2082, element=w2083, error in (no error)=w2081) -> (error out=w2080:errorcluster)  [unwired: 1 in, 2 out]
      }
      event "SO2 Zero": Value Change {
        n879 = event-data() -> ("NewVal"=w2086:dbl)  [unwired: 1 in]
        n880 = Bundle(cluster=T4 {"Message"="", "Message Data"=variant} ("Message Cluster"), "Message"="Offset", "Message Data"=w2086) -> (w2090:T4)
        n881 = Enqueue Element(queue=w2089, element=w2090, error in (no error)=w2088) -> (error out=w2087:errorcluster)  [unwired: 1 in, 2 out]
      }
      event "SO2 Sensitivity": Value Change {
        n882 = event-data() -> ("NewVal"=w2093:dbl)  [unwired: 1 in]
        n883 = Bundle(cluster=T4 {"Message"="", "Message Data"=variant} ("Message Cluster"), "Message"="Slope", "Message Data"=w2093) -> (w2097:T4)
        n884 = Enqueue Element(queue=w2096, element=w2097, error in (no error)=w2095) -> (error out=w2094:errorcluster)  [unwired: 1 in, 2 out]
      }
      event "Confirm Flight Number": Value Change {
        n885 = event-data() -> ()  [unwired: 1 in, 6 out]
        n886 = flat-sequence {
          tunnel: w2103 -> [w2106]
          tunnel: w2104 -> [w2107]
          tunnel: [w2107] -> w2101
          tunnel: [w2106] -> w2100
          tunnel: [w2109] -> w2102
          tunnel: w2101 -> [w2111]
          tunnel: w2100 -> [w2110]
          frame #0 {
            n887 = local write "cRIO File IO Stop\n(USB Flash Drive Unmount)"(FALSE ("cRIO File IO Stop\n(USB Flash Drive Unmount)")) -> ()
          }
          frame #1 {
            n888 = local read "Flight Number"() -> (w2108:string)
            n889 = Bundle(cluster=T4 {"Message"="", "Message Data"=variant} ("Message Cluster"), "Message"="Flight Number", "Message Data"=w2108) -> (w2112:T4)
            n890 = Enqueue Element(queue=w2111, element=w2112, error in (no error)=w2110) -> (error out=w2109:errorcluster)  [unwired: 1 in, 2 out]
          }
        }
      }
      event "cRIO File IO Stop\n(USB Flash Drive Unmount)": Value Change {
        n891 = event-data() -> ("NewVal"=w2115:bool)  [unwired: 1 in]
        n892 = Bundle(cluster=T4 {"Message"="", "Message Data"=variant} ("Message Cluster"), "Message"="Stop File Write", "Message Data"=w2115) -> (w2119:T4)
        n893 = Enqueue Element(queue=w2118, element=w2119, error in (no error)=w2117) -> (error out=w2116:errorcluster)  [unwired: 1 in, 2 out]
      }
    }
    "SO2 Event error out" <- w1713
  }
  n894 = Create Network Stream Writer Endpoint(6:w45, 7:10 ("writer buffer size"), 9:w40, 10:"//192.168.101.17/command/reader/SO2" ("reader url"), 11:"/command/writer/SO2" ("writer name")) -> (0:w44:errorcluster, 3:w43:refnum<k21>)  [unwired: 2 in]
  n895 = while {
    tunnel: w4 -> [w2126]
    tunnel: w3 -> [w2125]
    stop <- FALSE stop-if-true
    # "SO2 Auto Zero Handler Loop"
    n896 = local read "Network disconnected"() -> (w2123:bool)
    n897 = local read "SO2 CAL/Zero"() -> (w2130:bool)
    n898 = Equal?(x=w2130, y=FALSE) -> (x = y?=w2128:bool)
    n899 = Equal?(x=w2123, y=FALSE) -> (x = y?=w2122:bool)
    n900 = Compound Arithmetic op=AND("SO2 Auto Zeroing", w2128, w2122) -> (w2131:bool)
    n901 = case shown="True" w2131 {
      tunnel: w2126 -> [_ w2150]
      tunnel: w2125 -> [_ w2149]
      frame False {
        n902 = local write "Auto Zero\nIndicator"("Auto Zero Inactive; Manual Zero Allow" ("Auto Zero Indicator")) -> ()
        n903 = local write "SO2 Pause\nAuto Zeroing"(FALSE ("SO2 Pause\nAuto Zeroing")) -> ()
        n904 = property on="SO2 CAL/Zero" class="Bool (strict)"("Visible"=TRUE) -> ()  [unwired: 2 in, 2 out]
      }
      frame True {
        n905 = flat-sequence {
          tunnel: w2149 -> [w2159]
          tunnel: w2150 -> [w2160]
          tunnel: [w2160] -> w2148
          tunnel: [w2159] -> w2147
          tunnel: w2148 -> [w2169]
          tunnel: w2147 -> [w2168]
          tunnel: [w2167] -> w2146
          tunnel: [w2166] -> w2145
          tunnel: [w2175] -> w2156
          tunnel: [w2174] -> w2155
          tunnel: w2146 -> [w2179]
          tunnel: w2145 -> [w2180]
          tunnel: w2156 -> [w2184]
          tunnel: [w2183] -> w2154
          tunnel: w2155 -> [w2185]
          tunnel: [w2182] -> w2153
          tunnel: w2154 -> [w2193]
          tunnel: w2153 -> [w2195]
          tunnel: [w2191] -> w2138
          tunnel: [w2190] -> w2137
          tunnel: [w2245] -> w2152
          tunnel: [w2244] -> w2151
          tunnel: w2138 -> [w2247]
          tunnel: w2137 -> [w2246]
          tunnel: w2152 -> [w2263]
          tunnel: w2151 -> [w2262]
          tunnel: [w2260] -> w2143
          tunnel: [w2259] -> w2142
          tunnel: [w2268] -> w2144
          tunnel: w2143 -> [w2268]
          tunnel: w2142 -> [w2267]
          tunnel: [w2267] -> w2141
          tunnel: [w2273] -> w2140
          tunnel: w2141 -> [w2272]
          tunnel: w2144 -> [w2273]
          tunnel: [w2272] -> w2139
          tunnel: w2140 -> [w2307]
          tunnel: w2139 -> [w2306]
          frame #0 {
            n906 = local write "Auto Zero\nIndicator"("Auto Zero In Progress" ("Auto Zero\nIndicator")) -> ()
            n907 = while {
              stop <- w2161 stop-if-true
              n908 = local read "eV9"() -> (w2163:bool)
              n909 = Equal?(x=w2163, y=FALSE) -> (x = y?=w2161:bool)
              n910 = Wait (ms)(milliseconds to wait=u32 1000) -> ()  [unwired: 1 out]
            }
            n911 = property on="SO2 CAL/Zero" class="Bool (strict)"("Visible"=FALSE) -> ()  [unwired: 2 in, 2 out]
          }
          frame #1 {
            n912 = Bundle(cluster=T4 {"Message"="", "Message Data"=variant} ("Message Cluster"), "Message"="Auto_zero", "Message Data"=TRUE) -> (w2170:T4)
            n913 = Enqueue Element(queue=w2169, element=w2170, error in (no error)=w2168) -> (queue out=w2166:refnum<queue>, error out=w2167:errorcluster)  [unwired: 1 in, 1 out]
          }
          frame #2 {
            w2173 = TRUE ("SO2 Flush")
            n914 = Bundle(cluster=T4 {"Message"="", "Message Data"=variant} ("Message Cluster"), "Message"="V9", "Message Data"=w2173) -> (w2176:T4)
            n915 = local write "eV9"(w2173) -> ()
            n916 = Enqueue Element(queue=w2180, element=w2176, error in (no error)=w2179) -> (queue out=w2174:refnum<queue>, error out=w2175:errorcluster)  [unwired: 1 in, 1 out]
          }
          frame #3 {
            n917 = local read "MFC_2 User Set Value"() -> (w2181:dbl)
            n918 = local write "MFC_2 User Set Value"(w2181) -> ()
            n919 = Bundle(cluster=T4 {"Message"="", "Message Data"=variant} ("Message Cluster"), "Message"="MFC_2", "Message Data"=w2181) -> (w2186:T4)
            n920 = Enqueue Element(queue=w2185, element=w2186, error in (no error)=w2184) -> (queue out=w2182:refnum<queue>, error out=w2183:errorcluster)  [unwired: 1 in, 1 out]
          }
          frame #4 {
            n921 = local read "eV9 flush User\nset time (sec)"() -> (w2196:i32)
            n922 = for {
              N: w2196 -> [w2238]
              tunnel: [w2229] -> w2194
              tunnel: w2195 -> [w2229]
              tunnel: [w2228] -> w2192
              tunnel: w2193 -> [w2228]
              tunnel: [w2227] -> w2189
              i -> [w2237]
              stop <- w2227 stop-if-true
              n923 = local read "SO2 Zeroing / Calibration Abort"() -> (w2232:bool)
              n924 = case shown="True" w2232 {
                selector: w2232 -> [w2241 _]
                tunnel: [w2241 w2242] -> w2230
                frame False {
                }
                frame True {
                  n925 = Two Button Dialog(message="Are you sure to abort SO2 Cal?") -> (T button?=w2242:bool)  [unwired: 2 in]
                }
              }
              n926 = local read "Network disconnected"() -> (w2231:bool)
              n927 = Subtract(x=w2238, y=w2237) -> (x-y=w2236:i32)
              n928 = Decrement(x=w2236) -> (x-1=w2234:i32)
              n929 = Or(x=w2230, y=w2231) -> (x .or. y?=w2227:bool)
              n930 = Wait (ms)(milliseconds to wait=u32 1000) -> ()  [unwired: 1 out]
              n931 = Select(t=0, s=w2227, f=w2234) -> (s? t:f=w2233:i32)
              n932 = local write "SO2 Cal/Zero Flush\nTime Remain (sec)"(w2233) -> ()
              n933 = case shown="False" w2230 {
                selector: w2230 -> [w2240 _]
                frame False {
                  n934 = local write "SO2 Zeroing / Calibration Abort"(w2240) -> ()
                }
                frame True {
                }
              }
            }
            n935 = case shown="False" w2189 {
              tunnel: w2194 -> [w2202 w2226]
              tunnel: w2192 -> [w2201 w2225]
              tunnel: [w2200 w2226] -> w2191
              tunnel: [w2198 w2225] -> w2190
              frame False {
                w2203 = TRUE ("SO2 Flush")
                # "carry on cal when no connection problem or abort not confirmed"
                n936 = Bundle(cluster=T4 {"Message"="", "Message Data"=variant} ("Message Cluster"), "Message"="V8", "Message Data"=w2203) -> (w2204:T4)
                n937 = local write "eV8"(w2203) -> ()
                n938 = Enqueue Element(queue=w2202, element=w2204, error in (no error)=w2201) -> (queue out=w2199:refnum<queue>, error out=w2197:errorcluster)  [unwired: 1 in, 1 out]
                n939 = local read "eV8 User\nset time (sec)"() -> (w2207:i32)
                n940 = for {
                  N: w2207 -> [w2219]
                  tunnel: w2199 -> [w2209]
                  tunnel: [w2209] -> w2200
                  tunnel: w2197 -> [w2208]
                  tunnel: [w2208] -> w2198
                  i -> [w2218]
                  stop <- w2210 stop-if-true
                  n941 = local read "SO2 Zeroing / Calibration Abort"() -> (w2216:bool)
                  n942 = case shown="True" w2216 {
                    selector: w2216 -> [w2222 _]
                    tunnel: [w2222 w2223] -> w2211
                    frame False {
                    }
                    frame True {
                      n943 = Two Button Dialog(message="Are you sure to abort SO2 Cal?") -> (T button?=w2223:bool)  [unwired: 2 in]
                    }
                  }
                  n944 = local read "Network disconnected"() -> (w2214:bool)
                  n945 = Subtract(x=w2219, y=w2218) -> (x-y=w2217:i32)
                  n946 = Decrement(x=w2217) -> (x-1=w2212:i32)
                  n947 = Or(x=w2211, y=w2214) -> (x .or. y?=w2210:bool)
                  n948 = Wait (ms)(milliseconds to wait=u32 1000) -> ()  [unwired: 1 out]
                  n949 = Select(t=0, s=w2210, f=w2212) -> (s? t:f=w2213:i32)
                  n950 = case shown="False" w2211 {
                    selector: w2211 -> [w2221 _]
                    frame False {
                      n951 = local write "SO2 Zeroing / Calibration Abort"(w2221) -> ()
                    }
                    frame True {
                    }
                  }
                  n952 = local write "SO2 CAL/Zero\nTime Remain (sec)"(w2213) -> ()
                }
              }
              frame True {
                # "Ignore cal when connection problem or abort confirmed"
              }
            }
          }
          frame #5 {
            n953 = Cluster To Array(cluster=cluster{"Message":string, "Message 2":string} {"Message"="V8", "Message 2"="V9"}) -> (array=w2249:string[])
            n954 = for {
              tunnel: w2249 -> [w2256] mode=indexing
              tunnel: FALSE ("SO2 Flush") -> [w2255]
              tunnel: w2247 -> [w2254]
              tunnel: w2246 -> [w2253]
              tunnel: [w2252] -> w2245
              tunnel: [w2251] -> w2244
              n955 = Bundle(cluster=T4 {"Message"="", "Message Data"=variant} ("Message Cluster"), "Message"=w2256, "Message Data"=w2255) -> (w2257:T4)
              n956 = Enqueue Element(queue=w2254, element=w2257, error in (no error)=w2253) -> (queue out=w2252:refnum<queue>, error out=w2251:errorcluster)  [unwired: 1 in, 1 out]
            }
          }
          frame #6 {
            w2261 = 0.0 ("MFC_2\nSLPM Value")
            n957 = local write "MFC_2\nSLPM Value"(w2261) -> ()
            n958 = Bundle(cluster=T4 {"Message"="", "Message Data"=variant} ("Message Cluster"), "Message"="MFC_2", "Message Data"=w2261) -> (w2264:T4)
            n959 = Enqueue Element(queue=w2263, element=w2264, error in (no error)=w2262) -> (queue out=w2260:refnum<queue>, error out=w2259:errorcluster)  [unwired: 1 in, 1 out]
          }
          frame #7 {
            w2269 = FALSE ("SO2 Flush")
            n960 = local write "eV8"(w2269) -> ()
            n961 = local write "eV9"(w2269) -> ()
          }
          frame #8 {
            n962 = for {
              N: "Auto Zeroing \ninterval (sec)" -> [w2285]
              tunnel: [w2280] -> w2270
              i -> [w2284]
              stop <- w2280 stop-if-true
              n963 = local read "SO2 Pause\nAuto Zeroing"() -> (w2278:bool)
              n964 = Subtract(x=w2285, y=w2284) -> (x-y=w2286:i32)
              n965 = Equal?(x=w2278, y=TRUE) -> (x = y?=w2276:bool)
              n966 = Decrement(x=w2286) -> (x-1=→"Next Auto Zero\nStarts in (sec)":i32)
              n967 = Wait (ms)(milliseconds to wait=u32 1000) -> ()  [unwired: 1 out]
              n968 = case shown="True" w2276 {
                selector: w2276 -> [w2288 _]
                tunnel: [w2288 FALSE] -> w2275
                frame False {
                }
                frame True {
                  n969 = for {
                    N: "Pause Auto Zero Count \nDown set time (sec)" -> [w2302]
                    tunnel: [w2294] -> w2290
                    i -> [w2301]
                    stop <- w2294 stop-if-true
                    w2295 = FALSE
                    n970 = local read "SO2 Pause\nAuto Zeroing"() -> (w2297:bool)
                    n971 = local read "SO2 Auto Zeroing"() -> (w2298:bool)
                    n972 = Subtract(x=w2302, y=w2301) -> (x-y=w2303:i32)
                    n973 = Decrement(x=w2303) -> (x-1=→"SO2 Resume Zeroing\nCount down timer (sec)":i32)
                    n974 = Wait (ms)(milliseconds to wait=u32 1000) -> ()  [unwired: 1 out]
                    n975 = Equal?(x=w2298, y=w2295) -> (x = y?=w2299:bool)
                    n976 = Equal?(x=w2297, y=w2295) -> (x = y?=w2296:bool)
                    n977 = Or(x=w2299, y=w2296) -> (x .or. y?=w2294:bool)
                  }
                  n978 = case shown="True" w2290 {
                    frame False {
                    }
                    frame True {
                      n979 = local write "SO2 Resume Zeroing\nCount down timer (sec)"(u32 0 ("SO2 Resume Zeroing\nCount down timer (sec)")) -> ()
                    }
                  }
                  n980 = local write "Auto Zero\nIndicator"("Auto Zero Paused" ("Auto Zero\nIndicator")) -> ()
                }
              }
              n981 = local write "Auto Zero\nIndicator"("Waiting For The Next Zeroing\nInterrupt Waiting by Pressing Pause Auto Zeroing button " ("Auto Zero\nIndicator")) -> ()
              n982 = local read "SO2 Auto Zeroing"() -> (w2281:bool)
              n983 = local write "SO2 Pause\nAuto Zeroing"(w2275) -> ()
              n984 = Equal?(x=w2281, y=FALSE) -> (x = y?=w2280:bool)
            }
            n985 = case shown="True" w2270 {
              frame False {
              }
              frame True {
                n986 = local write "Next Auto Zero\nStarts in (sec)"(u32 0 ("Next Auto Zero\nStarts in (sec)")) -> ()
              }
            }
          }
          frame #9 {
            n987 = local write "SO2 Zeroing / Calibration Abort"(FALSE) -> ()
            n988 = Bundle(cluster=T4 {"Message"="", "Message Data"=variant} ("Message Cluster"), "Message"="Auto_zero", "Message Data"=FALSE) -> (w2310:T4)
            n989 = Enqueue Element(queue=w2307, element=w2310, error in (no error)=w2306) -> ()  [unwired: 1 in, 3 out]
          }
        }
      }
    }
    n990 = Wait (ms)(milliseconds to wait=u32 100) -> ()  [unwired: 1 out]
  }
  n991 = while {
    tunnel: w4 -> [w2319]
    shift-right: [w2314] -> _
    shift-left: w43 -> [w2316]
    shift-right: [w2312] -> w41
    shift-left: w44 -> [w2318]
    tunnel: w3 -> [w2313]
    stop <- w2312 stop-if-true
    # "SO2 UI Command Sender"
    n992 = Dequeue Element(queue=w2319, error in (no error)=w2313) -> (element=w2315:T4)  [unwired: 1 in, 3 out]
    n993 = Unbundle By Name(w2315) -> ("Message"=w2317:string)
    n994 = case shown="\"zeroing_interval\"" w2317 {
      tunnel: w2318 -> [w2320 w2324 w2331 w2338 w2345 w2352 w2359 w2366 w2373 w2380 w2387 w2394 w2401 w2408 w2415 w2422 w2429 w2436 w2443 w2450 w2457 w2464 w2471 w2478 w2485 w2492]
      tunnel: w2316 -> [w2321 w2327 w2334 w2341 w2348 w2355 w2362 w2369 w2376 w2383 w2390 w2397 w2404 w2411 w2418 w2425 w2432 w2439 w2446 w2453 w2460 w2467 w2474 w2481 w2488 w2495]
      tunnel: w2315 -> [_ w2326 w2333 w2340 w2347 w2354 w2361 w2368 w2375 w2382 w2389 w2396 w2403 w2410 w2417 w2424 w2431 w2438 w2445 w2452 w2459 w2466 w2473 w2480 w2487 w2494]
      tunnel: [w2320 w2323 w2330 w2337 w2344 w2351 w2358 w2365 w2372 w2379 w2386 w2393 w2400 w2407 w2414 w2421 w2428 w2435 w2442 w2449 w2456 w2463 w2470 w2477 w2484 w2491] -> w2312
      tunnel: [w2321 w2322 w2329 w2336 w2343 w2350 w2357 w2364 w2371 w2378 w2385 w2392 w2399 w2406 w2413 w2420 w2427 w2434 w2441 w2448 w2455 w2462 w2469 w2476 w2483 w2490] -> w2314
      frame "False", Default {
      }
      frame "V9" {
        n995 = shared-variable-write(w2327, w2324, w2326) -> (w2325:refnum<k21>, w2328:errorcluster)  [unwired: 1 in, 1 out]
        n996 = Flush Stream(8:w2328, 11:w2325) -> (0:w2323:errorcluster, 3:w2322:refnum<k21>)  [unwired: 2 in, 1 out]
      }
      frame "MFC_2" {
        n997 = shared-variable-write(w2334, w2331, w2333) -> (w2332:refnum<k21>, w2335:errorcluster)  [unwired: 1 in, 1 out]
        n998 = Flush Stream(8:w2335, 11:w2332) -> (0:w2330:errorcluster, 3:w2329:refnum<k21>)  [unwired: 2 in, 1 out]
      }
      frame "MFC_3" {
        n999 = shared-variable-write(w2341, w2338, w2340) -> (w2339:refnum<k21>, w2342:errorcluster)  [unwired: 1 in, 1 out]
        n1000 = Flush Stream(8:w2342, 11:w2339) -> (0:w2337:errorcluster, 3:w2336:refnum<k21>)  [unwired: 2 in, 1 out]
      }
      frame "V6" {
        n1001 = shared-variable-write(w2348, w2345, w2347) -> (w2346:refnum<k21>, w2349:errorcluster)  [unwired: 1 in, 1 out]
        n1002 = Flush Stream(8:w2349, 11:w2346) -> (0:w2344:errorcluster, 3:w2343:refnum<k21>)  [unwired: 2 in, 1 out]
      }
      frame "Simulate Conc" {
        n1003 = shared-variable-write(w2355, w2352, w2354) -> (w2353:refnum<k21>, w2356:errorcluster)  [unwired: 1 in, 1 out]
        n1004 = Flush Stream(8:w2356, 11:w2353) -> (0:w2351:errorcluster, 3:w2350:refnum<k21>)  [unwired: 2 in, 1 out]
      }
      frame "Simulate STEL Conc" {
        n1005 = shared-variable-write(w2362, w2359, w2361) -> (w2360:refnum<k21>, w2363:errorcluster)  [unwired: 1 in, 1 out]
        n1006 = Flush Stream(8:w2363, 11:w2360) -> (0:w2358:errorcluster, 3:w2357:refnum<k21>)  [unwired: 2 in, 1 out]
      }
      frame "Simulate TWA Conc" {
        n1007 = shared-variable-write(w2369, w2366, w2368) -> (w2367:refnum<k21>, w2370:errorcluster)  [unwired: 1 in, 1 out]
        n1008 = Flush Stream(8:w2370, 11:w2367) -> (0:w2365:errorcluster, 3:w2364:refnum<k21>)  [unwired: 2 in, 1 out]
      }
      frame "10mins STEL Limit" {
        n1009 = shared-variable-write(w2376, w2373, w2375) -> (w2374:refnum<k21>, w2377:errorcluster)  [unwired: 1 in, 1 out]
        n1010 = Flush Stream(8:w2377, 11:w2374) -> (0:w2372:errorcluster, 3:w2371:refnum<k21>)  [unwired: 2 in, 1 out]
      }
      frame "8hr TWA Limit" {
        n1011 = shared-variable-write(w2383, w2380, w2382) -> (w2381:refnum<k21>, w2384:errorcluster)  [unwired: 1 in, 1 out]
        n1012 = Flush Stream(8:w2384, 11:w2381) -> (0:w2379:errorcluster, 3:w2378:refnum<k21>)  [unwired: 2 in, 1 out]
      }
      frame "Offset" {
        n1013 = shared-variable-write(w2390, w2387, w2389) -> (w2388:refnum<k21>, w2391:errorcluster)  [unwired: 1 in, 1 out]
        n1014 = Flush Stream(8:w2391, 11:w2388) -> (0:w2386:errorcluster, 3:w2385:refnum<k21>)  [unwired: 2 in, 1 out]
      }
      frame "eV8_user_set_time" {
        n1015 = shared-variable-write(w2397, w2394, w2396) -> (w2395:refnum<k21>, w2398:errorcluster)  [unwired: 1 in, 1 out]
        n1016 = Flush Stream(8:w2398, 11:w2395) -> (0:w2393:errorcluster, 3:w2392:refnum<k21>)  [unwired: 2 in, 1 out]
      }
      frame "mean_cal_status" {
        n1017 = shared-variable-write(w2404, w2401, w2403) -> (w2402:refnum<k21>, w2405:errorcluster)  [unwired: 1 in, 1 out]
        n1018 = Flush Stream(8:w2405, 11:w2402) -> (0:w2400:errorcluster, 3:w2399:refnum<k21>)  [unwired: 2 in, 1 out]
      }
      frame "SO2_MOCCA_Alarm" {
        n1019 = shared-variable-write(w2411, w2408, w2410) -> (w2409:refnum<k21>, w2412:errorcluster)  [unwired: 1 in, 1 out]
        n1020 = Flush Stream(8:w2412, 11:w2409) -> (0:w2407:errorcluster, 3:w2406:refnum<k21>)  [unwired: 2 in, 1 out]
      }
      frame "MOCCA_window_delay_time" {
        n1021 = shared-variable-write(w2418, w2415, w2417) -> (w2416:refnum<k21>, w2419:errorcluster)  [unwired: 1 in, 1 out]
        n1022 = Flush Stream(8:w2419, 11:w2416) -> (0:w2414:errorcluster, 3:w2413:refnum<k21>)  [unwired: 2 in, 1 out]
      }
      frame "MOCCA_limit" {
        n1023 = shared-variable-write(w2425, w2422, w2424) -> (w2423:refnum<k21>, w2426:errorcluster)  [unwired: 1 in, 1 out]
        n1024 = Flush Stream(8:w2426, 11:w2423) -> (0:w2421:errorcluster, 3:w2420:refnum<k21>)  [unwired: 2 in, 1 out]
      }
      frame "calcon_save" {
        n1025 = shared-variable-write(w2432, w2429, w2431) -> (w2430:refnum<k21>, w2433:errorcluster)  [unwired: 1 in, 1 out]
        n1026 = Flush Stream(8:w2433, 11:w2430) -> (0:w2428:errorcluster, 3:w2427:refnum<k21>)  [unwired: 2 in, 1 out]
      }
      frame "Auto_zero" {
        n1027 = shared-variable-write(w2439, w2436, w2438) -> (w2437:refnum<k21>, w2440:errorcluster)  [unwired: 1 in, 1 out]
        n1028 = Flush Stream(8:w2440, 11:w2437) -> (0:w2435:errorcluster, 3:w2434:refnum<k21>)  [unwired: 2 in, 1 out]
      }
      frame "zeroing_interval" {
        n1029 = shared-variable-write(w2446, w2443, w2445) -> (w2444:refnum<k21>, w2447:errorcluster)  [unwired: 1 in, 1 out]
        n1030 = Flush Stream(8:w2447, 11:w2444) -> (0:w2442:errorcluster, 3:w2441:refnum<k21>)  [unwired: 2 in, 1 out]
      }
      frame "cal_gas_cylin_conc" {
        n1031 = shared-variable-write(w2453, w2450, w2452) -> (w2451:refnum<k21>, w2454:errorcluster)  [unwired: 1 in, 1 out]
        n1032 = Flush Stream(8:w2454, 11:w2451) -> (0:w2449:errorcluster, 3:w2448:refnum<k21>)  [unwired: 2 in, 1 out]
      }
      frame "sim_MOCCA_conc" {
        n1033 = shared-variable-write(w2460, w2457, w2459) -> (w2458:refnum<k21>, w2461:errorcluster)  [unwired: 1 in, 1 out]
        n1034 = Flush Stream(8:w2461, 11:w2458) -> (0:w2456:errorcluster, 3:w2455:refnum<k21>)  [unwired: 2 in, 1 out]
      }
      frame "Slope" {
        n1035 = shared-variable-write(w2467, w2464, w2466) -> (w2465:refnum<k21>, w2468:errorcluster)  [unwired: 1 in, 1 out]
        n1036 = Flush Stream(8:w2468, 11:w2465) -> (0:w2463:errorcluster, 3:w2462:refnum<k21>)  [unwired: 2 in, 1 out]
      }
      frame "Flight Number" {
        n1037 = shared-variable-write(w2474, w2471, w2473) -> (w2472:refnum<k21>, w2475:errorcluster)  [unwired: 1 in, 1 out]
        n1038 = Flush Stream(8:w2475, 11:w2472) -> (0:w2470:errorcluster, 3:w2469:refnum<k21>)  [unwired: 2 in, 1 out]
      }
      frame "Stop File Write" {
        n1039 = shared-variable-write(w2481, w2478, w2480) -> (w2479:refnum<k21>, w2482:errorcluster)  [unwired: 1 in, 1 out]
        n1040 = Flush Stream(8:w2482, 11:w2479) -> (0:w2477:errorcluster, 3:w2476:refnum<k21>)  [unwired: 2 in, 1 out]
      }
      frame "UDP Time Offset" {
        n1041 = shared-variable-write(w2488, w2485, w2487) -> (w2486:refnum<k21>, w2489:errorcluster)  [unwired: 1 in, 1 out]
        n1042 = Flush Stream(8:w2489, 11:w2486) -> (0:w2484:errorcluster, 3:w2483:refnum<k21>)  [unwired: 2 in, 1 out]
      }
      frame "V8" {
        n1043 = shared-variable-write(w2495, w2492, w2494) -> (w2493:refnum<k21>, w2496:errorcluster)  [unwired: 1 in, 1 out]
        n1044 = Flush Stream(8:w2496, 11:w2493) -> (0:w2491:errorcluster, 3:w2490:refnum<k21>)  [unwired: 2 in, 1 out]
      }
    }
  }
  "SO2 command sender \nerror out" <- w41
  n1045 = Obtain Queue(name (unnamed)="TEi43c_Command", element data type=w29) -> (queue out=w38:refnum<queue>, error out=w31:errorcluster)  [unwired: 3 in, 1 out]
  n1046 = Create Network Stream Writer Endpoint(6:w35, 7:10 ("writer buffer size"), 9:w29, 10:"//192.168.101.17/command/reader/TEi43c" ("reader url"), 11:"/command/writer/TEi43c" ("writer name")) -> (0:w34:errorcluster, 3:w33:refnum<k21>)  [unwired: 2 in]
  n1047 = while {
    tunnel: w38 -> [w2500]
    tunnel: w31 -> [w2499]
    tunnel: [w2497] -> _
    stop <- FALSE stop-if-true
    # "TEi43c Ozone UI Event Handler Loop"
    n1048 = event shown="[0] \"Ozone Zeroing\": Value Change" {
      selector: _ -> [_ _ _ _ _]
      dyn-events: _ -> [_ _ _ _ _]
      timeout: _ -> [_ _ _ _ _]
      tunnel: w2500 -> [w2508 w2546 w2554 w2561 w2569]
      tunnel: w2499 -> [w2507 w2545 w2553 w2560 w2568]
      tunnel: [w2506 w2544 w2552 w2559 w2567] -> w2497
      event "Ozone Zeroing": Value Change {
        n1049 = event-data() -> ()  [unwired: 1 in, 6 out]
        n1050 = flat-sequence {
          tunnel: w2508 -> [w2513]
          tunnel: w2507 -> [w2512]
          tunnel: [w2511] -> w2505
          tunnel: [w2509] -> w2501
          tunnel: w2505 -> [w2519]
          tunnel: [w2519] -> w2504
          tunnel: [w2517] -> w2502
          tunnel: w2501 -> [w2517]
          tunnel: w2504 -> [w2537]
          tunnel: [w2536] -> w2503
          tunnel: w2502 -> [w2538]
          tunnel: [w2543] -> w2506
          tunnel: w2503 -> [w2543]
          frame #0 {
            w2510 = TRUE
            n1051 = local write "Ozone eV6"(w2510) -> ()
            n1052 = Bundle(cluster=T4 {"Message"="", "Message Data"=variant} ("Message Cluster"), "Message"="V6", "Message Data"=w2510) -> (w2514:T4)
            n1053 = Enqueue Element(queue=w2513, element=w2514, error in (no error)=w2512) -> (queue out=w2509:refnum<queue>, error out=w2511:errorcluster)  [unwired: 1 in, 1 out]
          }
          frame #1 {
            # "10 Mins Count down"
            n1054 = for {
              N: 600 -> [w2529]
              i -> [w2528]
              stop <- w2521 stop-if-true
              n1055 = local read "Ozone Zeroing Abort"() -> (w2523:bool)
              n1056 = Subtract(x=w2529, y=w2528) -> (x-y=w2527:i32)
              n1057 = Decrement(x=w2527) -> (x-1=w2525:i32)
              n1058 = Wait (ms)(milliseconds to wait=u32 1000) -> ()  [unwired: 1 out]
              n1059 = case shown="True" w2523 {
                selector: w2523 -> [w2532 _]
                tunnel: [w2532 w2533] -> w2520
                frame False {
                }
                frame True {
                  n1060 = Two Button Dialog(message="Are you sure to abort Ozone Zeroing?") -> (T button?=w2533:bool)  [unwired: 2 in]
                }
              }
              n1061 = local read "Network disconnected"() -> (w2522:bool)
              n1062 = Or(x=w2522, y=w2520) -> (x .or. y?=w2521:bool)
              n1063 = Select(t=0, s=w2521, f=w2525) -> (s? t:f=→"Ozone Zeroing\nTime Remain (sec)":i32)
              n1064 = case shown="False" w2520 {
                selector: w2520 -> [w2531 _]
                frame False {
                  n1065 = local write "Ozone Zeroing Abort"(w2531) -> ()
                }
                frame True {
                }
              }
            }
          }
          frame #2 {
            w2535 = FALSE
            n1066 = local write "Ozone eV6"(w2535) -> ()
            n1067 = Bundle(cluster=T4 {"Message"="", "Message Data"=variant} ("Message Cluster"), "Message"="V6", "Message Data"=w2535) -> (w2539:T4)
            n1068 = Enqueue Element(queue=w2538, element=w2539, error in (no error)=w2537) -> (error out=w2536:errorcluster)  [unwired: 1 in, 2 out]
          }
          frame #3 {
            w2542 = FALSE ("Ozone Zeroing")
            n1069 = local write "Ozone Zeroing Abort"(w2542) -> ()
            n1070 = local write "Ozone Zeroing"(w2542) -> ()
          }
        }
      }
      event "Ozone eV6": Value Change {
        n1071 = event-data() -> ("NewVal"=w2547:bool)  [unwired: 1 in]
        n1072 = Bundle(cluster=T4 {"Message"="", "Message Data"=variant} ("Message Cluster"), "Message"="V6", "Message Data"=w2547) -> (w2548:T4)
        n1073 = Enqueue Element(queue=w2546, element=w2548, error in (no error)=w2545) -> (error out=w2544:errorcluster)  [unwired: 1 in, 2 out]
      }
      event "cRIO File IO Stop\n(USB Flash Drive Unmount)": Value Change {
        n1074 = event-data() -> ("NewVal"=w2551:bool)  [unwired: 1 in]
        n1075 = Bundle(cluster=T4 {"Message"="", "Message Data"=variant} ("Message Cluster"), "Message"="Stop File Write", "Message Data"=w2551) -> (w2555:T4)
        n1076 = Enqueue Element(queue=w2554, element=w2555, error in (no error)=w2553) -> (error out=w2552:errorcluster)  [unwired: 1 in, 2 out]
      }
      event "Ozone UDP Time Offset": Value Change {
        n1077 = event-data() -> ("NewVal"=w2558:i32)  [unwired: 1 in]
        n1078 = Bundle(cluster=T4 {"Message"="", "Message Data"=variant} ("Message Cluster"), "Message"="UDP Time Offset", "Message Data"=w2558) -> (w2562:T4)
        n1079 = Enqueue Element(queue=w2561, element=w2562, error in (no error)=w2560) -> (error out=w2559:errorcluster)  [unwired: 1 in, 2 out]
      }
      event "Confirm Flight Number": Value Change {
        n1080 = event-data() -> ()  [unwired: 1 in, 5 out]
        n1081 = flat-sequence {
          tunnel: w2568 -> [w2571]
          tunnel: w2569 -> [w2572]
          tunnel: [w2572] -> w2566
          tunnel: [w2571] -> w2565
          tunnel: [w2574] -> w2567
          tunnel: w2566 -> [w2576]
          tunnel: w2565 -> [w2575]
          frame #0 {
            n1082 = local write "cRIO File IO Stop\n(USB Flash Drive Unmount)"(FALSE ("cRIO File IO Stop\n(USB Flash Drive Unmount)")) -> ()
          }
          frame #1 {
            n1083 = local read "Flight Number"() -> (w2573:string)
            n1084 = Bundle(cluster=T4 {"Message"="", "Message Data"=variant} ("Message Cluster"), "Message"="Flight Number", "Message Data"=w2573) -> (w2577:T4)
            n1085 = Enqueue Element(queue=w2576, element=w2577, error in (no error)=w2575) -> (error out=w2574:errorcluster)  [unwired: 1 in, 2 out]
          }
        }
      }
    }
    "Ozone Event error out" <- w2497
  }
  n1086 = while {
    tunnel: w38 -> [w2587]
    shift-right: [w2582] -> _
    shift-left: w33 -> [w2584]
    shift-right: [w2580] -> w30
    shift-left: w34 -> [w2586]
    tunnel: w31 -> [w2581]
    stop <- w2580 stop-if-true
    # "TEi43c Ozone UI Command Sender"
    n1087 = Dequeue Element(queue=w2587, error in (no error)=w2581) -> (element=w2583:T4)  [unwired: 1 in, 3 out]
    n1088 = Unbundle By Name(w2583) -> ("Message"=w2585:string)
    n1089 = case shown="\"UDP Time Offset\"" w2585 {
      tunnel: w2586 -> [w2588 w2592 w2599 w2606 w2613]
      tunnel: w2584 -> [w2589 w2595 w2602 w2609 w2616]
      tunnel: w2583 -> [_ w2594 w2601 w2608 w2615]
      tunnel: [w2588 w2591 w2598 w2605 w2612] -> w2580
      tunnel: [w2589 w2590 w2597 w2604 w2611] -> w2582
      frame "False", Default {
      }
      frame "V6" {
        n1090 = shared-variable-write(w2595, w2592, w2594) -> (w2593:refnum<k21>, w2596:errorcluster)  [unwired: 1 in, 1 out]
        n1091 = Flush Stream(8:w2596, 11:w2593) -> (0:w2591:errorcluster, 3:w2590:refnum<k21>)  [unwired: 2 in, 1 out]
      }
      frame "Stop File Write" {
        n1092 = shared-variable-write(w2602, w2599, w2601) -> (w2600:refnum<k21>, w2603:errorcluster)  [unwired: 1 in, 1 out]
        n1093 = Flush Stream(8:w2603, 11:w2600) -> (0:w2598:errorcluster, 3:w2597:refnum<k21>)  [unwired: 2 in, 1 out]
      }
      frame "Flight Number" {
        n1094 = shared-variable-write(w2609, w2606, w2608) -> (w2607:refnum<k21>, w2610:errorcluster)  [unwired: 1 in, 1 out]
        n1095 = Flush Stream(8:w2610, 11:w2607) -> (0:w2605:errorcluster, 3:w2604:refnum<k21>)  [unwired: 2 in, 1 out]
      }
      frame "UDP Time Offset" {
        n1096 = shared-variable-write(w2616, w2613, w2615) -> (w2614:refnum<k21>, w2617:errorcluster)  [unwired: 1 in, 1 out]
        n1097 = Flush Stream(8:w2617, 11:w2614) -> (0:w2612:errorcluster, 3:w2611:refnum<k21>)  [unwired: 2 in, 1 out]
      }
    }
  }
  "Ozone command sender error out" <- w30
  n1098 = Obtain Queue(name (unnamed)="2BOzone_Command", element data type=w17) -> (queue out=w26:refnum<queue>, error out=w19:errorcluster)  [unwired: 3 in, 1 out]
  n1099 = Create Network Stream Writer Endpoint(6:w23, 7:10 ("writer buffer size"), 9:w17, 10:"//192.168.101.17/command/reader/2BOzone" ("reader url"), 11:"/command/writer/2BOzone" ("writer name")) -> (0:w22:errorcluster, 3:w21:refnum<k21>)  [unwired: 2 in]
  n1100 = while {
    tunnel: w26 -> [w2621]
    tunnel: w19 -> [w2620]
    tunnel: [w2618] -> _
    stop <- FALSE stop-if-true
    # "2BOzone UI Event Handler Loop"
    n1101 = event shown="[2] \"Simulate Inst Conc\": Value Change" {
      selector: _ -> [_ _ _ _ _ _ _ _]
      dyn-events: _ -> [_ _ _ _ _ _ _ _]
      timeout: _ -> [_ _ _ _ _ _ _ _]
      tunnel: w2621 -> [w2625 w2632 w2639 w2646 w2653 w2660 w2667 w2675]
      tunnel: w2620 -> [w2624 w2631 w2638 w2645 w2652 w2659 w2666 w2674]
      tunnel: [w2623 w2630 w2637 w2644 w2651 w2658 w2665 w2673] -> w2618
      event "Ambient = OFF\nCabin = ON": Value Change {
        n1102 = event-data() -> ("NewVal"=w2622:bool)  [unwired: 1 in]
        n1103 = Bundle(cluster=T4 {"Message"="", "Message Data"=variant} ("Message Cluster"), "Message"="Ambient/Cabin", "Message Data"=w2622) -> (w2626:T4)
        n1104 = Enqueue Element(queue=w2625, element=w2626, error in (no error)=w2624) -> (error out=w2623:errorcluster)  [unwired: 1 in, 2 out]
      }
      event "Simulate 2B Conc": Value Change {
        n1105 = event-data() -> ("NewVal"=w2629:bool)  [unwired: 1 in]
        n1106 = Bundle(cluster=T4 {"Message"="", "Message Data"=variant} ("Message Cluster"), "Message"="Simulate_conc", "Message Data"=w2629) -> (w2633:T4)
        n1107 = Enqueue Element(queue=w2632, element=w2633, error in (no error)=w2631) -> (error out=w2630:errorcluster)  [unwired: 1 in, 2 out]
      }
      event "Simulate Inst Conc": Value Change {
        n1108 = event-data() -> ("NewVal"=w2636:i32)  [unwired: 1 in]
        n1109 = Bundle(cluster=T4 {"Message"="", "Message Data"=variant} ("Message Cluster"), "Message"="Simulate_inst_conc", "Message Data"=w2636) -> (w2640:T4)
        n1110 = Enqueue Element(queue=w2639, element=w2640, error in (no error)=w2638) -> (error out=w2637:errorcluster)  [unwired: 1 in, 2 out]
      }
      event "Inst_alm_thresh": Value Change {
        n1111 = event-data() -> ("NewVal"=w2643:i32)  [unwired: 1 in]
        n1112 = Bundle(cluster=T4 {"Message"="", "Message Data"=variant} ("Message Cluster"), "Message"="Inst_alm_thresh", "Message Data"=w2643) -> (w2647:T4)
        n1113 = Enqueue Element(queue=w2646, element=w2647, error in (no error)=w2645) -> (error out=w2644:errorcluster)  [unwired: 1 in, 2 out]
      }
      event "3hr_alm_thresh": Value Change {
        n1114 = event-data() -> ("NewVal"=w2650:i32)  [unwired: 1 in]
        n1115 = Bundle(cluster=T4 {"Message"="", "Message Data"=variant} ("Message Cluster"), "Message"="3hr_alm_thresh", "Message Data"=w2650) -> (w2654:T4)
        n1116 = Enqueue Element(queue=w2653, element=w2654, error in (no error)=w2652) -> (error out=w2651:errorcluster)  [unwired: 1 in, 2 out]
      }
      event "Simulate 3hr Average Conc": Value Change {
        n1117 = event-data() -> ("NewVal"=w2657:dbl)  [unwired: 1 in]
        n1118 = Bundle(cluster=T4 {"Message"="", "Message Data"=variant} ("Message Cluster"), "Message"="Simulate_3hr_av_conc", "Message Data"=w2657) -> (w2661:T4)
        n1119 = Enqueue Element(queue=w2660, element=w2661, error in (no error)=w2659) -> (error out=w2658:errorcluster)  [unwired: 1 in, 2 out]
      }
      event "cRIO File IO Stop\n(USB Flash Drive Unmount)": Value Change {
        n1120 = event-data() -> ("NewVal"=w2664:bool)  [unwired: 1 in]
        n1121 = Bundle(cluster=T4 {"Message"="", "Message Data"=variant} ("Message Cluster"), "Message"="Stop File Write", "Message Data"=w2664) -> (w2668:T4)
        n1122 = Enqueue Element(queue=w2667, element=w2668, error in (no error)=w2666) -> (error out=w2665:errorcluster)  [unwired: 1 in, 2 out]
      }
      event "Confirm Flight Number": Value Change {
        n1123 = event-data() -> ()  [unwired: 1 in, 5 out]
        n1124 = flat-sequence {
          tunnel: w2674 -> [w2677]
          tunnel: w2675 -> [w2678]
          tunnel: [w2678] -> w2672
          tunnel: [w2677] -> w2671
          tunnel: [w2680] -> w2673
          tunnel: w2672 -> [w2682]
          tunnel: w2671 -> [w2681]
          frame #0 {
            n1125 = local write "cRIO File IO Stop\n(USB Flash Drive Unmount)"(FALSE ("cRIO File IO Stop\n(USB Flash Drive Unmount)")) -> ()
          }
          frame #1 {
            n1126 = local read "Flight Number"() -> (w2679:string)
            n1127 = Bundle(cluster=T4 {"Message"="", "Message Data"=variant} ("Message Cluster"), "Message"="Flight Number", "Message Data"=w2679) -> (w2683:T4)
            n1128 = Enqueue Element(queue=w2682, element=w2683, error in (no error)=w2681) -> (error out=w2680:errorcluster)  [unwired: 1 in, 2 out]
          }
        }
      }
    }
    "2BOzone Event error out" <- w2618
  }
  n1129 = while {
    tunnel: w26 -> [w2693]
    shift-right: [w2688] -> _
    shift-left: w21 -> [w2690]
    shift-right: [w2686] -> w18
    shift-left: w22 -> [w2692]
    tunnel: w19 -> [w2687]
    stop <- w2686 stop-if-true
    # "2BOzone UI Command Sender"
    n1130 = Dequeue Element(queue=w2693, error in (no error)=w2687) -> (element=w2689:T4)  [unwired: 1 in, 3 out]
    n1131 = Unbundle By Name(w2689) -> ("Message"=w2691:string)
    n1132 = case shown="\"3hr_alm_thresh\"" w2691 {
      tunnel: w2692 -> [w2694 w2698 w2705 w2712 w2719 w2726 w2733 w2740 w2747]
      tunnel: w2690 -> [w2695 w2701 w2708 w2715 w2722 w2729 w2736 w2743 w2750]
      tunnel: w2689 -> [_ w2700 w2707 w2714 w2721 w2728 w2735 w2742 w2749]
      tunnel: [w2694 w2697 w2704 w2711 w2718 w2725 w2732 w2739 w2746] -> w2686
      tunnel: [w2695 w2696 w2703 w2710 w2717 w2724 w2731 w2738 w2745] -> w2688
      frame "False", Default {
      }
      frame "Ambient/Cabin" {
        n1133 = shared-variable-write(w2701, w2698, w2700) -> (w2699:refnum<k21>, w2702:errorcluster)  [unwired: 1 in, 1 out]
        n1134 = Flush Stream(8:w2702, 11:w2699) -> (0:w2697:errorcluster, 3:w2696:refnum<k21>)  [unwired: 2 in, 1 out]
      }
      frame "Simulate_conc" {
        n1135 = shared-variable-write(w2708, w2705, w2707) -> (w2706:refnum<k21>, w2709:errorcluster)  [unwired: 1 in, 1 out]
        n1136 = Flush Stream(8:w2709, 11:w2706) -> (0:w2704:errorcluster, 3:w2703:refnum<k21>)  [unwired: 2 in, 1 out]
      }
      frame "Simulate_inst_conc" {
        n1137 = shared-variable-write(w2715, w2712, w2714) -> (w2713:refnum<k21>, w2716:errorcluster)  [unwired: 1 in, 1 out]
        n1138 = Flush Stream(8:w2716, 11:w2713) -> (0:w2711:errorcluster, 3:w2710:refnum<k21>)  [unwired: 2 in, 1 out]
      }
      frame "Inst_alm_thresh" {
        n1139 = shared-variable-write(w2722, w2719, w2721) -> (w2720:refnum<k21>, w2723:errorcluster)  [unwired: 1 in, 1 out]
        n1140 = Flush Stream(8:w2723, 11:w2720) -> (0:w2718:errorcluster, 3:w2717:refnum<k21>)  [unwired: 2 in, 1 out]
      }
      frame "3hr_alm_thresh" {
        n1141 = shared-variable-write(w2729, w2726, w2728) -> (w2727:refnum<k21>, w2730:errorcluster)  [unwired: 1 in, 1 out]
        n1142 = Flush Stream(8:w2730, 11:w2727) -> (0:w2725:errorcluster, 3:w2724:refnum<k21>)  [unwired: 2 in, 1 out]
      }
      frame "Simulate_3hr_av_conc" {
        n1143 = shared-variable-write(w2736, w2733, w2735) -> (w2734:refnum<k21>, w2737:errorcluster)  [unwired: 1 in, 1 out]
        n1144 = Flush Stream(8:w2737, 11:w2734) -> (0:w2732:errorcluster, 3:w2731:refnum<k21>)  [unwired: 2 in, 1 out]
      }
      frame "Stop File Write" {
        n1145 = shared-variable-write(w2743, w2740, w2742) -> (w2741:refnum<k21>, w2744:errorcluster)  [unwired: 1 in, 1 out]
        n1146 = Flush Stream(8:w2744, 11:w2741) -> (0:w2739:errorcluster, 3:w2738:refnum<k21>)  [unwired: 2 in, 1 out]
      }
      frame "Flight Number" {
        n1147 = shared-variable-write(w2750, w2747, w2749) -> (w2748:refnum<k21>, w2751:errorcluster)  [unwired: 1 in, 1 out]
        n1148 = Flush Stream(8:w2751, 11:w2748) -> (0:w2746:errorcluster, 3:w2745:refnum<k21>)  [unwired: 2 in, 1 out]
      }
    }
  }
  "2BOzone command sender error out" <- w18
